vi "TC.vi"() -> ()   [LabVIEW 2013]
uses:
  lib/Lib.llb/CS.lvclass
  lib/Lib.llb/TCS.lvclass
  lib/Lib.llb/QCS.lvclass
  lib/Lib.llb/CS Emulation.lvclass
  lib/Lib.llb/PCS.lvclass
panel:
  out "Name":string
  out "SetControl":T1
  out "ControlNames":string[](array[string])
  out "VIRef":T2 {"Array DataType" format="%.0x"; "WaveForm Type" format="%.0x"; "RefNum Type" format="%.0x"; "DataType" format="%.0x"}
  out "Scan Parameters":cluster{string, "Freq":dbl, "V_exc":dbl}
  out "zConfig":path=path "C:/Users/Sasha/Dropbox/Labview/LC Software/ImpSoft-V5.2.2-multithreaded/ImpBridgeLabview/ImpBridgeDll.dll"
  out "TempStabilized":refnum<user-event>
  out "Actual I":dbl[](array[numeric])
  out "VI called?":bool=TRUE
  out "Error code":u8
  out "UpdateChannelInfo":refnum<user-event>
  out "zBridge set nr.":u8
  out "zDll":path=path "C:/Users/Sasha/Dropbox/Labview/LC Software/ImpSoft-V5.2.2-multithreaded/ImpBridgeLabview/ImpBridgeDll.dll"
  in  "String":string="^ Click the Run button to start the program "
  in  "Toolbar":enum32{"Page 1", "Page 2"}(tab)
  in  "Load config":bool
  in  "Start":bool
  in  "Load Data":bool
  in  "Pause":bool
  in  "Stop":bool
  in  "Copy to Clipboard":bool
  in  "Save to Cal Log":bool
  in  "Save config":bool
  in  "Save Data":bool
  in  "Clear all plots":bool
  in  "ColorBox":enum32{"Page 1", "Page 2"}(tab)
  in  "Colors":picture
  out "Color":u32(colorbox)
  in  "LogFileCreationTime":timestamp=timestamp(2742897600 s since 1904-01-01)
  out "UpdateLogFilePath":refnum<user-event>
  out "Calib path":path=path "C:/avs-47/aaaa"
  out "Log path":path
  out "TCS port":i32(ring)=3 items=["COM1", "COM2", "COM3", "COM4", "COM5", "COM6", "COM7", "COM8", "COM9", "PRN1", "PRN2", "PRN3", "PRN4"]
  out "UpdateCalibrations":refnum<user-event>
  out "AVS VISA session":refnum<visa-resource-name>="COM3"
  in  "Minimize 2":bool
  out "Revision":string="TC" caption="V"
  in  "Minimize":bool
  out "Current1flow":bool
  out "Current2flow":bool
  in  "Tab Control":enum32{"AVS"}(tab)
  in  "Channel Controls":T3(tab)=enum."All"
  out "T0":dbl=nan caption="T" format="%#.2p"
  out "R0":dbl caption="R" format="%.3p"
  out "R-Plot 0":cluster{dbl[], dbl[]}(graph) caption="R-Plot"
  out "T1":dbl=nan caption="T" format="%#.2p"
  out "R1":dbl caption="R" format="%.3p"
  out "R-Plot 1":cluster{dbl[], dbl[]}(graph) caption="R-Plot"
  out "T2":dbl=nan caption="T" format="%#.2p"
  out "R2":dbl caption="R" format="%.3p"
  out "R-Plot 2":cluster{dbl[], dbl[]}(graph) caption="R-Plot"
  out "T3":dbl=nan caption="T" format="%#.2p"
  out "R3":dbl caption="R" format="%.3p"
  out "R-Plot 3":cluster{dbl[], dbl[]}(graph) caption="R-Plot"
  out "T4":dbl=nan caption="T" format="%#.2p"
  out "R4":dbl caption="R" format="%.3p"
  out "R-Plot 4":cluster{dbl[], dbl[]}(graph) caption="R-Plot"
  out "T5":dbl=nan caption="T" format="%#.2p"
  out "R5":dbl caption="R" format="%.3p"
  out "R-Plot 5":cluster{dbl[], dbl[]}(graph) caption="R-Plot"
  out "T6":dbl=nan caption="T" format="%#.2p"
  out "R6":dbl caption="R" format="%.3p"
  out "R-Plot 6":cluster{dbl[], dbl[]}(graph) caption="R-Plot"
  out "T7":dbl=nan caption="T" format="%#.2p"
  out "R7":dbl caption="R" format="%.3p"
  out "R-Plot 7":cluster{dbl[], dbl[]}(graph) caption="R-Plot"
  out "T8":dbl=nan caption="T" format="%#.2p"
  out "R8":dbl caption="R" format="%.3p"
  out "R-Plot 8":cluster{dbl[], dbl[]}(graph) caption="R-Plot"
  out "T9":dbl=nan caption="T" format="%#.2p"
  out "R9":dbl caption="R" format="%.3p"
  out "R-Plot 9":cluster{dbl[], dbl[]}(graph) caption="R-Plot"
  out "T":T4 {"T0 3" format="%.2p"; "T0 2" format="%.2p"; "T0" format="%.2p"; "T0" format="%.2p"; "T0" format="%.2p"; "T0" format="%.2p"; "T0" format="%.2p"; "T0" format="%.2p"; "T0" format="%.2p"; "T0" format="%.2p"}
  in  "AVS names":T5={"AVS Name 0"="3K", "AVS Name 1"="Still", "AVS Name 2"="50 mK", "AVS Name 3"="MC", "AVS Name 4"="MC", "AVS Name 5"="", "AVS Name 6"="", "AVS Name 7"="", "AVS Name 8"="", "AVS Name 9"=""}
  in  "Edit Calibrations":T6
  in  "Thermometer":T7 {"Select sensor 10" items=["No Calibration", "PT100", "PT1000", "RuO2 10k", "RuO2 1k5", "RuO2 2k", "Emulation R", "PT 1000", "RuO2-10K-NEW", "testCMN", "No Calibration"]; "Select sensor 9" items=["No Calibration", "PT100", "PT1000", "RuO2 10k", "RuO2 1k5", "RuO2 2k", "Emulation R", "PT 1000", "RuO2-10K-NEW", "testCMN", "No Calibration"]; "Select sensor 8" items=["No Calibration", "PT100", "PT1000", "RuO2 10k", "RuO2 1k5", "RuO2 2k", "Emulation R", "PT 1000", "RuO2-10K-NEW", "testCMN", "No Calibration"]; "Select sensor 7" items=["No Calibration", "PT100", "PT1000", "RuO2 10k", "RuO2 1k5", "RuO2 2k", "Emulation R", "PT 1000", "RuO2-10K-NEW", "testCMN", "No Calibration"]; "Select sensor 6" items=["No Calibration", "PT100", "PT1000", "RuO2 10k", "RuO2 1k5", "RuO2 2k", "Emulation R", "PT 1000", "RuO2-10K-NEW", "testCMN", "No Calibration"]; "Select sensor 5" items=["No Calibration", "PT100", "PT1000", "RuO2 10k", "RuO2 1k5", "RuO2 2k", "Emulation R", "PT 1000", "RuO2-10K-NEW", "testCMN", "No Calibration"]; "Select sensor 4" items=["No Calibration", "PT100", "PT1000", "RuO2 10k", "RuO2 1k5", "RuO2 2k", "Emulation R", "PT 1000", "RuO2-10K-NEW", "testCMN", "No Calibration"]; "Select sensor 3" items=["No Calibration", "PT100", "PT1000", "RuO2 10k", "RuO2 1k5", "RuO2 2k", "Emulation R", "PT 1000", "RuO2-10K-NEW", "testCMN", "No Calibration"]; "Select sensor 2" items=["No Calibration", "PT100", "PT1000", "RuO2 10k", "RuO2 1k5", "RuO2 2k", "Emulation R", "PT 1000", "RuO2-10K-NEW", "testCMN", "No Calibration"]; "Select sensor 1" items=["No Calibration", "PT100", "PT1000", "RuO2 10k", "RuO2 1k5", "RuO2 2k", "Emulation R", "PT 1000", "RuO2-10K-NEW", "testCMN", "No Calibration"]}
  out "Units":T5
  out "R":T8={"R0"=0.0, "R1"=0.0, "R2"=-0.0, "R3"=0.0, "R4"=0.0, "R5"=0.0, "R6"=0.0, "R7"=0.0, "R6 2"=0.0, "R7 2"=0.0} {"R7 2" format="%.3p"; "R6 2" format="%.3p"; "R7" format="%.3p"; "R6" format="%.3p"; "R5" format="%.3p"; "R4" format="%.3p"; "R3" format="%.3p"; "R2" format="%.3p"; "R1" format="%.3p"; "R0" format="%.3p"}
  in  "Scan Parameters":enum32{"Page 1", "Page 2"}(tab)
  in  "Exc&Ranges":T9={"Excitationl 0"=4, "Excitationl 0"=4, "Excitationl 0"=3, "Excitationl 0"=3, "Excitationl 0"=3, "Excitationl 0"=3, "Excitationl 0"=3, "Excitationl 0"=3, "Range 0"=5, "Range 0"=5, "Range 0"=5, "Range 0"=5, "Range 0"=5, "Range 0"=5, "Range 0"=5, "Range 0"=5} {"Range 0" items=["n.a."=-1, "open"=0, "2 Ohm"=1, "20 Ohm"=2, "200 Ohm"=3, "2k Ohm"=4, "20k Ohm"=5, "200k Ohm"=6, "2M Ohm"=7]; "Range 0" items=["n.a."=-1, "open"=0, "2 Ohm"=1, "20 Ohm"=2, "200 Ohm"=3, "2k Ohm"=4, "20k Ohm"=5, "200k Ohm"=6, "2M Ohm"=7]; "Range 0" items=["n.a."=-1, "open"=0, "2 Ohm"=1, "20 Ohm"=2, "200 Ohm"=3, "2k Ohm"=4, "20k Ohm"=5, "200k Ohm"=6, "2M Ohm"=7]; "Range 0" items=["n.a."=-1, "open"=0, "2 Ohm"=1, "20 Ohm"=2, "200 Ohm"=3, "2k Ohm"=4, "20k Ohm"=5, "200k Ohm"=6, "2M Ohm"=7]; "Range 0" items=["n.a."=-1, "open"=0, "2 Ohm"=1, "20 Ohm"=2, "200 Ohm"=3, "2k Ohm"=4, "20k Ohm"=5, "200k Ohm"=6, "2M Ohm"=7]; "Range 0" items=["n.a."=-1, "open"=0, "2 Ohm"=1, "20 Ohm"=2, "200 Ohm"=3, "2k Ohm"=4, "20k Ohm"=5, "200k Ohm"=6, "2M Ohm"=7]; "Range 0" items=["n.a."=-1, "open"=0, "2 Ohm"=1, "20 Ohm"=2, "200 Ohm"=3, "2k Ohm"=4, "20k Ohm"=5, "200k Ohm"=6, "2M Ohm"=7]; "Range 0" items=["n.a."=-1, "open"=0, "2 Ohm"=1, "20 Ohm"=2, "200 Ohm"=3, "2k Ohm"=4, "20k Ohm"=5, "200k Ohm"=6, "2M Ohm"=7]; "Excitationl 0" items=["none", "3 µV", "10 µV", "30 µV", "100 µV", "300 µV", "1 mV", "3 mV"]; "Excitationl 0" items=["none", "3 µV", "10 µV", "30 µV", "100 µV", "300 µV", "1 mV", "3 mV"]; "Excitationl 0" items=["none", "3 µV", "10 µV", "30 µV", "100 µV", "300 µV", "1 mV", "3 mV"]; "Excitationl 0" items=["none", "3 µV", "10 µV", "30 µV", "100 µV", "300 µV", "1 mV", "3 mV"]; "Excitationl 0" items=["none", "3 µV", "10 µV", "30 µV", "100 µV", "300 µV", "1 mV", "3 mV"]; "Excitationl 0" items=["none", "3 µV", "10 µV", "30 µV", "100 µV", "300 µV", "1 mV", "3 mV"]; "Excitationl 0" items=["none", "3 µV", "10 µV", "30 µV", "100 µV", "300 µV", "1 mV", "3 mV"]; "Excitationl 0" items=["none", "3 µV", "10 µV", "30 µV", "100 µV", "300 µV", "1 mV", "3 mV"]}
  out "Status":T10
  out "zBridge params":T5
  out "uPlots":T11
  in  "Autorange":bool=TRUE
  out "Active":T12={"active Channel 0"=TRUE, "active Channel 1"=TRUE, "active Channel 2"=TRUE, "active Channel 3"=FALSE, "active Channel 4"=FALSE, "active Channel 5"=FALSE, "active Channel 6"=FALSE, "active Channel 7"=FALSE, "active Channel 8"=FALSE, "active Channel 9"=FALSE}
  out "PID-Plot":cluster{"Numeric":dbl, "R/T":dbl}(graph)
  in  "HW Address":u32
  in  "Edit calibration":bool
  in  "Convert":bool
  out "T7":dbl caption="T=" format="%#.2p"
  in  "QuickR":dbl caption="R=" format="%_6g"
  in  "Select sensor 1":u16(ring) items=["No Calibration", "PT100", "PT1000", "RuO2 10k", "RuO2 1k5", "RuO2 2k", "Emulation R", "PT 1000", "RuO2-10K-NEW", "testCMN", "No Calibration"]
  out "I_list[i]":dbl[](array[numeric]) min=-1.0
  out "I_in":dbl[](array[numeric]) min=-1.0
  in  "Tab Control 5":enum32{"Page 1", "Page 2"}(tab)
  in  "Data History":enum32{"History", "Settings"}(tab)=enum."Settings"
  in  "Mode Buttons":T13(radio)
  in  "Erase All":bool
  out "AVS names small":T5={"AVS Name 0"="3K", "AVS Name 1"="Still", "AVS Name 2"="50 mK", "AVS Name 3"="MC", "AVS Name 4"="MC", "AVS Name 5"="", "AVS Name 6"="", "AVS Name 7"="", "AVS Name 8"="", "AVS Name 9"=""}
  out "Active channel":T14
  out "Small T":T15 caption="T" {"R1" format="%#.2p"; "R1" format="%#.2p"; "R1" format="%#.2p"; "R1" format="%#.2p"; "R1" format="%#.2p"; "R1" format="%#.2p"; "R1" format="%#.2p"; "R1" format="%#.2p"; "R1" format="%#.2p"; "R1" format="%#.2p"}
  out "Small R":T16 caption="R" {"R1 2" format="%#_5p"; "R1 2" format="%#_5p"; "R1 2" format="%#_5p"; "R1 2" format="%#_5p"; "R1 2" format="%#_5p"; "R1 2" format="%#_5p"; "R1 2" format="%#_5p"; "R1 2" format="%#_5p"; "R1 2" format="%#_5p"; "R1 2" format="%#_5p"}
  out "Time":dbl format="%<%X\n%x>T"
  in  "AVS Runtime Settings":T17={"Read AVS channels from"=0, "Last Channel"=7, "Delay Between Scans"=0, "Stabilisation Delay"=0.5, "Averages"=2, "Data Memory"=5000, "Filter graphs:"=FALSE, "Y_min"=0.0, "Y_max"=2000000.0, "Plot type"=enum."T vs Time", "Allow neg R"=TRUE, "Data Memory 2"=30.0} {"Data Memory 2" min=0.0; "Delay Between Scans" format="%.0f s"; "Averages" min=1 max=1000; "Stabilisation Delay" min=0.5; "Last Channel" min=0 max=7 step=1; "Read AVS channels from" min=0 max=7 step=1; "Y_max" format="%#_6f"; "Y_min" min=0.0 format="%#_6f"; "Data Memory" min=3 max=30000}
  out "I":dbl[](array[numeric])
  in  "Data":cluster{"R":dbl[], "T":dbl[], "Time":dbl[]}[](array[cluster])=[{"R"=[], "T"=[], "Time"=[]}, {"R"=[0.0, 2.0], "T"=[], "Time"=[]}]
  out "Int":dbl=10.0 format="%#.2f"
  out "T_array":dbl[](array[numeric])
  in  "Data array":dbl[](array[numeric])
  out "I3_SetPnt":dbl
  out "Currents changed":bool
  in  "Excitations":T18={"Excitationl 0"=4, "Excitation 1"=4, "Excitation 2"=3, "Excitation 3"=3, "Excitation 4"=3, "Excitation 5"=3, "Excitation 6"=3, "Excitation 7"=3} {"Excitation 7" items=["none", "3 µV", "10 µV", "30 µV", "100 µV", "300 µV", "1 mV", "3 mV"]; "Excitation 6" items=["none", "3 µV", "10 µV", "30 µV", "100 µV", "300 µV", "1 mV", "3 mV"]; "Excitation 5" items=["none", "3 µV", "10 µV", "30 µV", "100 µV", "300 µV", "1 mV", "3 mV"]; "Excitation 4" items=["none", "3 µV", "10 µV", "30 µV", "100 µV", "300 µV", "1 mV", "3 mV"]; "Excitation 3" items=["none", "3 µV", "10 µV", "30 µV", "100 µV", "300 µV", "1 mV", "3 mV"]; "Excitation 2" items=["none", "3 µV", "10 µV", "30 µV", "100 µV", "300 µV", "1 mV", "3 mV"]; "Excitation 1" items=["none", "3 µV", "10 µV", "30 µV", "100 µV", "300 µV", "1 mV", "3 mV"]; "Excitationl 0" items=["none", "3 µV", "10 µV", "30 µV", "100 µV", "300 µV", "1 mV", "3 mV"]}
  in  "Ranges":T18={"Excitationl 0"=5, "Excitation 1"=5, "Excitation 2"=5, "Excitation 3"=5, "Excitation 4"=5, "Excitation 5"=5, "Excitation 6"=5, "Excitation 7"=5} {"Excitation 7" items=["n.a."=-1, "open"=0, "2 Ohm"=1, "20 Ohm"=2, "200 Ohm"=3, "2k Ohm"=4, "20k Ohm"=5, "200k Ohm"=6, "2M Ohm"=7]; "Excitation 6" items=["n.a."=-1, "open"=0, "2 Ohm"=1, "20 Ohm"=2, "200 Ohm"=3, "2k Ohm"=4, "20k Ohm"=5, "200k Ohm"=6, "2M Ohm"=7]; "Excitation 5" items=["n.a."=-1, "open"=0, "2 Ohm"=1, "20 Ohm"=2, "200 Ohm"=3, "2k Ohm"=4, "20k Ohm"=5, "200k Ohm"=6, "2M Ohm"=7]; "Excitation 4" items=["n.a."=-1, "open"=0, "2 Ohm"=1, "20 Ohm"=2, "200 Ohm"=3, "2k Ohm"=4, "20k Ohm"=5, "200k Ohm"=6, "2M Ohm"=7]; "Excitation 3" items=["n.a."=-1, "open"=0, "2 Ohm"=1, "20 Ohm"=2, "200 Ohm"=3, "2k Ohm"=4, "20k Ohm"=5, "200k Ohm"=6, "2M Ohm"=7]; "Excitation 2" items=["n.a."=-1, "open"=0, "2 Ohm"=1, "20 Ohm"=2, "200 Ohm"=3, "2k Ohm"=4, "20k Ohm"=5, "200k Ohm"=6, "2M Ohm"=7]; "Excitation 1" items=["n.a."=-1, "open"=0, "2 Ohm"=1, "20 Ohm"=2, "200 Ohm"=3, "2k Ohm"=4, "20k Ohm"=5, "200k Ohm"=6, "2M Ohm"=7]; "Excitationl 0" items=["n.a."=-1, "open"=0, "2 Ohm"=1, "20 Ohm"=2, "200 Ohm"=3, "2k Ohm"=4, "20k Ohm"=5, "200k Ohm"=6, "2M Ohm"=7]}
  out "CS ref":refnum<class "CS.lvclass">
  out "start 2":bool
  in  "Current indicators":enum32{"Page 1", "Page 2"}(tab)
  out "Automatic mode 0":bool
  out "Automatic mode 1":bool
  out "Map Channel 0 to 2":T19(ring) caption="Output to"
  in  "uA 0":u32
  in  "CS Names":T20={"CS Name 0"="N.C.", "CS Name 1"="3K", "CS Name 2"="Still", "CS Name 3"="MC"}
  out "I0":T21={"uA"="000", "ON"=FALSE, "Gated"=FALSE, "current flows"=FALSE, "Error"=FALSE} caption="Ch0 -"
  in  "uA 3":u32
  in  "uA 2":u32
  in  "uA 1":u32
  out "Automatic mode 3":bool
  out "Automatic mode 2":bool
  out "I3":T21={"uA"="000", "ON"=FALSE, "Gated"=FALSE, "current flows"=FALSE, "Error"=FALSE} caption="Chn 3"
  out "I2":T21={"uA"="000", "ON"=FALSE, "Gated"=FALSE, "current flows"=FALSE, "Error"=FALSE} caption="Chn 2"
  out "I1":T21={"uA"="000", "ON"=FALSE, "Gated"=FALSE, "current flows"=FALSE, "Error"=FALSE} caption="Chn 1"
  out "I_0":dbl=10.0
  out "vi reference":refnum<vi>
  in  "Show PID graph?":bool
  in  "Set Color":bool
  in  "Save Screen Data":bool
  in  "CS Ch3 mode":enum32{"Page 1", "Page 2"}(tab)=enum."Page 2"
  in  "T Sweep":T22={"Start value"=200.0, "End value"=250.0, "Step"=10.0, "Current"=0.0, "I_next"=FALSE, "I_prev"=FALSE, "Interrrupt Sweep"=FALSE, "Start"=FALSE, "Boolean"=TRUE} {"Step" min=0.0; "End value" min=0.0; "Start value" min=0.0}
  out "CallExtVI":refnum<user-event>
  out "Unit":string
  out "UpdateValuesAVS":refnum<user-event>
  out "DoPID":refnum<user-event>
  out "UpdateValuesZBridge":refnum<user-event>
  out "zBridge params/Error":string
  out "CurCalibrations":T23
  out "LMB Down":bool
  out "T controlled":dbl
  out "ResetPIDloop":refnum<user-event>
  in  "Tab Control 2":T24(tab)=enum."Current source control"
  in  "Refresh Calibrations":bool
  in  "Save Screen Data 2":bool
  out "ID":string
  out "Bridge status":errorcluster
  out "CS status":errorcluster
  out "General":errorcluster caption="General status"
  in  "Bridge settings":T25={"AVS type"=enum."AVS47A (GPIB interface)", "AVS_SPort"="COM5", "Address"="GPIB0::20::INSTR", "AVS_CalFolder"=path "E:/Dropbox/Labview/LC Software/All Calibrations"}
  in  "Current source settings":T26={"TCS_Port"="COM1", "TCS_Imax"=5, "CS type"=enum."TCS", "QCS/PCS Device"=0}
  in  "Data logging":T27={"AVS_Path"=path "C:/avs-47", "AVS_FName"="LogAVS", "CAL_FName"="calibration", "Filenames suffix"="_%Y-%m-%d-%H-%M-%S", "Delimeter"="\t", "NewFevery"=7, "Time Units"=enum."Days", "Date/Time Format"="%Y-%m-%d %H:%M:%S", "External VI path"=path "C:/Users/User1/Dropbox/Labview/LC Software/TempControl/OnTempStabilized Ext VI Laurens.vi", "VI state:"=enum."Bad", "Ask on start?"=FALSE, "Run description"="\n"}
  in  "I_list":dbl[][](array[numeric]) min=-1.0
  out "T Channel":bool[](array[boolean])
  in  "Trigger other running TC instances":bool
  in  "I_Clear":bool
  in  "I3 as temp":cluster{"I3 as temp 2":bool}
  in  "C_I3":T28={"Toggle ON/OFF"=FALSE, "Toggle Gated"=FALSE, "I"=0, "Range"=enum."x1 uA"} caption="I3" {"I" max=100000 step=1}
  in  "C_I2":T28={"Toggle ON/OFF"=FALSE, "Toggle Gated"=FALSE, "I"=0, "Range"=enum."x1 uA"} caption="I2" {"I" max=100000 step=1}
  in  "C_I1":T28={"Toggle ON/OFF"=FALSE, "Toggle Gated"=FALSE, "I"=0, "Range"=enum."x1 uA"} caption="I1" {"I" max=100000 step=1}
  in  "C_I0":T28={"Toggle ON/OFF"=FALSE, "Toggle Gated"=FALSE, "I"=0, "Range"=enum."x1 uA"} caption="I0" {"I" max=100000 step=1}
  in  "I0 output to":T29(ring) caption="Set QCS Channel 0 output to"
  in  "CS Mode":enum16{"Manual", "Automatic"}(ring) caption="CS control mode"
  in  "Write to log":bool
  in  "Load from file":bool
  in  "Save to file":bool
  in  "I_tofirst":bool
  in  "I_next":bool
  in  "I_prev":bool
  out "VI state:":T30(ring)
  out "I_selection":bool[](array[boolean])=[TRUE, FALSE, FALSE, FALSE, FALSE, FALSE, FALSE, FALSE, FALSE, FALSE]
  in  "Call external VI":bool
  out "Time Old":dbl format="%#_16g"
  in  "Automode Settings 2":T31={"AVS Channel"=0, "N averages"=10, "Delay Time"=10.0, "T stability"=0.3, "FB on"=enum."Temperature"} {"Delay Time" min=0.0 format="%#_g min"; "AVS Channel" min=-1 max=9 step=1}
  in  "Automode 2":bool=TRUE caption="Enable automatic sweeping/list iteration"
  in  "PID setup 2":T32={"Current limit, [uA]"=10000.0, "Proportional Gain"=3.0, "Integral Gain"=3.0, "Derivative Gain"=1.0, "SP tolerance"=0.1, "Feed Fwd Gain [uA/mK]"=0.0, "Integral Gain Bandwidth"=10.0, "Integral Gain Background"=1.0, "FB on 2"=enum."1"} {"Integral Gain Background" format="%#.6g"; "Integral Gain Bandwidth" format="%#.6g"; "Feed Fwd Gain [uA/mK]" format="%#.5g"; "SP tolerance" format="%#.5g"; "Derivative Gain" format="%#.6g"; "Integral Gain" format="%#.6g"; "Proportional Gain" format="%#.6g"; "Current limit, [uA]" format="%#.5g"}
  in  "Reset PID":bool
  in  "Next step":bool
  out "I_list_idx":i32=10 caption="Point #"
  out "I_list_idx_max":i32=10 caption="of"
  out "Timer":dbl format="%<%H:%M:%S>t"
  out "Slope":dbl format="%#_3g %"
  out "Error":dbl=10.0 format="%#_6f"
  out "SP reached?":bool
  # "Quick convert R->T:"
  # "Ohm"
  # "mK"
  # "Ch#"
  # "Miniplot"
  # "Channel parameters"
  # "Impedance"
  # "Unit"
  # "Type of sensor"
  # "T [mK]"
  # "Description"
  # "0"
  # "1"
  # "2"
  # "3"
  # "4"
  # "5"
  # "6"
  # "7"
  # "8"
  # "9"
  # "0"
  # "1"
  # "2"
  # "3"
  # "4"
  # "5"
  # "7"
  # "8"
  # "9"
  # "6"
  # "auto"
  # "auto"
  # "auto"
  # "auto"
  # "gated"
  # "gated"
  # "gated"
  # "gated"
  # "Ch3"
  # "Current source mode"
  # "Current source manual control"
  # "Automatic mode or current source"
  # "Currents List"
  # "Settings"
  # "I0"
  # "I1"
  # "I2"
  # "I3"
  # "Status"
  # "On temperature stabilized"
types:
  T1 = cluster{"Name":string, "Scalar":string, "Array":string[][]}
  T2 = cluster{"Control Ref ID":refnum<vi>[], "Full Name":string[], "ClassID":enum16{"<Null>", "1", "2", "Generic", "Decoration", "Text", "Control", "ColorBox", "Boolean", "RefNum", "Variant", "Path", "ListBox", "Table", "Array", "Picture", "ActiveXContainer", "Numeric", "Digital", "NamedNumeric", "ColorRamp", "Slide", "GraphOrChart", "WaveformChart", "WaveformGraph", "IntensityChart", "IntensityGraph", "String", "IOName", "ComboBox", "Cluster", "Panel", "Knob", "NumWithScale", "Ring", "Enum", "GObject", "Plot", "Cursor", "NumericText", "Scale", "ColorScale", "GraphScale", "ColorGraphScale", "TypedRefNum", "OldKnobScale", "MCListbox", "MeasureData", "BVTag", "DAQName", "VISAName", "IVIName", "SlideScale", "TabControl", "Page", "TabArrayTabControl", "ConPane", "57", "58", "59", "60", "61", "62", "63", "64", "SubPanel", "TreeControl", "67", "68", "69", "70", "71", "72", "73", "74", "75", "SplitterBar"}[], "Short Name":string[], "DataType":enum8{"<Null>", "I8", "I16", "I32", "I64", "U8", "U16", "U32", "U64", "SGL", "DBL", "EXT", "CSG", "CDB", "CXT", "0x0F", "0x10", "0x11", "0x12", "0x13", "0x14", "Enum U8", "Enum U16", "Enum U32", "Enum U64", "SGL PQ", "DBL PQ", "EXT PQ", "CSG PQ", "CDB PQ", "CXT PQ", "0x1F", "0x20", "Boolean", "0x22", "0x23", "0x24", "0x25", "0x26", "0x27", "0x28", "0x29", "0x2A", "0x2B", "0x2C", "0x2D", "0x2E", "0x2F", "String", "0x31", "Path", "Pict", "0x34", "0x35", "0x36", "DAQ", "0x38", "0x39", "0x3A", "0x3B", "0x3C", "0x3D", "0x3E", "0x3F", "Array", "0x41", "0x42", "0x43", "0x44", "0x45", "0x46", "0x47", "0x48", "0x49", "0x4A", "0x4B", "0x4C", "0x4D", "0x4E", "0x4F", "Cluster", "0x51", "0x52", "Variant", "Waveform", "0x55", "0x56", "0x57", "0x58", "0x59", "0x5A", "0x5B", "0x5C", "0x5D", "0x5E", "0x5F", "0x60", "0x61", "0x62", "0x63", "0x64", "0x65", "0x66", "0x67", "0x68", "0x69", "0x6A", "0x6B", "0x6C", "0x6D", "0x6E", "0x6F", "Refnum"}[], "RefNum Type":enum8{"Generic", "Datalog File Refnum", "Byte Stream File Refnum", "Device Refnum", "Occurence Refnum", "TCP Connection Refnum", "VISA Refnum (Obsolete)", "Automation Renum", "VI Server Refnum", "Menu Refnum", "IVI Refnum (Obsolete)", "IMAQ Session", "0x0C", "Datasocket Refnum", "VISA Resource", "IVI Logical Name", "UDP Connection Refnum", "Notifier Refnum", "Queue Refnum", "IrDA Refnum", "Hardware Plugin Refnum", "Hardware Plugin Tag Refnum", "DAQmx Refnum", "Event Registration Refnum", ".NET Refnum", "User Event Refnum", "0x1A", "Event Callback", "0x1C", "0x1D", "Only Used Internal to LabVIEW", "Bluetooth", "Data Value References", "RT FIFO", "TDM Streaming"}[], "WaveForm Type":enum8{"<Not a Waveform Type>", "0x01", "Analog 16-bit signed", "Analog Double-Precision", "0x04", "Analog Single Precision", "Timestamp", "Digital Data", "Digital Waveform", "Dynamic Data", "Analog Extended-Precision", "Analog 8-bit unsigned", "Analog 16-bit unsigned", "Analog 32-bit unsigned", "Analog 8-bit signed", "Analog 32-bit signed", "Analog Complex Single-Precision", "Analog Complex Double-Precision", "Analog Complex Extended Precision", "Analog 64-bit signed", "Analog 64-bit unsigned"}[], "Parent":i32[], "Array DataType":enum8{"<Null>", "I8", "I16", "I32", "I64", "U8", "U16", "U32", "U64", "SGL", "DBL", "EXT", "CSG", "CDB", "CXT", "0x0F", "0x10", "0x11", "0x12", "0x13", "0x14", "Enum U8", "Enum U16", "Enum U32", "Enum U64", "SGL PQ", "DBL PQ", "EXT PQ", "CSG PQ", "CDB PQ", "CXT PQ", "0x1F", "0x20", "Boolean", "0x22", "0x23", "0x24", "0x25", "0x26", "0x27", "0x28", "0x29", "0x2A", "0x2B", "0x2C", "0x2D", "0x2E", "0x2F", "String", "0x31", "Path", "Pict", "0x34", "0x35", "0x36", "DAQ", "0x38", "0x39", "0x3A", "0x3B", "0x3C", "0x3D", "0x3E", "0x3F", "Array", "0x41", "0x42", "0x43", "0x44", "0x45", "0x46", "0x47", "0x48", "0x49", "0x4A", "0x4B", "0x4C", "0x4D", "0x4E", "0x4F", "Cluster", "0x51", "0x52", "Variant", "Waveform", "0x55", "0x56", "0x57", "0x58", "0x59", "0x5A", "0x5B", "0x5C", "0x5D", "0x5E", "0x5F", "0x60", "0x61", "0x62", "0x63", "0x64", "0x65", "0x66", "0x67", "0x68", "0x69", "0x6A", "0x6B", "0x6C", "0x6D", "0x6E", "0x6F", "Refnum"}[], "Owning VI":refnum<vi>[], "Active?":bool[]}
  T3 = enum32{"0", "1", "2", "3", "4", "5", "6", "7", "8", "9", "All", "PID loop"}
  T4 = cluster{"T0":dbl, "T0":dbl, "T0":dbl, "T0":dbl, "T0":dbl, "T0":dbl, "T0":dbl, "T0":dbl, "T0 2":dbl, "T0 3":dbl}
  T5 = cluster{"AVS Name 0":string, "AVS Name 1":string, "AVS Name 2":string, "AVS Name 3":string, "AVS Name 4":string, "AVS Name 5":string, "AVS Name 6":string, "AVS Name 7":string, "AVS Name 8":string, "AVS Name 9":string}
  T6 = cluster{"Boolean":bool, "Boolean 2":bool, "Boolean 3":bool, "Boolean 4":bool, "Boolean 5":bool, "Boolean 6":bool, "Boolean 7":bool, "Boolean 8":bool, "Boolean 9":bool, "Boolean 10":bool}
  T7 = cluster{"Select sensor 1":u16, "Select sensor 2":u16, "Select sensor 3":u16, "Select sensor 4":u16, "Select sensor 5":u16, "Select sensor 6":u16, "Select sensor 7":u16, "Select sensor 8":u16, "Select sensor 9":u16, "Select sensor 10":u16}
  T8 = cluster{"R0":dbl, "R1":dbl, "R2":dbl, "R3":dbl, "R4":dbl, "R5":dbl, "R6":dbl, "R7":dbl, "R6 2":dbl, "R7 2":dbl}
  T9 = cluster{"Excitationl 0":i16, "Excitationl 0":i16, "Excitationl 0":i16, "Excitationl 0":i16, "Excitationl 0":i16, "Excitationl 0":i16, "Excitationl 0":i16, "Excitationl 0":i16, "Range 0":i16, "Range 0":i16, "Range 0":i16, "Range 0":i16, "Range 0":i16, "Range 0":i16, "Range 0":i16, "Range 0":i16}
  T10 = cluster{"Numeric":dbl, "Numeric":dbl, "Numeric":dbl, "Numeric":dbl, "Numeric":dbl, "Numeric":dbl, "Numeric":dbl, "Numeric":dbl, "Numeric":dbl, "Numeric":dbl}
  T11 = cluster{"uPlot 0":cluster{dbl[], dbl[]}, "uPlot 1":cluster{dbl[], dbl[]}, "uPlot 2":cluster{dbl[], dbl[]}, "uPlot 3":cluster{dbl[], dbl[]}, "uPlot 4":cluster{dbl[], dbl[]}, "uPlot 5":cluster{dbl[], dbl[]}, "uPlot 6":cluster{dbl[], dbl[]}, "uPlot 7":cluster{dbl[], dbl[]}, "uPlot 8":cluster{dbl[], dbl[]}, "uPlot 9":cluster{dbl[], dbl[]}}
  T12 = cluster{"active Channel 0":bool, "active Channel 1":bool, "active Channel 2":bool, "active Channel 3":bool, "active Channel 4":bool, "active Channel 5":bool, "active Channel 6":bool, "active Channel 7":bool, "active Channel 8":bool, "active Channel 9":bool}
  T13 = enum32{"No Selection", "Cursor Mode", "Erase point", "Erase Range"}
  T14 = cluster{"Boolean 5":bool, "Boolean 5":bool, "Boolean 5":bool, "Boolean 5":bool, "Boolean 5":bool, "Boolean 5":bool, "Boolean 5":bool, "Boolean 5":bool, "Boolean 5":bool, "Boolean 5":bool}
  T15 = cluster{"R1":dbl, "R1":dbl, "R1":dbl, "R1":dbl, "R1":dbl, "R1":dbl, "R1":dbl, "R1":dbl, "R1":dbl, "R1":dbl}
  T16 = cluster{"R1 2":dbl, "R1 2":dbl, "R1 2":dbl, "R1 2":dbl, "R1 2":dbl, "R1 2":dbl, "R1 2":dbl, "R1 2":dbl, "R1 2":dbl, "R1 2":dbl}
  T17 = cluster{"Read AVS channels from":i8, "Last Channel":i8, "Delay Between Scans":u32, "Stabilisation Delay":dbl, "Averages":u16, "Data Memory":u16, "Filter graphs:":bool, "Y_min":dbl, "Y_max":dbl, "Plot type":enum16{"R vs Time", "T vs Time"}, "Allow neg R":bool, "Data Memory 2":dbl}
  T18 = cluster{"Excitationl 0":i16, "Excitation 1":i16, "Excitation 2":i16, "Excitation 3":i16, "Excitation 4":i16, "Excitation 5":i16, "Excitation 6":i16, "Excitation 7":i16}
  T19 = enum16{"Chn 0", "Aux 0", "Aux 1", "Aux 2", "Aux 3"}
  T20 = cluster{"CS Name 0":string, "CS Name 1":string, "CS Name 2":string, "CS Name 3":string}
  T21 = cluster{"uA":string, "ON":bool, "Gated":bool, "current flows":bool, "Error":bool}
  T22 = cluster{"Start value":dbl, "End value":dbl, "Step":dbl, "Current":dbl, "I_next":bool, "I_prev":bool, "Interrrupt Sweep":bool, "Start":bool, "Boolean":bool}
  T23 = cluster{"[0]":string, "[1]":string, "[2]":string, "[3]":string, "[4]":string, "[5]":string, "[6]":string, "[7]":string, "[8]":string, "[9]":string}
  T24 = enum32{"Devices Settings", "Current source control"}
  T25 = cluster{"AVS type":enum16{"AVS47A (GPIB interface)", "AVS47B (RS232 interface)", "AVS48", "AVS Emulation", "Impedance Bridge", "Disabled"}, "AVS_SPort":refnum<visa-resource-name>, "Address":refnum<visa-resource-name>, "AVS_CalFolder":path}
  T26 = cluster{"TCS_Port":refnum<visa-resource-name>, "TCS_Imax":i32, "CS type":enum16{"TCS", "QCS v1", "PCS (n.a.)", "CS Emulation", "Disabled"}, "QCS/PCS Device":u16}
  T27 = cluster{"AVS_Path":path, "AVS_FName":string, "CAL_FName":string, "Filenames suffix":string, "Delimeter":string, "NewFevery":u32, "Time Units":enum16{"Minutes", "Hours", "Days"}, "Date/Time Format":string, "External VI path":path, "VI state:":enum32{"Bad", "Idle", "Run top level", "Running"}, "Ask on start?":bool, "Run description":string}
  T28 = cluster{"Toggle ON/OFF":bool, "Toggle Gated":bool, "I":u32, "Range":enum8{"Auto", "x1 uA", "x10 uA", "x100 uA", "x1 mA"}}
  T29 = enum16{"Channel 0", "Aux 0", "Aux 1", "Aux 2", "Aux 3"}
  T30 = enum32{"Bad", "Idle", "Run top level", "Running"}
  T31 = cluster{"AVS Channel":i32, "N averages":i32, "Delay Time":dbl, "T stability":dbl, "FB on":enum16{"Resistance", "Temperature"}}
  T32 = cluster{"Current limit, [uA]":dbl, "Proportional Gain":dbl, "Integral Gain":dbl, "Derivative Gain":dbl, "SP tolerance":dbl, "Feed Fwd Gain [uA/mK]":dbl, "Integral Gain Bandwidth":dbl, "Integral Gain Background":dbl, "FB on 2":enum16{"0", "1", "2", "3"}}
  T33 = cluster{"error":bool, "code":i32, "source":string}
  T34 = enum32{"No Selection", "Erase Data", "Erase Range", "Cursor Mode"}
  T35 = enum16{"AVS47A (GPIB interface)", "AVS47B (RS232 interface)", "AVS48", "AVS Emulation", "Impedance Bridge", "Disabled"}
  T36 = enum16{"TCS", "QCS v1", "PCS (n.a.)", "CS Emulation", "Disabled"}
  T37 = enum8{"Auto", "x1 uA", "x10 uA", "x100 uA", "x1 mA"}
  T38 = cluster{"Cluster":cluster{"Time":dbl[], "T":dbl[]}, "Cluster":cluster{"Time":dbl[], "T":dbl[]}, "Cluster":cluster{"Time":dbl[], "T":dbl[]}, "Cluster":cluster{"Time":dbl[], "T":dbl[]}, "Cluster":cluster{"Time":dbl[], "T":dbl[]}, "Cluster":cluster{"Time":dbl[], "T":dbl[]}, "Cluster":cluster{"Time":dbl[], "T":dbl[]}, "Cluster":cluster{"Time":dbl[], "T":dbl[]}, "Cluster":cluster{"Time":dbl[], "T":dbl[]}, "Cluster":cluster{"Time":dbl[], "T":dbl[]}}
  T39 = enum32{"HKEY_CLASSES_ROOT", "HKEY_CURRENT_USER", "HKEY_LOCAL_MACHINE", "HKEY_USERS", "HKEY_PERFORMANCE_DATA", "HKEY_CURRENT_CONFIG", "HKEY_DYN_DATA"}
  T40 = enum32{"invalid app kind", "Development System", "Run Time System", "Student Edition", "Embedded LabVIEW", "Evaluation", "Custom"}
  T41 = cluster{"[0]":dbl, "[1]":dbl, "[2]":dbl, "[3]":dbl, "[4]":dbl, "[5]":dbl, "[6]":dbl, "[7]":dbl, "[8]":dbl, "[9]":dbl}
  T42 = cluster{"Temperature[0]":dbl, "Temperature[1]":dbl, "Temperature[2]":dbl, "Temperature[3]":dbl, "Temperature[4]":dbl, "Temperature[5]":dbl, "Temperature[6]":dbl, "Temperature[7]":dbl, "Temperature[8]":dbl, "Temperature[9]":dbl}
  T43 = cluster{"type":string, "creator":string, "permissions":i32, "data size":i32, "res size":i32, "creation date":u32, "modification date":u32, "bFolder":bool, "bInvisible":bool, "location":cluster{"vertical":i16, "horizontal":i16}, "owner":string, "group":string}
  T44 = enum16{"CF", "CF_Z_Bridge", "MNK", "MNK_Z_Bridge"}
  T45 = cluster{"Units[0]":string, "Units[1]":string, "Units[2]":string, "Units[3]":string, "Units[4]":string, "Units[5]":string, "Units[6]":string, "Units[7]":string, "Units[8]":string, "Units[9]":string}
  T46 = cluster{"zBridge params[0]":string, "zBridge params[1]":string, "zBridge params[2]":string, "zBridge params[3]":string, "zBridge params[4]":string, "zBridge params[5]":string, "zBridge params[6]":string, "zBridge params[7]":string, "zBridge params[8]":string, "zBridge params[9]":string}
  T47 = cluster{"date/time string":string, "Value":dbl[], "Value":dbl[], "Value":dbl[]}
  T48 = typedef "imagedata.ctl" = cluster{"image type":i32, "image depth":i32, "image":u8[], "mask":u8[], "colors":u32[], "Rectangle":cluster{"left":i16, "top":i16, "right":i16, "bottom":i16}}
  T49 = typedef "LVPoint32TypeDef.ctl" = cluster{"Horizontal":i32, "Vertical":i32}
  T50 = cluster{"Output Array":dbl[], "array w/ subset deleted":dbl[], "array w/ subset deleted":dbl[]}
  T51 = typedef "LVRectTypeDef.ctl" = cluster{"Left":i16, "Top":i16, "Right":i16, "Bottom":i16}
  T52 = cluster{"Excitationl 0":i16, "Excitation 1":i16, "Excitation 2":i16, "Excitation 3":i16, "Excitation 4":i16, "Excitation 5":i16, "Excitation 6":i16, "Excitation 7":i16, "Range 0":i16, "Range 1":i16, "Range 2":i16, "Range 3":i16, "Range 4":i16, "Range 5":i16, "Range 6":i16, "Range 7":i16}
  T53 = enum8{"Active", "Channel Type", "Channel No", "Reference No", "RLC select", "Save Data", "L Inverted", "Menu Active"}
  T54 = typedef "LVPositionTypeDef.ctl" = cluster{"Left":i32, "Top":i32}
  T55 = cluster{"Range 0":i16, "Range 1":i16, "Range 2":i16, "Range 3":i16, "Range 4":i16, "Range 7":i16, "Range 5":i16, "Range 6":i16}
  T56 = cluster{"Range 0":i16, "Range 1":i16, "Range 2":i16, "Range 3":i16, "Range 4":i16, "Range 5":i16, "Range 6":i16, "Range 7":i16}
  T57 = cluster{"RANGE 0":u16, "RANGE 1":u16, "RANGE 2":u16, "RANGE 3":u16, "RANGE 4":u16, "RANGE 5":u16, "RANGE 6":u16, "RANGE 7":u16}
  T58 = cluster{"Range":u8, "Current":dbl, "Current (string)":string, "On?":bool, "G?":bool, "I?":bool, "Err?":bool}
  T59 = cluster{"uA":string, " ON":bool, "Gated":bool, "current flows":bool, "Error":bool}
  T60 = cluster{"Toggle ON/OFF":bool, "Toggle Gated":bool}
  T61 = cluster{"Current":u32, "Range":enum16{"Auto", "x1 uA", "x10 uA", "x100 uA", "x1 mA"}}
  T62 = cluster{"Toggle ON/OFF":bool, "Toggle Gated":bool, "Current":u32, "Range":enum8{"Auto", "x1 uA", "x10 uA", "x100 uA", "x1 mA"}}
  T63 = cluster{"Status[0]":i32, "Status[1]":i32, "Status[2]":i32, "Status[3]":i32, "Status[4]":i32, "Status[5]":i32, "Status[6]":i32, "Status[7]":i32, "Status[8]":i32, "Status[9]":i32}
  T64 = cluster{"Active":bool, "Active":bool, "Active":bool, "Active":bool, "Active":bool, "Active":bool, "Active":bool, "Active":bool, "Active":bool, "Active":bool}
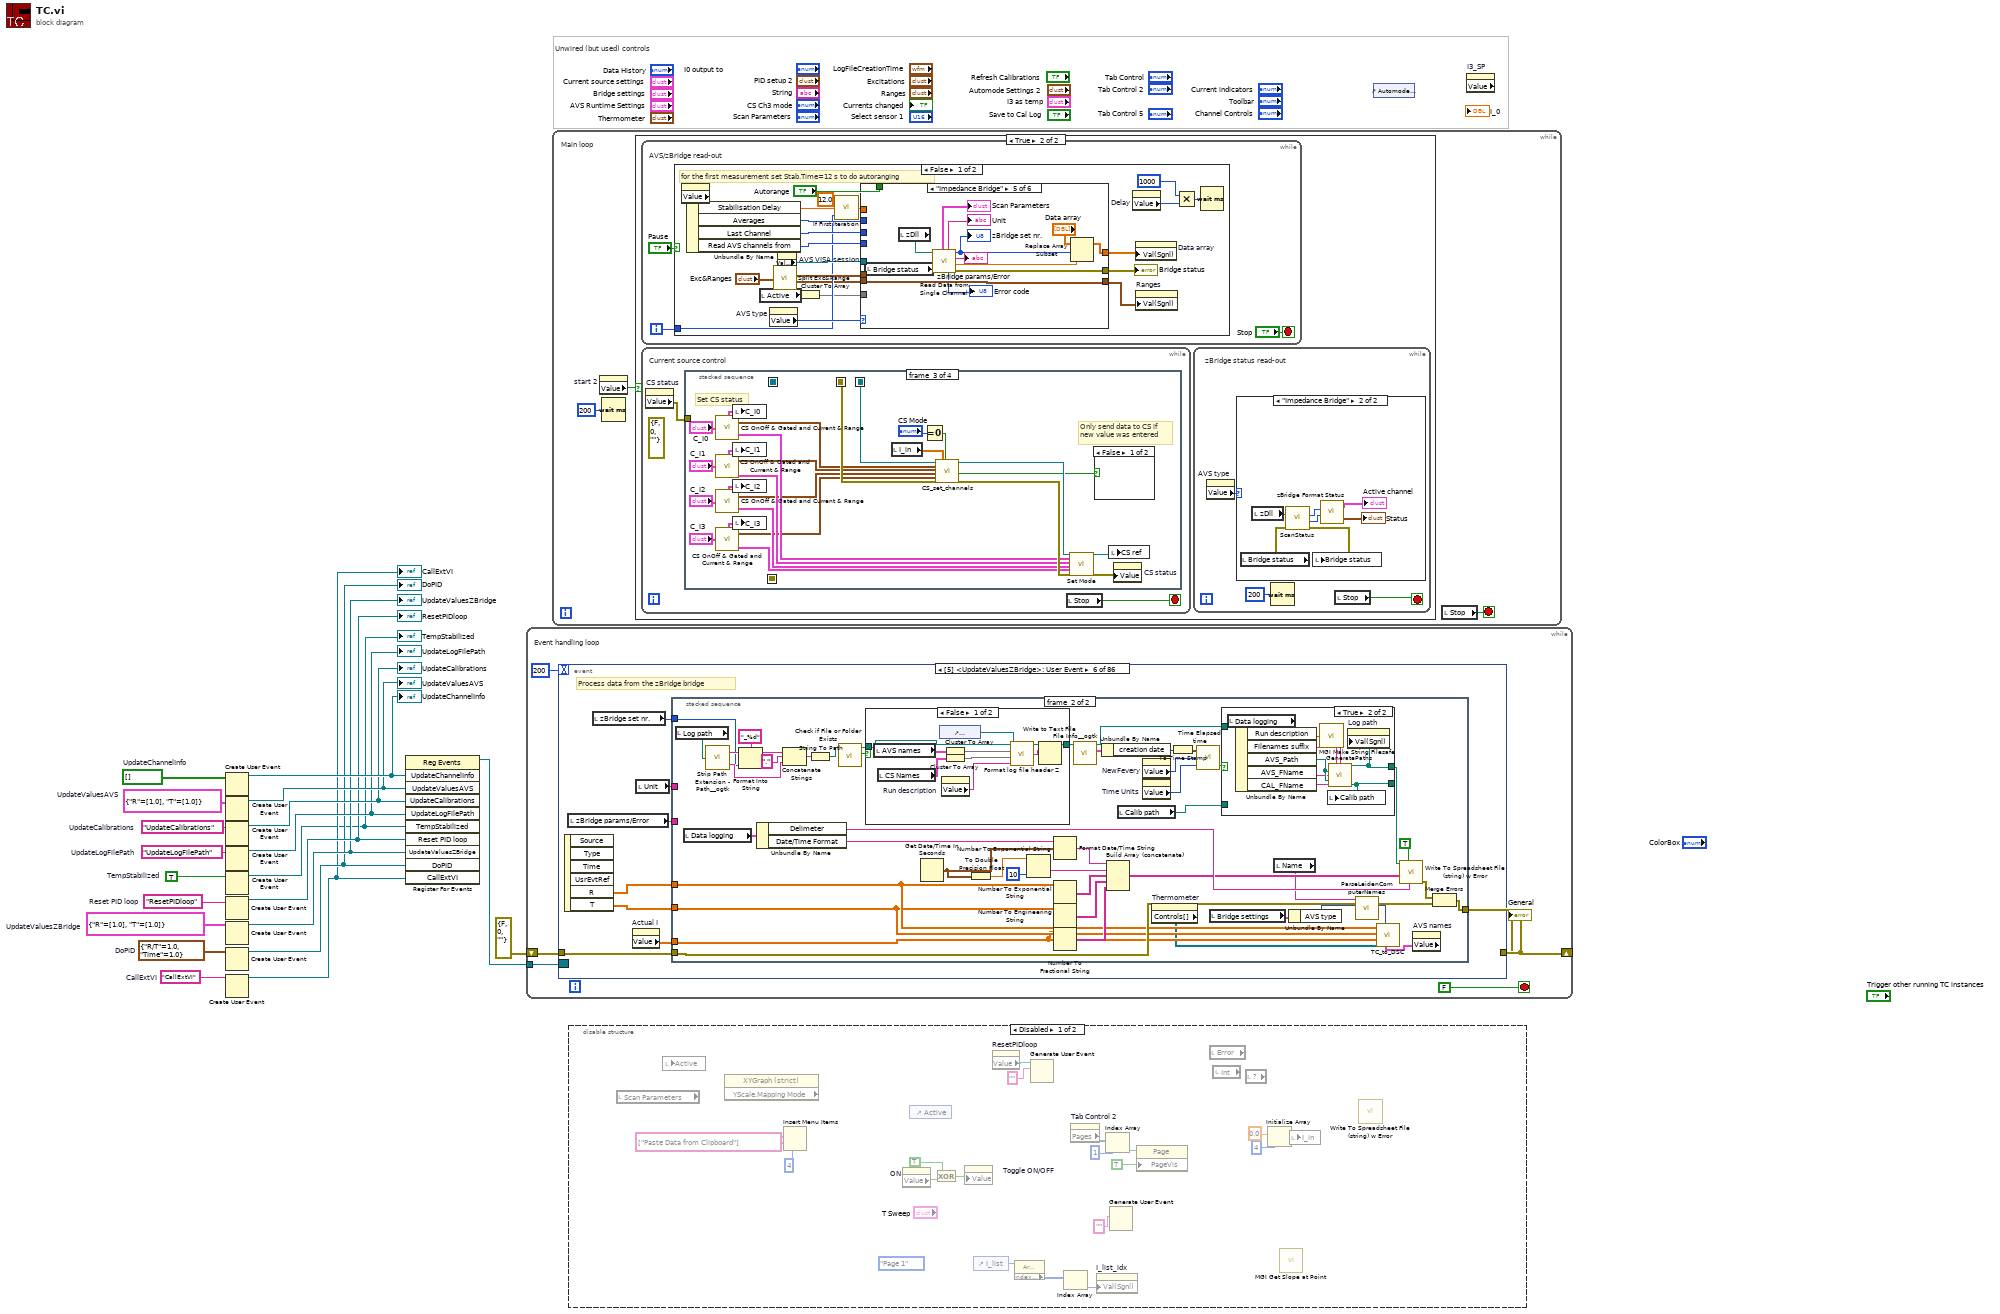
[diagram p0: block diagram]
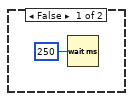
[diagram p3: hidden frame]
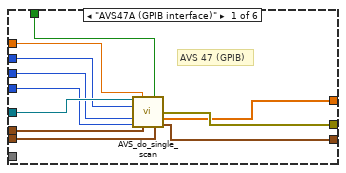
[diagram p5: hidden frame]
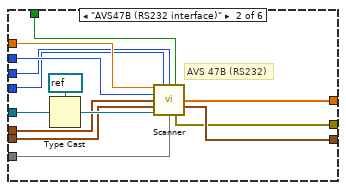
[diagram p6: hidden frame]
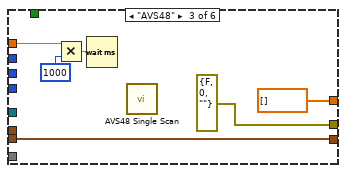
[diagram p7: hidden frame]
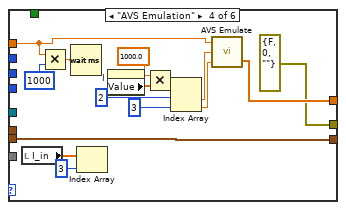
[diagram p8: hidden frame]
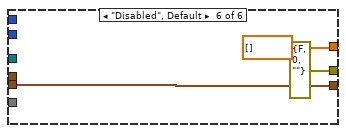
[diagram p9: hidden frame]
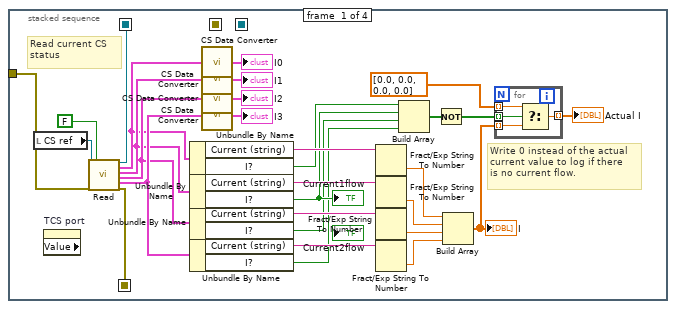
[diagram p11: hidden frame]
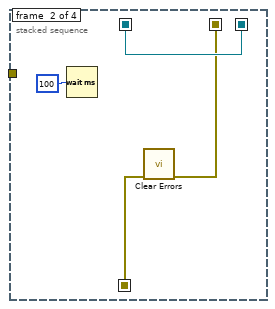
[diagram p12: hidden frame]
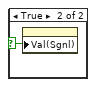
[diagram p13: hidden frame]
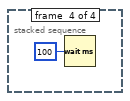
[diagram p14: hidden frame]
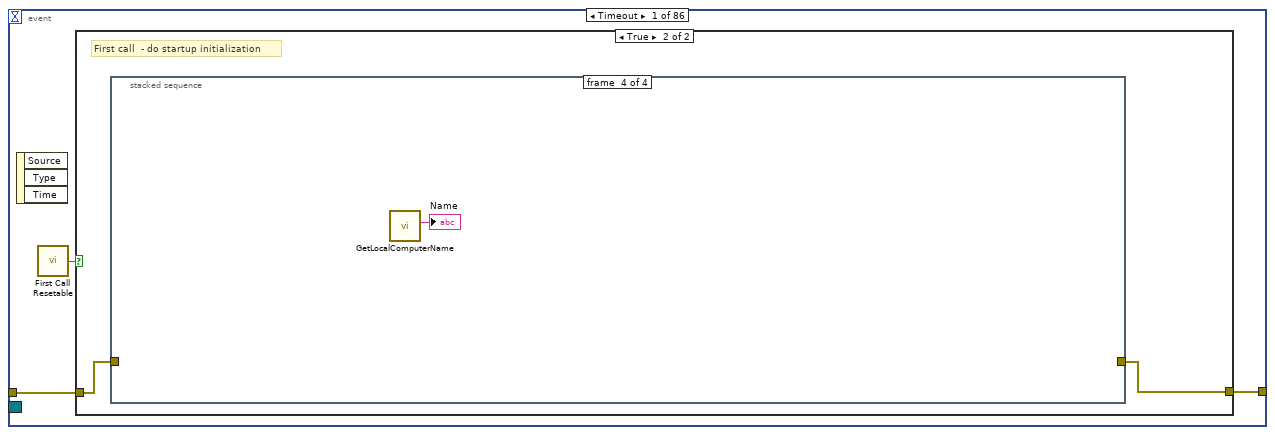
[diagram p15: hidden frame]
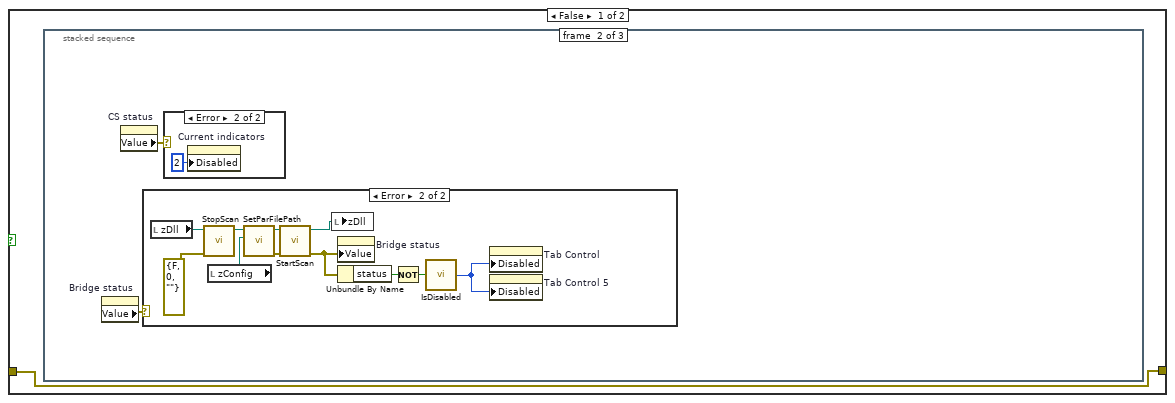
[diagram p16: hidden frame]
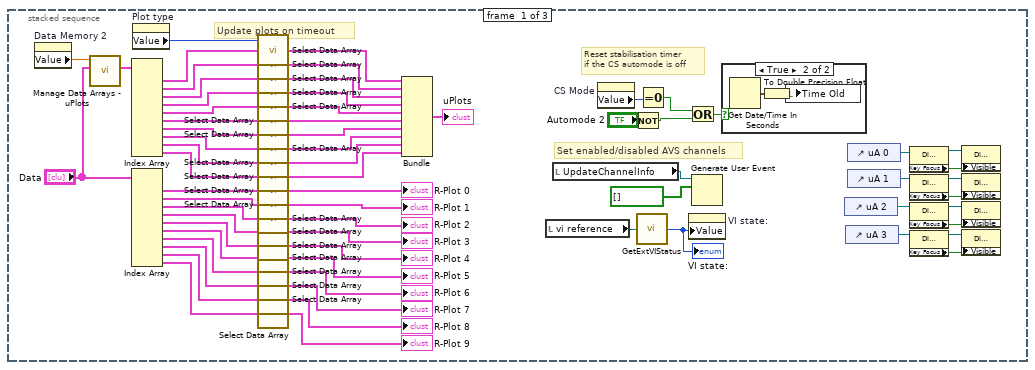
[diagram p17: hidden frame]
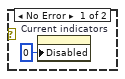
[diagram p19: hidden frame]
diagram:
  w2 = "CallExtVI"  # CallExtVI
  w4 = bool[] []  # UpdateChannelInfo
  w7 = cluster{"R/T":dbl, "Time":dbl} {"R/T"=1.0, "Time"=1.0}  # DoPID
  w8 = cluster{"R":dbl[], "T":dbl[]} {"R"=[1.0], "T"=[1.0]}  # UpdateValuesAVS
  w9 = cluster{"R":dbl[], "T":dbl[]} {"R"=[1.0], "T"=[1.0]}  # UpdateValuesZBridge
  w11 = "ResetPIDloop"  # Reset PID loop
  w13 = TRUE  # TempStabilized
  w14 = "UpdateLogFilePath"  # UpdateLogFilePath
  w17 = "UpdateCalibrations"  # UpdateCalibrations
  # "Unwired (but used) controls"
  n1 = Create User Event(user event datatype=w4) -> (user event=w20:refnum<user-event>)  [unwired: 1 in, 1 out]
  "UpdateChannelInfo" <- w20
  n2 = Create User Event(user event datatype=w8) -> (user event=w19:refnum<user-event>)  [unwired: 1 in, 1 out]
  "UpdateValuesAVS" <- w19
  n3 = Create User Event(user event datatype=w17) -> (user event=w16:refnum<user-event>)  [unwired: 1 in, 1 out]
  "UpdateCalibrations" <- w16
  n4 = Create User Event(user event datatype=w14) -> (user event=w15:refnum<user-event>)  [unwired: 1 in, 1 out]
  "UpdateLogFilePath" <- w15
  n5 = Create User Event ("TempStabilized")(user event datatype=w13) -> (user event=w1:refnum<user-event>)  [unwired: 1 in, 1 out]
  "TempStabilized" <- w1
  n6 = Create User Event(user event datatype=w11) -> (user event=w10:refnum<user-event>)  [unwired: 1 in, 1 out]
  "ResetPIDloop" <- w10
  n7 = Create User Event(user event datatype=w9) -> (user event=w6:refnum<user-event>)  [unwired: 1 in, 1 out]
  "UpdateValuesZBridge" <- w6
  n8 = Create User Event(user event datatype=w7) -> (user event=w5:refnum<user-event>)  [unwired: 1 in, 1 out]
  "DoPID" <- w5
  n9 = Create User Event(user event datatype=w2) -> (user event=w3:refnum<user-event>)  [unwired: 1 in, 1 out]
  "CallExtVI" <- w3
  n10 = register-events(w20, w19, w16, w15, w1, w10, w6, w5, w3) -> (reference out=w18:refnum<event-registration>)  [unwired: 2 in, 1 out]
  n11 = while {
    tunnel: w18 -> [w24]
    shift-right: [w21] -> _
    shift-left: errorcluster {"status"=FALSE, "code"=0, "source"=""} ("error in (no error)") -> [w22]
    stop <- FALSE stop-if-true
    # "Event handling loop"
    n12 = event shown="[5] <UpdateValuesZBridge>: User Event" {
      selector: w24 -> [_ _ _ _ _ _ _ _ _ _ _ _ _ _ _ _ _ _ _ _ _ _ _ _ _ _ _ _ _ _ _ _ _ _ _ _ _ _ _ _ _ _ _ _ _ _ _ _ _ _ _ _ _ _ _ _ _ _ _ _ _ _ _ _ _ _ _ _ _ _ _ _ _ _ _ _ _ _ _ _ _ _ _ _ _ _]
      dyn-events: _ -> [_ _ _ _ _ _ _ _ _ _ _ _ _ _ _ _ _ _ _ _ _ _ _ _ _ _ _ _ _ _ _ _ _ _ _ _ _ _ _ _ _ _ _ _ _ _ _ _ _ _ _ _ _ _ _ _ _ _ _ _ _ _ _ _ _ _ _ _ _ _ _ _ _ _ _ _ _ _ _ _ _ _ _ _ _ _]
      timeout: 200 -> [_ _ _ _ _ _ _ _ _ _ _ _ _ _ _ _ _ _ _ _ _ _ _ _ _ _ _ _ _ _ _ _ _ _ _ _ _ _ _ _ _ _ _ _ _ _ _ _ _ _ _ _ _ _ _ _ _ _ _ _ _ _ _ _ _ _ _ _ _ _ _ _ _ _ _ _ _ _ _ _ _ _ _ _ _ _]
      tunnel: w22 -> [w28 _ _ w420 w467 w551 _ _ w719 _ _ w816 w824 _ _ _ _ _ _ _ _ _ _ _ w1113 _ w1120 _ _ _ _ _ _ _ _ _ w1203 _ _ _ _ _ _ _ _ _ _ _ _ _ _ _ _ _ _ _ _ _ _ _ _ _ w1612 w1629 _ _ _ _ _ w1753 _ _ _ _ _ _ _ _ _ _ _ _ _ _ _ _]
      tunnel: [w27 _ _ w423 w466 w548 _ _ w718 _ _ w815 w824 _ _ _ _ _ _ _ _ _ _ _ w1113 _ w1120 _ _ _ _ _ _ _ _ _ w1203 _ _ _ _ _ _ _ _ _ _ _ _ _ _ _ _ _ _ _ _ _ _ _ _ _ w1611 w1628 _ _ _ _ _ w1753 _ _ _ _ _ _ _ _ _ _ _ _ _ _ _ _] -> w21
      event Timeout {
        n13 = event-data() -> ()  [unwired: 1 in, 3 out]
        n14 = call "First Call Resetable.vi"() -> ("First Call?"=w26:bool)
        n15 = case shown="True" w26 {
          tunnel: w28 -> [w29 w144]
          tunnel: [w29 w143] -> w27
          frame False {
            n16 = stacked-sequence {
              frame #0 {
                # "Update plots on timeout"
                # "Set enabled/disabled AVS channels"
                # "Reset stabilisation timer\nif the CS automode is off"
                n17 = property on="Data Memory 2" class="DigNum (strict)"() -> ("Value"=w91:dbl)  [unwired: 2 in, 2 out]
                n18 = call "Manage Data Arrays - uPlots.vi"("Data In"="Data", "Data Memory"=w91) -> ("Data Out"=w46:cluster{"R":dbl[], "T":dbl[], "Time":dbl[]}[])  [unwired: 7 in]
                n19 = Index Array(array=w46) -> (element #1=w61:cluster{"R":dbl[], "T":dbl[], "Time":dbl[]}, element #2=w62:cluster{"R":dbl[], "T":dbl[], "Time":dbl[]}, element #3=w63:cluster{"R":dbl[], "T":dbl[], "Time":dbl[]}, element #4=w64:cluster{"R":dbl[], "T":dbl[], "Time":dbl[]}, element #5=w65:cluster{"R":dbl[], "T":dbl[], "Time":dbl[]}, element #6=w66:cluster{"R":dbl[], "T":dbl[], "Time":dbl[]}, element #7=w67:cluster{"R":dbl[], "T":dbl[], "Time":dbl[]}, element #8=w68:cluster{"R":dbl[], "T":dbl[], "Time":dbl[]}, element #9=w69:cluster{"R":dbl[], "T":dbl[], "Time":dbl[]}, element #10=w70:cluster{"R":dbl[], "T":dbl[], "Time":dbl[]})  [unwired: 10 in]
                n20 = Index Array(array="Data") -> (element #1=w90:cluster{"R":dbl[], "T":dbl[], "Time":dbl[]}, element #2=w89:cluster{"R":dbl[], "T":dbl[], "Time":dbl[]}, element #3=w88:cluster{"R":dbl[], "T":dbl[], "Time":dbl[]}, element #4=w87:cluster{"R":dbl[], "T":dbl[], "Time":dbl[]}, element #5=w86:cluster{"R":dbl[], "T":dbl[], "Time":dbl[]}, element #6=w85:cluster{"R":dbl[], "T":dbl[], "Time":dbl[]}, element #7=w84:cluster{"R":dbl[], "T":dbl[], "Time":dbl[]}, element #8=w83:cluster{"R":dbl[], "T":dbl[], "Time":dbl[]}, element #9=w82:cluster{"R":dbl[], "T":dbl[], "Time":dbl[]}, element #10=w81:cluster{"R":dbl[], "T":dbl[], "Time":dbl[]})  [unwired: 10 in]
                n21 = property on="Plot type" class="Enum (strict)"() -> ("Value"=w49:enum16{"R vs Time", "T vs Time"})  [unwired: 2 in, 2 out]
                n22 = call "Select Data Array.vi"("Cluster 2"=w61, "Value"=w49) -> ("Cluster"=w71:cluster{"Time":dbl[], "T":dbl[]})
                n23 = call "Select Data Array.vi"("Cluster 2"=w62, "Value"=w49) -> ("Cluster"=w72:cluster{"Time":dbl[], "T":dbl[]})
                n24 = call "Select Data Array.vi"("Cluster 2"=w63, "Value"=w49) -> ("Cluster"=w73:cluster{"Time":dbl[], "T":dbl[]})
                n25 = call "Select Data Array.vi"("Cluster 2"=w64, "Value"=w49) -> ("Cluster"=w74:cluster{"Time":dbl[], "T":dbl[]})
                n26 = call "Select Data Array.vi"("Cluster 2"=w65, "Value"=w49) -> ("Cluster"=w80:cluster{"Time":dbl[], "T":dbl[]})
                n27 = call "Select Data Array.vi"("Cluster 2"=w66, "Value"=w49) -> ("Cluster"=w75:cluster{"Time":dbl[], "T":dbl[]})
                n28 = call "Select Data Array.vi"("Cluster 2"=w67, "Value"=w49) -> ("Cluster"=w76:cluster{"Time":dbl[], "T":dbl[]})
                n29 = call "Select Data Array.vi"("Cluster 2"=w68, "Value"=w49) -> ("Cluster"=w77:cluster{"Time":dbl[], "T":dbl[]})
                n30 = call "Select Data Array.vi"("Cluster 2"=w69, "Value"=w49) -> ("Cluster"=w78:cluster{"Time":dbl[], "T":dbl[]})
                n31 = call "Select Data Array.vi"("Cluster 2"=w70, "Value"=w49) -> ("Cluster"=w79:cluster{"Time":dbl[], "T":dbl[]})
                n32 = call "Select Data Array.vi"("Cluster 2"=w90, "Value"=w49) -> ("Cluster"=→"R-Plot 0":cluster{"Time":dbl[], "T":dbl[]})
                n33 = call "Select Data Array.vi"("Cluster 2"=w89, "Value"=w49) -> ("Cluster"=→"R-Plot 1":cluster{"Time":dbl[], "T":dbl[]})
                n34 = call "Select Data Array.vi"("Cluster 2"=w88, "Value"=w49) -> ("Cluster"=→"R-Plot 2":cluster{"Time":dbl[], "T":dbl[]})
                n35 = call "Select Data Array.vi"("Cluster 2"=w87, "Value"=w49) -> ("Cluster"=→"R-Plot 3":cluster{"Time":dbl[], "T":dbl[]})
                n36 = call "Select Data Array.vi"("Cluster 2"=w86, "Value"=w49) -> ("Cluster"=→"R-Plot 4":cluster{"Time":dbl[], "T":dbl[]})
                n37 = call "Select Data Array.vi"("Cluster 2"=w85, "Value"=w49) -> ("Cluster"=→"R-Plot 5":cluster{"Time":dbl[], "T":dbl[]})
                n38 = call "Select Data Array.vi"("Cluster 2"=w84, "Value"=w49) -> ("Cluster"=→"R-Plot 6":cluster{"Time":dbl[], "T":dbl[]})
                n39 = call "Select Data Array.vi"("Cluster 2"=w83, "Value"=w49) -> ("Cluster"=→"R-Plot 7":cluster{"Time":dbl[], "T":dbl[]})
                n40 = call "Select Data Array.vi"("Cluster 2"=w82, "Value"=w49) -> ("Cluster"=→"R-Plot 8":cluster{"Time":dbl[], "T":dbl[]})
                n41 = call "Select Data Array.vi"("Cluster 2"=w81, "Value"=w49) -> ("Cluster"=→"R-Plot 9":cluster{"Time":dbl[], "T":dbl[]})
                n42 = Bundle("Cluster"=w71, "Cluster"=w72, "Cluster"=w73, "Cluster"=w74, "Cluster"=w80, "Cluster"=w75, "Cluster"=w76, "Cluster"=w77, "Cluster"=w78, "Cluster"=w79) -> (→"uPlots":T38)  [unwired: 1 in]
                n43 = local read "vi reference"() -> (w45:refnum<vi>)
                n44 = local read "UpdateChannelInfo"() -> (w44:refnum<user-event>)
                n45 = property on="CS Mode" class="Enum (strict)"() -> ("Value"=w94:enum16{"Manual", "Automatic"})  [unwired: 2 in, 2 out]
                n46 = Not(x="Automode 2") -> (.not. x?=w93:bool)
                n47 = call "GetExtVIStatus.vi"("vi reference in"=w45) -> ("Exec.State"=w43:T30)  [unwired: 2 out]
                "VI state:" <- w43
                n48 = Equal To 0?(x=w94) -> (x = 0?=w42:bool)
                n49 = Or(x=w42, y=w93) -> (x .or. y?=w92:bool)
                n50 = property on="VI state:" class="Enum (strict)"("Value"=w43) -> ()  [unwired: 2 in, 2 out]
                n51 = Generate User Event(user event=w44, event data cluster=bool[] [] ("event data")) -> ()  [unwired: 2 in, 2 out]
                n52 = case shown="True" w92 {
                  frame False {
                  }
                  frame True {
                    n53 = Get Date/Time In Seconds() -> (seconds since 1Jan1904=w96:timestamp)
                    n54 = To Double Precision Float(number=w96) -> (double precision float=w97:dbl)
                    n55 = local write "Time Old"(w97) -> ()
                  }
                }
                n56 = control-ref of="uA 2"() -> (w30:refnum<vi>)
                n57 = control-ref of="uA 3"() -> (w31:refnum<vi>)
                n58 = control-ref of="uA 0"() -> (w41:refnum<vi>)
                n59 = control-ref of="uA 1"() -> (w37:refnum<vi>)
                n60 = property class="DigNum (strict)"(reference=w41) -> (reference out=w40:refnum<vi>, "Key Focus"=w39:bool)  [unwired: 1 in, 1 out]
                n61 = property class="DigNum (strict)"(reference=w37) -> (reference out=w38:refnum<vi>, "Key Focus"=w36:bool)  [unwired: 1 in, 1 out]
                n62 = property class="DigNum (strict)"(reference=w30) -> (reference out=w32:refnum<vi>, "Key Focus"=w33:bool)  [unwired: 1 in, 1 out]
                n63 = property class="DigNum (strict)"(reference=w31) -> (reference out=w34:refnum<vi>, "Key Focus"=w35:bool)  [unwired: 1 in, 1 out]
                n64 = property class="DigNum (strict)"(reference=w40, "Visible"=w39) -> ()  [unwired: 1 in, 2 out]
                n65 = property class="DigNum (strict)"(reference=w38, "Visible"=w36) -> ()  [unwired: 1 in, 2 out]
                n66 = property class="DigNum (strict)"(reference=w32, "Visible"=w33) -> ()  [unwired: 1 in, 2 out]
                n67 = property class="DigNum (strict)"(reference=w34, "Visible"=w35) -> ()  [unwired: 1 in, 2 out]
              }
              frame #1 {
                n68 = property on="Bridge status" class="Clust (strict)"() -> ("Value"=w99:errorcluster)  [unwired: 2 in, 2 out]
                n69 = property on="CS status" class="Clust (strict)"() -> ("Value"=w98:errorcluster)  [unwired: 2 in, 2 out]
                n70 = case shown="Error" w99 {
                  frame No Error {
                  }
                  frame Error {
                    n71 = local read "zDll"() -> (w112:path)
                    n72 = call "StopScan.vi"("error in (no error)"=errorcluster {"status"=FALSE, "code"=0, "source"=""}, "path in"=w112) -> ("path out"=w108:path)  [unwired: 8 in, 1 out]
                    n73 = local read "zConfig"() -> (w111:path)
                    n74 = call "SetParFilePath.vi"("path"=w111, "zDll"=w108) -> ("error out"=w110:errorcluster, "zDll out"=w109:path)  [unwired: 8 in]
                    n75 = call "StartScan.vi"("error in (no error)"=w110, "path in"=w109) -> ("error out"=w105:errorcluster, "path out"=w106:path)  [unwired: 8 in]
                    n76 = local write "zDll"(w106) -> ()
                    n77 = property on="Bridge status" class="Clust (strict)"("Value"=w105) -> ()  [unwired: 2 in, 2 out]
                    n78 = Unbundle By Name(w105) -> ("status"=w103:bool)
                    n79 = Not(x=w103) -> (.not. x?=w104:bool)
                    n80 = call "IsDisabled.vi"("Enabled?"=w104) -> ("Numeric"=w102:i16)
                    n81 = property on="Tab Control" class="TabCtl (strict)"("Disabled"=w102) -> ()  [unwired: 2 in, 2 out]
                    n82 = property on="Tab Control 5" class="TabCtl (strict)"("Disabled"=w102) -> ()  [unwired: 2 in, 2 out]
                  }
                }
                n83 = case shown="Error" w98 {
                  frame No Error {
                    n84 = property on="Current indicators" class="TabCtl (strict)"("Disabled"=u8 0) -> ()  [unwired: 2 in, 2 out]
                  }
                  frame Error {
                    n85 = property on="Current indicators" class="TabCtl (strict)"("Disabled"=u8 2) -> ()  [unwired: 2 in, 2 out]
                  }
                }
              }
              frame #2 {
                # "Check if the structure is \nnot empty and only one\nof Scalar or Array is set"
                # "Set FP control value from external script/program"
                n86 = local read "SetControl"() -> (w113:T1)
                n87 = Unbundle By Name(w113) -> ("Name"=w115:string, "Scalar"=w114:string, "Array"=w123:string[][])
                n88 = call "Empty 2D Array (String)__ogtk.vi"("Array"=w123) -> ("Empty Array?"=w120:bool)  [unwired: 8 in]
                n89 = Empty String/Path?(string/path=w115) -> (empty?=w119:bool)
                n90 = Empty String/Path?(string/path=w114) -> (empty?=w118:bool)
                n91 = Not(x=w119) -> (.not. x?=w117:bool)
                n92 = Not(x=w118) -> (.not. x?=w121:bool)
                n93 = Not(x=w120) -> (.not. x?=w124:bool)
                n94 = Exclusive Or(1:w124, 2:w121) -> (0:w122:bool)
                n95 = And(x=w117, y=w122) -> (x .and. y?=w116:bool)
                n96 = case shown="True" w116 {
                  tunnel: w115 -> [_ w128]
                  tunnel: w114 -> [_ w127]
                  tunnel: w123 -> [_ w126]
                  tunnel: w124 -> [_ w125]
                  frame False {
                  }
                  frame True {
                    n97 = flat-sequence {
                      tunnel: w128 -> [w132]
                      tunnel: w127 -> [w131]
                      tunnel: w126 -> [w129]
                      tunnel: w125 -> [w130]
                      frame #0 {
                        n98 = local read "VIRef"() -> (w133:T2)
                        n99 = case shown="True" w130 {
                          tunnel: w133 -> [w136 w139]
                          tunnel: w132 -> [w135 w138]
                          tunnel: w131 -> [w134 _]
                          tunnel: w129 -> [_ w137]
                          frame False {
                            n100 = call "Push2VI.vi"("New Value"=w134, "element"=w135, "VIRef"=w136) -> ()  [unwired: 8 in, 1 out]
                          }
                          frame True {
                            n101 = call "PushArray2VI.vi"("Str"=w137, "element"=w138, "VIRef"=w139) -> ()  [unwired: 8 in, 1 out]
                          }
                        }
                      }
                      frame #1 {
                        w141 = ""
                        n102 = Bundle(w141, w141, "Array"=string[][] []) -> (→"SetControl":cluster{string, string, "Array":string[][]})  [unwired: 1 in]
                      }
                    }
                  }
                }
              }
            }
          }
          frame True {
            # "First call  - do startup initialization"
            n103 = stacked-sequence {
              tunnel: w144 -> [_ w169 _ _]
              tunnel: [_ w160 _ _] -> w143
              frame #0 {
                w157 = u8 0 ("Disabled")
                n104 = property on="Tab Control 5" class="TabCtl (strict)"("Disabled"=w157) -> ()  [unwired: 2 in, 2 out]
                n105 = property on="Toolbar" class="TabCtl (strict)"("Disabled"=w157) -> ()  [unwired: 2 in, 2 out]
                n106 = property on="Tab Control" class="TabCtl (strict)"("Disabled"=w157) -> ()  [unwired: 2 in, 2 out]
                n107 = property on="Current indicators" class="TabCtl (strict)"("Disabled"=w157) -> ()  [unwired: 2 in, 2 out]
                n108 = property on="Tab Control 2" class="TabCtl (strict)"("Disabled"=w157) -> ()  [unwired: 2 in, 2 out]
                n109 = property on="String" class="Str"("Visible"=FALSE) -> ()  [unwired: 2 in, 2 out]
                n110 = property on="I_0" class="DigNum (strict)"("Value"=0.0 ("I3")) -> ()  [unwired: 2 in, 2 out]
                n111 = call "Current VIs Reference__ogtk.vi"() -> ("Current VI's reference"=w147:refnum<vi>)  [unwired: 5 in]
                n112 = call "Current VIs Parent Directory__ogtk.vi"("Relative path (.)"=path "Calibrations" ("Library Path")) -> ("Parent Directory (+ Relative)"=w153:path)  [unwired: 4 in]
                n113 = call "Current VIs Parent Directory__ogtk.vi"("Relative path (.)"=path "data/Temp Control.lvlib" ("Library Path")) -> ("Parent Directory (+ Relative)"=w155:path)  [unwired: 4 in]
                n114 = call "Current VIs Parent Directory__ogtk.vi"("Relative path (.)"=path "data/ImpBridgeDll.dll" ("Library Path")) -> ("Parent Directory (+ Relative)"=→"zDll":path)  [unwired: 4 in]
                n115 = call "Current VIs Parent Directory__ogtk.vi"("Relative path (.)"=path "data" ("Library Path")) -> ("Parent Directory (+ Relative)"=→"zConfig":path)  [unwired: 4 in]
                n116 = call "GetFrontPanelControls.vi"("Ref to VI"=w147) -> ("VIRef"=w146:T2)  [unwired: 9 in, 1 out]
                "VIRef" <- w146
                n117 = property on="AVS_CalFolder" class="Path"("Value"=w153) -> ()  [unwired: 2 in, 2 out]
                n118 = invoke class="App" method="Library.Deploy Library"("libPath"=w155) -> ()  [unwired: 4 in, 5 out]
                n119 = Unbundle By Name(w146) -> ("Full Name"=→"ControlNames":string[])
                n120 = property on="Minimize" class="Bool (strict)"("Val(Sgnl)"=FALSE ("Value (Signaling)")) -> ()  [unwired: 2 in, 2 out]
              }
              frame #1 {
                # "Read settings from registry"
                n121 = flat-sequence {
                  tunnel: [w184] -> w168
                  tunnel: w169 -> [w183]
                  tunnel: [w181] -> w167
                  tunnel: w168 -> [w189]
                  tunnel: [w189] -> w166
                  tunnel: [w187] -> w165
                  tunnel: w167 -> [w187]
                  tunnel: [w194] -> w164
                  tunnel: w166 -> [w193]
                  tunnel: [w191] -> w163
                  tunnel: w165 -> [w191]
                  tunnel: w164 -> [w200]
                  tunnel: [w200] -> w162
                  tunnel: [w198] -> w161
                  tunnel: w163 -> [w198]
                  tunnel: w162 -> [w203]
                  tunnel: [w202] -> w160
                  tunnel: w161 -> [w201]
                  frame #0 {
                    n122 = call "Current VIs Parent Directory__ogtk.vi"("Relative path (.)"=path "data/config.ini") -> ("Parent Directory (+ Relative)"=w181:path)  [unwired: 4 in]
                    n123 = control-ref of="Active"() -> (w173:refnum<vi>)
                    n124 = control-ref of="Automode Settings 2"() -> (w171:refnum<vi>)
                    n125 = control-ref of="Current source settings"() -> (w174:refnum<vi>)
                    n126 = control-ref of="Bridge settings"() -> (w185:refnum<vi>)
                    n127 = control-ref of="AVS Runtime Settings"() -> (w180:refnum<vi>)
                    n128 = control-ref of="I3 as temp"() -> (w172:refnum<vi>)
                    n129 = control-ref of="Data logging"() -> (w179:refnum<vi>)
                    n130 = control-ref of="PID setup 2"() -> (w178:refnum<vi>)
                    n131 = control-ref of="CS Names"() -> (w177:refnum<vi>)
                    n132 = control-ref of="CurCalibrations"() -> (w175:refnum<vi>)
                    n133 = control-ref of="AVS names"() -> (w176:refnum<vi>)
                    n134 = Build Array(w173, w174, w185, w180, w179, w178, w177, w176, w175, w172, w171) -> (w186:refnum<vi>[])
                    n135 = call "Save Load Settings to File by Ref with path.vi"("Array of Cluster References"=w186, "Action"=enum8{"Load", "Save"}."Load", "error in (no error)"=w183, "configuration file path"=w181) -> ("error out"=w184:errorcluster)  [unwired: 5 in]
                  }
                  frame #1 {
                    n136 = Wait (ms)(milliseconds to wait=250) -> ()  [unwired: 1 out]
                  }
                  frame #2 {
                    n137 = control-ref of="Thermometer"() -> (w192:refnum<vi>)
                    n138 = control-ref of="CurCalibrations"() -> (w190:refnum<vi>)
                    n139 = control-ref of="CurCalibrations"() -> ()  [unwired: 1 out]
                    n140 = control-ref of="AVS_CalFolder"() -> (w196:refnum<vi>)
                    n141 = control-ref of="Select sensor 1"() -> (w197:refnum<vi>)
                    n142 = control-ref of="Select sensor 1"() -> (w195:refnum<vi>)
                    n143 = call "ReloadCalibrations.vi"("error in (no error)"=w193, "Quick convert sensors"=w195, "CurCalibrations"=w190, "Calibration files path"=w196, "Channel1 sensors"=w197, "Channels list"=w192) -> ("error out"=w194:errorcluster)  [unwired: 1 in]
                  }
                  frame #3 {
                    n144 = Wait (ms)(milliseconds to wait=250) -> ()  [unwired: 1 out]
                  }
                  frame #4 {
                    n145 = disable-structure shown="Enabled" {
                      disable-tunnel: w203 -> [w206 w213]
                      disable-tunnel: [w205 w211] -> w202
                      disable-tunnel: w201 -> [w204 _]
                      frame Disabled {
                        (unwired) "SOFTWARE\\Leiden Cryogenics\\TC" ("subkey 2")
                        (unwired) T39."HKEY_CURRENT_USER" ("root key (HKEY_LOCAL_MACHINE) 2")
                        n146 = control-ref of="Thermometer"() -> (w208:refnum<vi>)
                        n147 = Build Array(w208) -> (w207:refnum<vi>[])
                        n148 = call "Save Load Settings to File by Ref with path.vi"("Array of Cluster References"=w207, "Action"=enum8{"Load", "Save"}."Load", "error in (no error)"=w206, "configuration file path"=w204) -> ("error out"=w205:errorcluster)  [unwired: 5 in]
                      }
                      frame Enabled {
                        n149 = property on="UpdateCalibrations" class="TypRef (strict)"(error in=w213) -> (error out=w212:errorcluster, "Value"=w214:refnum<user-event>)  [unwired: 1 in, 1 out]
                        n150 = Generate User Event(user event=w214, event data cluster="" ("event data"), error in=w212) -> (error out=w211:errorcluster)  [unwired: 1 in, 1 out]
                      }
                    }
                  }
                }
              }
              frame #2 {
                w224 = 0.0 ("T_error")
                w225 = u8 0 ("Disabled")
                # "Set enabled/disabled AVS channels"
                # "Print VI version on low left corner"
                # "Reset Current lists\nto first element"
                # "Reset pid parameters"
                # "Hardware settings"
                # "Reset currents lists"
                # "Set initial controls state"
                n151 = property on="Start" class="Bool (strict)"("Visible"=TRUE, "Disabled"=u8 0, "Value"=FALSE ("start")) -> ()  [unwired: 2 in, 2 out]
                n152 = property on="I_list_idx" class="DigNum (strict)"("Val(Sgnl)"=1 ("Value (Signaling)")) -> ()  [unwired: 2 in, 2 out]
                n153 = property on="CS Mode" class="Enum (strict)"("Val(Sgnl)"=enum16{"Manual", "Automatic"}."Manual" ("Value (Signaling)")) -> ()  [unwired: 2 in, 2 out]
                n154 = property on="I_tofirst" class="Bool (strict)"("Val(Sgnl)"=TRUE ("Value (Signaling)")) -> ()  [unwired: 2 in, 2 out]
                n155 = property on="AVS type" class="Enum (strict)"("Disabled"=w225) -> ()  [unwired: 2 in, 2 out]
                n156 = property on="Address" class="VISAName"("Disabled"=w225) -> ()  [unwired: 2 in, 2 out]
                n157 = property on="TCS_Port" class="VISAName"("Disabled"=w225) -> ()  [unwired: 2 in, 2 out]
                n158 = property on="CS type" class="Enum (strict)"("Disabled"=w225) -> ()  [unwired: 2 in, 2 out]
                n159 = property on="QCS/PCS Device" class="DigNum (strict)"("Disabled"=w225) -> ()  [unwired: 2 in, 2 out]
                n160 = property on="I0 output to" class="Enum (strict)"("Disabled"=u8 2, "Value"=T29."Channel 0" ("Map Channel 0 to")) -> ()  [unwired: 2 in, 2 out]
                n161 = property class="App"() -> ("App.Kind"=w220:T40)  [unwired: 2 in, 2 out]
                n162 = case shown="\"Run Time System\"" w220 {
                  tunnel: [w230 w241] -> w221
                  frame "invalid app kind", Default {
                    n163 = control-ref of="This VI"() -> (w237:refnum<vi>)
                    n164 = property class="VI"(reference=w237) -> ("Hist.Revision"=w236:u32)  [unwired: 1 in, 2 out]
                    n165 = Divide(x=w236, y=1000.0 ("x")) -> (x/y=w232:dbl)
                    n166 = Number To Fractional String(use system decimal point (T)=FALSE, number=w232, precision (6)=i16 2) -> (F-format string=w231:string)  [unwired: 1 in]
                    n167 = Concatenate Strings("" ("string"), w231) -> (w230:string)
                  }
                  frame "Run Time System" {
                    n168 = Current VI's Path() -> (path=w243:path)
                    n169 = Strip Path(path=w243) -> (stripped path=w242:path)  [unwired: 1 out]
                    n170 = Path To String(path=w242) -> (string=w240:string)
                    n171 = invoke class="FileVersionInfo" method="GetVersionInfo"(reference=refnum<k24> refnum (".NET object"), "fileName"=w240) -> ("GetVersionInfo"=w239:refnum<k24>)  [unwired: 2 in, 3 out]
                    n172 = property class="FileVersionInfo"(reference=w239) -> ("FileVersion"=w241:string)  [unwired: 1 in, 2 out]
                  }
                }
                "Revision" <- w221
                n173 = local write "Error"(w224) -> ()
                n174 = local write "Int"(w224) -> ()
                n175 = local read "UpdateChannelInfo"() -> (w219:refnum<user-event>)
                n176 = Generate User Event(user event=w219, event data cluster=bool[] [] ("event data")) -> ()  [unwired: 2 in, 2 out]
              }
              frame #3 {
                n177 = call <userlib>:"GetLocalComputerName.vi"() -> ("Name"=→"Name":string)  [unwired: 10 in, 1 out]
              }
            }
          }
        }
      }
      event "Start": Value Change {
        # "\"Start\" button clicked -> start measuring"
        n178 = event-data() -> ()  [unwired: 1 in, 6 out]
        n179 = stacked-sequence {
          frame #0 {
            n180 = property on="Run description" class="Str"() -> ("Value"=w247:string)  [unwired: 2 in, 2 out]
            n181 = property on="Ask on start?" class="Bool (strict)"() -> ("Value"=w246:bool)  [unwired: 2 in, 2 out]
            n182 = Not(x=w246) -> (.not. x?=w245:bool)
            n183 = call "Run Reference DLG.vi"("Enable"=w246, "Run Reference"=w247, "Dont' ask again"=w245) -> ("Dont' ask again"=w249:bool, "Run Reference"=w250:string, "OK"=w251:bool)  [unwired: 13 in, 1 out]
            n184 = Not(x=w249) -> (.not. x?=w248:bool)
            n185 = case shown="True" w251 {
              tunnel: w250 -> [_ w253]
              tunnel: w248 -> [_ w252]
              frame False {
              }
              frame True {
                n186 = property on="Run description" class="Str"("Val(Sgnl)"=w253) -> ()  [unwired: 2 in, 2 out]
                n187 = property on="Ask on start?" class="Bool (strict)"("Val(Sgnl)"=w252) -> ()  [unwired: 2 in, 2 out]
              }
            }
          }
          frame #1 {
            (unwired) T39."HKEY_CURRENT_USER" ("root key (HKEY_LOCAL_MACHINE) 2")
            # "Save new settings to config file"
            n188 = control-ref of="Active"() -> (w258:refnum<vi>)
            n189 = control-ref of="I3 as temp"() -> (w257:refnum<vi>)
            n190 = control-ref of="Automode Settings 2"() -> (w256:refnum<vi>)
            n191 = control-ref of="Automode Settings 2"() -> (w255:refnum<vi>)
            n192 = control-ref of="CS Names"() -> (w263:refnum<vi>)
            n193 = control-ref of="AVS names"() -> (w262:refnum<vi>)
            n194 = control-ref of="CurCalibrations"() -> (w259:refnum<vi>)
            n195 = control-ref of="Bridge settings"() -> (w268:refnum<vi>)
            n196 = control-ref of="AVS Runtime Settings"() -> (w269:refnum<vi>)
            n197 = control-ref of="Current source settings"() -> (w267:refnum<vi>)
            n198 = control-ref of="Thermometer"() -> (w270:refnum<vi>)
            n199 = control-ref of="PID setup 2"() -> (w271:refnum<vi>)
            n200 = control-ref of="Data logging"() -> (w266:refnum<vi>)
            n201 = Build Array(w258, w268, w269, w267, w266, w270, w271, w263, w262, w259, w257, w256, w255) -> (w265:refnum<vi>[])
            n202 = call "Current VIs Parent Directory__ogtk.vi"("Relative path (.)"=path "data/config.ini") -> ("Parent Directory (+ Relative)"=w260:path)  [unwired: 4 in]
            n203 = call "Save Load Settings to File by Ref with path.vi"("Array of Cluster References"=w265, "subkey"="SOFTWARE\\Leiden Cryogenics\\TC" ("subkey 2"), "Action"=enum8{"Load", "Save"}."Save", "configuration file path"=w260) -> ()  [unwired: 5 in, 1 out]
          }
          frame #2 {
            w284 = u8 2 ("Disabled")
            # "Reset stop button"
            # "Hide Disable Start button"
            # "Load external calibration VI"
            # "Set controls\nInitialize data for run"
            # "Lock hardware settings"
            n204 = property on="AVS type" class="Enum (strict)"("Disabled"=w284) -> ()  [unwired: 2 in, 2 out]
            n205 = property on="Address" class="VISAName"("Disabled"=w284) -> ()  [unwired: 2 in, 2 out]
            n206 = property on="AVS_SPort" class="VISAName"("Disabled"=w284) -> ()  [unwired: 2 in, 2 out]
            n207 = property on="TCS_Port" class="VISAName"("Disabled"=w284) -> ()  [unwired: 2 in, 2 out]
            n208 = property on="CS type" class="Enum (strict)"("Disabled"=w284) -> ()  [unwired: 2 in, 2 out]
            n209 = property on="QCS/PCS Device" class="DigNum (strict)"("Disabled"=w284) -> ()  [unwired: 2 in, 2 out]
            n210 = property on="I0 output to" class="Enum (strict)"("Disabled"=u8 0) -> ()  [unwired: 2 in, 2 out]
            n211 = Get Date/Time In Seconds() -> (seconds since 1Jan1904=w283:timestamp)
            n212 = To Double Precision Float(number=w283) -> (double precision float=w282:dbl)
            n213 = local write "Time Old"(w282) -> ()
            n214 = property on="External VI path" class="Path"() -> ("Value"=w281:path)  [unwired: 2 in, 2 out]
            n215 = vi-ref "OnTempStabilizedRef.vi"() -> (w280:refnum<vi>)
            n216 = Open VI Reference(type specifier VI Refnum (for type only)=w280, vi path=w281) -> (vi reference=→"vi reference":refnum<vi>)  [unwired: 4 in, 1 out]
            n217 = local write "VI called?"(FALSE ("VI called?")) -> ()
            n218 = property on="Start" class="Bool (strict)"("Visible"=TRUE, "Disabled"=u8 2) -> ()  [unwired: 2 in, 2 out]
            n219 = Initialize Array(cluster{"R":dbl[], "T":dbl[], "Time":dbl[]} {"R"=[], "T"=[], "Time"=[]}, 10 ("dimension size")) -> (w275:cluster{"R":dbl[], "T":dbl[], "Time":dbl[]}[])
            n220 = disable-structure shown="Enabled" {
              frame Enabled {
                n221 = property on="Stop" class="Bool (strict)"("Value"=FALSE ("MainStopButton")) -> ()  [unwired: 2 in, 2 out]
              }
              frame Disabled {
              }
            }
            n222 = local write "Data"(w275) -> ()
          }
          frame #3 {
            # "Initialize CS"
            n223 = local read "CS ref"() -> (w296:refnum<class "CS.lvclass">)
            n224 = call-dynamic "Initialize.vi"("CS in"=w296, "HW Address"="HW Address", "error in (no error)"=T33 {"error"=FALSE, "code"=0, "source"=""} ("error in")) -> ("CS out"=w289:refnum<class "CS.lvclass">, "Instrument ID"=→"ID":string, "error out"=w288:errorcluster)  [unwired: 10 in]
            n225 = call-dynamic "Get Currents & Ranges.vi"("CS.lvclass in"=w289, "error in (no error)"=w288) -> ("CS.lvclass out"=w297:refnum<class "CS.lvclass">, "I0"=w298:cluster{"Value":dbl, "Range":dbl}, "I1"=w290:cluster{"Value":dbl, "Range":dbl}, "I2"=w291:cluster{"Value":dbl, "Range":dbl}, "I3"=w292:cluster{"Value":dbl, "Range":dbl}, "error out"=w294:errorcluster)  [unwired: 12 in]
            "CS status" <- w294
            n226 = local write "CS ref"(w297) -> ()
            n227 = Unbundle By Name(w294) -> ("status"=w286:bool)
            n228 = case shown="False" w286 {
              tunnel: w290 -> [w310 _]
              tunnel: w291 -> [w309 _]
              tunnel: w292 -> [w308 _]
              tunnel: w298 -> [w302 _]
              frame False {
                n229 = Unbundle By Name(w302) -> ("Value"=w301:dbl, "Range"=w300:dbl)
                n230 = Unbundle By Name(w310) -> ("Value"=w307:dbl, "Range"=w306:dbl)
                n231 = Unbundle By Name(w309) -> ("Value"=w305:dbl, "Range"=w304:dbl)
                n232 = Unbundle By Name(w308) -> ("Value"=w299:dbl, "Range"=w303:dbl)
                n233 = property on="I" class="DigNum (strict)"("Value"=w301) -> ()  [unwired: 2 in, 2 out]
                n234 = property on="I" class="DigNum (strict)"("Value"=w307) -> ()  [unwired: 2 in, 2 out]
                n235 = property on="I" class="DigNum (strict)"("Value"=w305) -> ()  [unwired: 2 in, 2 out]
                n236 = property on="I" class="DigNum (strict)"("Value"=w299) -> ()  [unwired: 2 in, 2 out]
                n237 = property on="Range" class="Enum (strict)"("Value"=w300) -> ()  [unwired: 2 in, 2 out]
                n238 = property on="Range" class="Enum (strict)"("Value"=w306) -> ()  [unwired: 2 in, 2 out]
                n239 = property on="Range" class="Enum (strict)"("Value"=w304) -> ()  [unwired: 2 in, 2 out]
                n240 = property on="Range" class="Enum (strict)"("Value"=w303) -> ()  [unwired: 2 in, 2 out]
                n241 = property on="I_0" class="DigNum (strict)"("Value"=w299) -> ()  [unwired: 2 in, 2 out]
              }
              frame True {
              }
            }
          }
          frame #4 {
            # "Initialize AVS/zBridge"
            n242 = property on="AVS type" class="Enum (strict)"() -> ("Value"=w314:T35)  [unwired: 2 in, 2 out]
            n243 = case shown="\"Impedance Bridge\"" w314 {
              tunnel: [w322 w331 w348 refnum<visa-resource-name> refnum ("dup VISA session") refnum<visa-resource-name> refnum ("dup VISA session")] -> w313
              tunnel: [w321 w334 _ w357 errorcluster {"status"=FALSE, "code"=0, "source"=""} ("error out")] -> w312
              tunnel: [TRUE ("start 2") TRUE ("start 2") TRUE ("start 2") TRUE ("start 2") TRUE ("start 2")] -> w315
              tunnel: [_ _ w347 _ _] -> _
              frame "AVS47A (GPIB interface)" {
                # "Set default Parameters,\n enable Autoranging"
                n244 = property on="Address" class="VISAName"() -> ("Value"=w316:refnum<visa-resource-name>)  [unwired: 2 in, 2 out]
                n245 = call "AVS47IB Initialize.vi"("Instr. Descriptor (GPIB::)"=w316) -> ("VISA session"=w330:refnum<visa-resource-name>, "error out"=w317:errorcluster)  [unwired: 13 in]
                n246 = call "AVS47IB Stop.vi"("VISA session"=w330, "error in (no error)"=w317) -> ("dup VISA session"=w328:refnum<visa-resource-name>, "error out"=w320:errorcluster)  [unwired: 12 in]
                n247 = call "AVS47IB Go Remote.vi"("VISA session"=w328, "error in (no error)"=w320) -> ("dup VISA session"=w329:refnum<visa-resource-name>, "error out"=w319:errorcluster)  [unwired: 12 in]
                n248 = call "AVS47IB Configure 47IB.vi"("VISA session"=w329, "Printer Enabled (-1:no change)"=i8 0, "Buffer Enabled (-1:no change)"=i8 0, "Message Headers Included  (-1:no change)"=i8 0, "Autoranging Enabled (-1:no change)"=i8 1, "Stabilisation Delay (-1:no change)"=i8 15, "error in (no error)"=w319) -> ("dup VISA session"=w322:refnum<visa-resource-name>, "error out"=w321:errorcluster)  [unwired: 7 in]
              }
              frame "AVS47B (RS232 interface)" {
                n249 = property on="Bridge settings" class="Clust (strict)"() -> ("Value"=w339:T25)  [unwired: 2 in, 2 out]
                n250 = Unbundle By Name(w339) -> ("AVS_SPort"=w338:refnum<visa-resource-name>)
                n251 = call "InitPort_b.vi"("VISA resource"=w338) -> ("error out"=w333:errorcluster, "dup VISA resource"=w337:refnum<visa-resource-name>)  [unwired: 5 in]
                n252 = Type Cast(type=refnum<visa-resource-name> refnum ("dup VISA session"), x=w337) -> (*(type *) &x=w332:refnum<visa-resource-name>)
                n253 = case shown="Error" w333 {
                  selector: w333 -> [w340 w343]
                  tunnel: w332 -> [w341 w345]
                  tunnel: [w340 w344] -> w334
                  tunnel: [w341 refnum<visa-resource-name> refnum ("dup VISA session")] -> w331
                  frame No Error {
                  }
                  frame Error {
                    n254 = VISA Close(VISA resource name=w345, error in (no error)=w343) -> (error out=w344:errorcluster)
                  }
                }
              }
              frame "AVS48" {
                n255 = property on="Bridge settings" class="Clust (strict)"() -> ("Value"=w352:T25)  [unwired: 2 in, 2 out]
                n256 = Unbundle By Name(w352) -> ("AVS_SPort"=w349:refnum<visa-resource-name>)
                n257 = call "Configure Hardware.vi"("VISA RESOURCE NAME"=w349) -> ("THREAD OUT"=w346:string)  [unwired: 14 in]
                n258 = call "Configure Sensor Wiring of CHs.vi"("THREAD IN"=w346) -> ("THREAD OUT"=w347:string)  [unwired: 10 in]
                n259 = Type Cast(type=refnum<visa-resource-name> refnum ("dup VISA session"), x=w349) -> (*(type *) &x=w348:refnum<visa-resource-name>)
              }
              frame "Impedance Bridge" {
                n260 = local read "zConfig"() -> (w356:path)
                n261 = local read "zDll"() -> (w353:path)
                n262 = call "SetParFilePath.vi"("path"=w356, "zDll"=w353) -> ("error out"=w355:errorcluster, "zDll out"=w354:path)  [unwired: 8 in]
                n263 = call "StartScan.vi"("error in (no error)"=w355, "path in"=w354) -> ("error out"=w357:errorcluster)  [unwired: 8 in, 1 out]
              }
              frame "Disabled", Default {
              }
            }
            "AVS VISA session" <- w313
            "start 2" <- w315
            n264 = property on="Bridge status" class="Clust (strict)"("Value"=w312) -> ()  [unwired: 2 in, 2 out]
            n265 = property on="Data array" class="Arr (strict)"("Value"=dbl[] [0.0, 0.0, 0.0, 0.0, 0.0, 0.0, 0.0, 0.0, 0.0, 0.0] ("R_array")) -> ()  [unwired: 2 in, 2 out]
          }
          frame #5 {
            # "Generate paths for log files"
            n266 = Unbundle By Name("Data logging") -> ("Run description"=w366:string, "Filenames suffix"=w367:string, "AVS_Path"=w364:path, "AVS_FName"=w370:string, "CAL_FName"=w369:string)
            n267 = call "Create Dir if Non-Existant__ogtk.vi"("Directory Path"=w364) -> ("dup Directory Path"=w363:path)  [unwired: 8 in, 2 out]
            n268 = call "MGI Make String Filesafe.vi"("String In"=w366) -> ("Filesafe String Out"=w365:string)
            n269 = call "GeneratePaths.vi"("Filename Suffix"=w367, "Run description"=w365, "AVS_Path"=w363, "AVS_FName"=w370, "CAL_Path"=w363, "CAL_FName"=w369) -> ("Generated Log path"=w368:path, "Generated Calib path"=→"Calib path":path)  [unwired: 8 in]
            n270 = property on="Log path" class="Path"("Val(Sgnl)"=w368) -> ()  [unwired: 2 in, 2 out]
          }
        }
      }
      event "Stop": Value Change; Application Instance Close {
        # "\"Stop\" button pressed -> Stop measuring."
        n271 = event-data() -> ()  [unwired: 1 in, 3 out]
        n272 = flat-sequence {
          frame #0 {
            (unwired) T39."HKEY_CURRENT_USER" ("root key (HKEY_LOCAL_MACHINE) 2")
            # "Save settings to config file"
            n273 = control-ref of="Active"() -> (w375:refnum<vi>)
            n274 = control-ref of="Bridge settings"() -> (w384:refnum<vi>)
            n275 = control-ref of="AVS Runtime Settings"() -> (w383:refnum<vi>)
            n276 = control-ref of="Current source settings"() -> (w385:refnum<vi>)
            n277 = control-ref of="Data logging"() -> (w386:refnum<vi>)
            n278 = control-ref of="Thermometer"() -> (w382:refnum<vi>)
            n279 = control-ref of="PID setup 2"() -> (w381:refnum<vi>)
            n280 = control-ref of="CS Names"() -> (w380:refnum<vi>)
            n281 = control-ref of="AVS names"() -> (w379:refnum<vi>)
            n282 = control-ref of="CurCalibrations"() -> (w376:refnum<vi>)
            n283 = control-ref of="I3 as temp"() -> (w374:refnum<vi>)
            n284 = control-ref of="Automode Settings 2"() -> (w373:refnum<vi>)
            n285 = call "Current VIs Parent Directory__ogtk.vi"("Relative path (.)"=path "data/config.ini") -> ("Parent Directory (+ Relative)"=w377:path)  [unwired: 4 in]
            n286 = Build Array(w375, w384, w383, w385, w386, w382, w381, w380, w379, w376, w374, w373) -> (w388:refnum<vi>[])
            n287 = call "Save Load Settings to File by Ref with path.vi"("Array of Cluster References"=w388, "subkey"="SOFTWARE\\Leiden Cryogenics\\TC" ("subkey 2"), "Action"=enum8{"Load", "Save"}."Save", "configuration file path"=w377) -> ()  [unwired: 5 in, 1 out]
          }
          frame #1 {
            # "Free serial ports"
            n288 = control-ref of="AVS VISA session"() -> (w391:refnum<vi>)
            n289 = control-ref of="TCS_Port"() -> (w396:refnum<vi>)
            n290 = local read "zDll"() -> (w390:path)
            n291 = call "StopScan.vi"("path in"=w390) -> ()  [unwired: 9 in, 2 out]
            n292 = property class="VISAName"(reference=w391) -> (error out=w393:errorcluster, "Value"=w392:refnum<visa-resource-name>)  [unwired: 1 in, 1 out]
            n293 = property class="VISAName"(reference=w396) -> (error out=w394:errorcluster, "Value"=w395:refnum<visa-resource-name>)  [unwired: 1 in, 1 out]
            n294 = VISA Close(VISA resource name=w392, error in (no error)=w393) -> ()  [unwired: 1 out]
            n295 = VISA Close(VISA resource name=w395, error in (no error)=w394) -> ()  [unwired: 1 out]
          }
          frame #2 {
            w399 = u8 0 ("Disabled")
            # "Reset controls state"
            n296 = property on="Start" class="Bool (strict)"("Visible"=TRUE, "Disabled"=u8 0, "Value"=FALSE ("start")) -> ()  [unwired: 2 in, 2 out]
            n297 = property on="Stop" class="Bool (strict)"("Value"=FALSE ("MainStopButton")) -> ()  [unwired: 2 in, 2 out]
            n298 = property on="start 2" class="Bool (strict)"("Value"=FALSE ("start 2")) -> ()  [unwired: 2 in, 2 out]
            n299 = property on="AVS type" class="Enum (strict)"("Disabled"=w399) -> ()  [unwired: 2 in, 2 out]
            n300 = property on="Address" class="VISAName"("Disabled"=w399) -> ()  [unwired: 2 in, 2 out]
            n301 = property on="AVS_SPort" class="VISAName"("Disabled"=w399) -> ()  [unwired: 2 in, 2 out]
            n302 = property on="TCS_Port" class="VISAName"("Disabled"=w399) -> ()  [unwired: 2 in, 2 out]
            n303 = property on="CS type" class="Enum (strict)"("Disabled"=w399) -> ()  [unwired: 2 in, 2 out]
            n304 = property on="QCS/PCS Device" class="DigNum (strict)"("Disabled"=w399) -> ()  [unwired: 2 in, 2 out]
          }
          frame #3 {
            w403 = u8 2 ("Disabled")
            # "Disable UI"
            n305 = property on="Toolbar" class="TabCtl (strict)"("Disabled"=w403) -> ()  [unwired: 2 in, 2 out]
            n306 = property on="Tab Control" class="TabCtl (strict)"("Disabled"=w403) -> ()  [unwired: 2 in, 2 out]
            n307 = property on="Current indicators" class="TabCtl (strict)"("Disabled"=w403) -> ()  [unwired: 2 in, 2 out]
            n308 = property on="Tab Control 2" class="TabCtl (strict)"("Disabled"=w403) -> ()  [unwired: 2 in, 2 out]
            n309 = property on="Tab Control 5" class="TabCtl (strict)"("Disabled"=w403) -> ()  [unwired: 2 in, 2 out]
            n310 = property on="String" class="Str"("Visible"=TRUE) -> ()  [unwired: 2 in, 2 out]
          }
          frame #4 {
            # "Stop execution"
            n311 = Stop(stop? (T)=TRUE) -> ()
          }
        }
      }
      event "Data array": Value Change {
        # "Convert 8 elements AVS\narray to 10 elements"
        # "Received new data from AVS/zBridge. Do general tasks - update indicators, calculate temperature and pass the data further to \nAVS/zBridge specific processing"
        n312 = event-data() -> ("NewVal"=w417:dbl[])  [unwired: 1 in, 4 out]
        n313 = for {
          tunnel: w417 -> [w447] mode=indexing
          tunnel: [w445] -> w413 mode=indexing
          n314 = Less?(x=w447, y=1e+25) -> (x < y?=w448:bool)
          n315 = Select(t=w447, s=w448, f=inf) -> (s? t:f=w445:dbl)
        }
        n316 = Index Array(array=w413) -> (element #1=→"R0":dbl, element #2=→"R1":dbl, element #3=→"R2":dbl, element #4=→"R3":dbl, element #5=→"R4":dbl, element #6=→"R5":dbl, element #7=→"R6":dbl, element #8=→"R7":dbl, element #9=→"R8":dbl, element #10=→"R9":dbl)  [unwired: 10 in]
        n317 = Array To Cluster(array=w413) -> (cluster=w407:T41)
        "R" <- w407
        n318 = Cluster To Array(cluster=w407) -> (array=w406:dbl[])
        n319 = Absolute Value(x=w406) -> (abs(x)=w414:dbl[])
        n320 = property on="Allow neg R" class="Bool (strict)"() -> ("Value"=w412:bool)  [unwired: 2 in, 2 out]
        n321 = Select(t=w406, s=w412, f=w414) -> (s? t:f=w411:dbl[])
        n322 = local read "CurCalibrations"() -> (w419:T23)
        n323 = property on="AVS_CalFolder" class="Path"() -> ("Value"=w427:path)  [unwired: 2 in, 2 out]
        n324 = Cluster To Array(cluster=w419) -> (array=w418:string[])
        n325 = call "Resistance to Temp no Ext.vi"("error in"=w420, "Path"=w427, "CurCalibrations"=w418, "Resistance"=w411) -> ("Temperature"=w409:dbl[])  [unwired: 1 in, 3 out]
        "T_array" <- w409
        n326 = Array To Cluster(array=w409) -> (cluster=w425:T42)
        "T" <- w425
        n327 = Unbundle(w425) -> ("Temperature[0]"=→"T0":dbl, "Temperature[1]"=→"T1":dbl, "Temperature[2]"=→"T2":dbl, "Temperature[3]"=→"T3":dbl, "Temperature[4]"=→"T4":dbl, "Temperature[5]"=→"T5":dbl, "Temperature[6]"=→"T6":dbl, "Temperature[7]"=→"T7":dbl, "Temperature[8]"=→"T8":dbl, "Temperature[9]"=→"T9":dbl)
        n328 = property on="Mode Buttons" class="RadioBtnsControl (strict)"() -> ("Value"=w424:T13)  [unwired: 2 in, 2 out]
        n329 = Array To Cluster(array=w411) -> (cluster=w410:T41)
        n330 = Array To Cluster(array=w409) -> (cluster=w408:T42)
        n331 = case shown="\"No Selection\", Default" w424 {
          tunnel: w408 -> [w459 _]
          tunnel: w410 -> [w460 _]
          frame "No Selection", Default {
            n332 = Get Date/Time In Seconds() -> (seconds since 1Jan1904=w462:timestamp)
            n333 = To Double Precision Float(number=w462) -> (double precision float=→"Time":dbl)
            "Small R" <- w460
            "Small T" <- w459
          }
          frame "Cursor Mode" {
          }
        }
        n334 = Bundle(w411, "Temperature"=w409) -> (w422:cluster{dbl[], "Temperature":dbl[]})  [unwired: 1 in]
        n335 = property on="AVS type" class="Enum (strict)"() -> ("Value"=w421:T35)  [unwired: 2 in, 2 out]
        n336 = case shown="\"AVS47B (RS232 interface)\", Default" w421 {
          tunnel: [w453 w454 w457] -> w423
          tunnel: w420 -> [w452 w454 w458]
          tunnel: w422 -> [w450 _ w456]
          frame "AVS47B (RS232 interface)", Default {
            n337 = local read "UpdateValuesAVS"() -> (w451:refnum<user-event>)
            n338 = Generate User Event(user event=w451, event data cluster=w450, error in=w452) -> (error out=w453:errorcluster)  [unwired: 1 in, 1 out]
          }
          frame "Disabled" {
          }
          frame "Impedance Bridge" {
            n339 = local read "UpdateValuesZBridge"() -> (w455:refnum<user-event>)
            n340 = Generate User Event(user event=w455, event data cluster=w456, error in=w458) -> (error out=w457:errorcluster)  [unwired: 1 in, 1 out]
          }
        }
      }
      event User Event {
        # "Process data from the AVS bridge"
        n341 = event-data() -> ("R"=w464:dbl[], "T"=w463:dbl[])  [unwired: 1 in]
        n342 = property on="Actual I" class="Arr (strict)"() -> ("Value"=w465:dbl[])  [unwired: 2 in, 2 out]
        n343 = stacked-sequence {
          tunnel: w467 -> [_ w499]
          tunnel: [_ w513] -> w466
          tunnel: w465 -> [_ w496]
          tunnel: w464 -> [w486 w498]
          tunnel: w463 -> [w487 w497]
          frame #0 {
            # "Filter data and add it to the data array. \nDo PID"
            n344 = property on="AVS Runtime Settings" class="Clust (strict)"() -> ("Value"=w475:T17)  [unwired: 2 in, 2 out]
            n345 = Unbundle By Name(w475) -> ("Y_max"=w478:dbl, "Y_min"=w477:dbl, "Filter graphs:"=w476:bool)
            n346 = local read "Data"() -> (w472:cluster{"R":dbl[], "T":dbl[], "Time":dbl[]}[])
            n347 = property on="Data Memory" class="DigNum (strict)"() -> ("Value"=w480:u16)  [unwired: 2 in, 2 out]
            n348 = Get Date/Time In Seconds() -> (seconds since 1Jan1904=w474:timestamp)
            n349 = To Double Precision Float(number=w474) -> (double precision float=w471:dbl)
            n350 = call "Manage Data Arrays - AVS.vi"("Y_max"=w478, "Y_min"=w477, "Filter Graph Results"=w476, "Append New Data"=TRUE, "Data In"=w472, "Curr R"=w486, "Curr T"=w487, "Curr Time"=w471, "Data Memory"=w480) -> ("Data Out"=w473:cluster{"R":dbl[], "T":dbl[], "Time":dbl[]}[])  [unwired: 10 in]
            n351 = property on="FB on" class="Enum (strict)"() -> ("Value"=w468:enum16{"Resistance", "Temperature"})  [unwired: 2 in, 2 out]
            n352 = local write "Data"(w473) -> ()
            n353 = property on="AVS Channel" class="DigNum (strict)"() -> ("Value"=w469:i32)  [unwired: 2 in, 2 out]
            n354 = Index Array(array=w486, index=w469) -> (element=w485:dbl)
            n355 = Index Array(array=w487, index=w469) -> (element=w484:dbl)
            n356 = case shown="\"Temperature\"" w468 {
              tunnel: w485 -> [w488 _]
              tunnel: [w488 w489] -> w482
              tunnel: w484 -> [_ w489]
              frame "Resistance", Default {
              }
              frame "Temperature" {
              }
            }
            "T controlled" <- w482
            n357 = local read "DoPID"() -> (w483:refnum<user-event>)
            n358 = Bundle(w482, w471) -> (w481:cluster{dbl, dbl})  [unwired: 1 in]
            n359 = Generate User Event(user event=w483, event data cluster=w481) -> ()  [unwired: 2 in, 2 out]
            n360 = local write "Units"(T5 {"AVS Name 0"="O\u0000h\u0000m\u0000\u0000\u0000\u0000\u0000\u0000\u0000\u0000\u0000\u0000\u0000\u0000\u0000\u0000\u0000", "AVS Name 1"="O\u0000h\u0000m\u0000\u0000\u0000\u0000\u0000\u0000\u0000\u0000\u0000\u0000\u0000\u0000\u0000\u0000\u0000", "AVS Name 2"="O\u0000h\u0000m\u0000\u0000\u0000\u0000\u0000\u0000\u0000\u0000\u0000\u0000\u0000\u0000\u0000\u0000\u0000", "AVS Name 3"="O\u0000h\u0000m\u0000\u0000\u0000\u0000\u0000\u0000\u0000\u0000\u0000\u0000\u0000\u0000\u0000\u0000\u0000", "AVS Name 4"="O\u0000h\u0000m\u0000\u0000\u0000\u0000\u0000\u0000\u0000\u0000\u0000\u0000\u0000\u0000\u0000\u0000\u0000", "AVS Name 5"="O\u0000h\u0000m\u0000\u0000\u0000\u0000\u0000\u0000\u0000\u0000\u0000\u0000\u0000\u0000\u0000\u0000\u0000", "AVS Name 6"="O\u0000h\u0000m\u0000\u0000\u0000\u0000\u0000\u0000\u0000\u0000\u0000\u0000\u0000\u0000\u0000\u0000\u0000", "AVS Name 7"="O\u0000h\u0000m\u0000\u0000\u0000\u0000\u0000\u0000\u0000\u0000\u0000\u0000\u0000\u0000\u0000\u0000\u0000", "AVS Name 8"="O\u0000h\u0000m\u0000\u0000\u0000\u0000\u0000\u0000\u0000\u0000\u0000\u0000\u0000\u0000\u0000\u0000\u0000", "AVS Name 9"="O\u0000h\u0000m\u0000\u0000\u0000\u0000\u0000\u0000\u0000\u0000\u0000\u0000\u0000\u0000\u0000\u0000\u0000"} ("Units")) -> ()
          }
          frame #1 {
            # "Save data to log file"
            n361 = local read "Calib path"() -> (w512:path)
            n362 = local read "Log path"() -> (w511:path)
            n363 = call <vilib>:"Check if File or Folder Exists.vi"("path"=w511) -> ("file or folder exists?"=w503:bool, "dup path"=w504:path)  [unwired: 8 in, 1 out]
            n364 = case shown="False" w503 {
              tunnel: w504 -> [w540 w547]
              tunnel: [w540 w547] -> w505
              frame False {
                n365 = control-ref of="Thermometer"() -> (w543:refnum<vi>)
                n366 = property on="Run description" class="Str"() -> ("Value"=w539:string)  [unwired: 2 in, 2 out]
                n367 = Cluster To Array(cluster="AVS names") -> (array=w545:string[])
                n368 = Cluster To Array(cluster="CS Names") -> (array=w546:string[])
                n369 = call "Format log file header Z.vi"("Thermometer"=w543, "AVS names"=w545, "CS Names"=w546, "Run description"=w539) -> ("String"=w541:string)  [unwired: 1 in]
                n370 = Write to Text File(file (use dialog)=w540, text=w541) -> ()  [unwired: 2 in, 3 out]
              }
              frame True {
              }
            }
            n371 = property on="Data logging" class="Clust (strict)"() -> ("Value"=w526:T27)  [unwired: 2 in, 2 out]
            n372 = Unbundle By Name(w526) -> ("Delimeter"=w527:string, "Date/Time Format"=w525:string)
            n373 = Get Date/Time In Seconds() -> (seconds since 1Jan1904=w518:timestamp)
            n374 = To Double Precision Float(number=w518) -> (double precision float=w516:dbl)
            n375 = call "File Info__ogtk.vi"("file"=w505) -> ("file info"=w501:T43, "file out"=w510:path)  [unwired: 5 in, 1 out]
            n376 = Unbundle By Name(w501) -> ("creation date"=w502:u32)
            n377 = Number To Exponential String(number=w516, precision (6)=i16 10) -> (E-format string=w517:string)  [unwired: 2 in]
            n378 = Format Date/Time String(time format string (%c)=w525, seconds (now)=w518) -> (date/time string=w522:string)  [unwired: 1 in]
            n379 = Number To Fractional String(number=w498) -> (F-format string=w524:string[])  [unwired: 3 in]
            n380 = Number To Fractional String(number=w497) -> (F-format string=w523:string[])  [unwired: 3 in]
            n381 = Number To Fractional String(number=w496) -> (F-format string=w521:string[])  [unwired: 3 in]
            n382 = property on="NewFevery" class="DigNum (strict)"() -> ("Value"=w506:u32)  [unwired: 2 in, 2 out]
            n383 = property on="Time Units" class="Enum (strict)"() -> ("Value"=w507:enum16{"Minutes", "Hours", "Days"})  [unwired: 2 in, 2 out]
            n384 = To Time Stamp(1:w502) -> (0:w508:timestamp)
            n385 = Build Array (concatenate)(w522, w517, w524, w523, w521) -> (w520:string[])
            n386 = call "Time Elapsed time.vi"("Time Units"=w507, "Delay Time"=w506, "Time Old In"=w508) -> ("T>dT?"=w509:bool)  [unwired: 2 out]
            n387 = case shown="True" w509 {
              tunnel: [w529 w532] -> w500
              tunnel: [w528 w533] -> _
              tunnel: w510 -> [w529 _]
              tunnel: w512 -> [w528 _]
              frame False {
              }
              frame True {
                n388 = local read "Data logging"() -> (w534:T27)
                n389 = Unbundle By Name(w534) -> ("Run description"=w530:string, "AVS_Path"=w538:path, "AVS_FName"=w536:string, "CAL_FName"=w537:string, "Filenames suffix"=w535:string)
                n390 = call "MGI Make String Filesafe.vi"("String In"=w530) -> ("Filesafe String Out"=w531:string)
                n391 = call "GeneratePaths.vi"("Filename Suffix"=w535, "Run description"=w531, "AVS_Path"=w538, "AVS_FName"=w536, "CAL_Path"=w538, "CAL_FName"=w537) -> ("Generated Log path"=w532:path, "Generated Calib path"=w533:path)  [unwired: 8 in]
                n392 = local write "Calib path"(w533) -> ()
                n393 = property on="Log path" class="Path"("Val(Sgnl)"=w532) -> ()  [unwired: 2 in, 2 out]
              }
            }
            n394 = property on="Thermometer" class="Clust (strict)"() -> ("Controls[]"=w495:refnum<vi>[])  [unwired: 2 in, 2 out]
            n395 = local read "Bridge settings"() -> (w491:T25)
            n396 = Unbundle By Name(w491) -> ("AVS type"=w490:T35)
            n397 = local read "Name"() -> (w493:string)
            n398 = call <userlib>:"ParseLeidenComputerNames.vi"("AVS type"=w490, "computer name"=w493) -> ("AVS Type"=w492:T44)  [unwired: 7 in, 2 out]
            n399 = call "Write To Spreadsheet File (string) w Error.vi"("delimiter (\\t)"=w527, "append to file? (new file:F)"=TRUE, "1D data"=w520, "file path (dialog if empty)"=w500) -> ("error out"=w514:errorcluster)  [unwired: 6 in, 1 out]
            n400 = property on="AVS names" class="Clust (strict)"() -> ("Value"=w494:T5)  [unwired: 2 in, 2 out]
            n401 = call <userlib>:"TC_to_DSC.vi"("AVS names"=w494, "AVS Type"=w492, "Array"=w495, "I"=w496, "T"=w497, "R"=w498) -> ()  [unwired: 6 in]
            n402 = Merge Errors(w514, w499) -> (w513:errorcluster)
          }
        }
      }
      event User Event {
        # "Process data from the zBridge bridge"
        n403 = event-data() -> ("R"=w554:dbl[], "T"=w553:dbl[])  [unwired: 1 in, 4 out]
        n404 = local read "zBridge params/Error"() -> (w549:string)
        n405 = local read "zBridge set nr."() -> (w555:u8)
        n406 = property on="Actual I" class="Arr (strict)"() -> ("Value"=w552:dbl[])  [unwired: 2 in, 2 out]
        n407 = local read "Unit"() -> (w550:string)
        n408 = stacked-sequence {
          tunnel: w549 -> [w581 _]
          tunnel: w555 -> [w564 w600]
          tunnel: w554 -> [w563 w597]
          tunnel: w553 -> [w562 w596]
          tunnel: w552 -> [_ w595]
          tunnel: w551 -> [_ w623]
          tunnel: [_ w622] -> w548
          tunnel: w550 -> [w567 _]
          frame #0 {
            # "Only do PID after measuring\non selected channel"
            n409 = local read "zBridge params"() -> (w566:T5)
            n410 = local read "Units"() -> (w568:T5)
            n411 = Cluster To Array(cluster=w568) -> (array=w571:string[])
            n412 = Cluster To Array(cluster=w566) -> (array=w582:string[])
            n413 = Replace Array Subset(array=w571, new element=w567, index=w564) -> (w570:string[])
            n414 = Replace Array Subset(array=w582, new element=w581, index=w564) -> (w583:string[])
            n415 = Array To Cluster(array=w570) -> (cluster=→"Units":T45)
            n416 = Array To Cluster(array=w583) -> (cluster=→"zBridge params":T46)
            n417 = property on="AVS Runtime Settings" class="Clust (strict)"() -> ("Value"=w575:T17)  [unwired: 2 in, 2 out]
            n418 = Unbundle By Name(w575) -> ("Y_max"=w578:dbl, "Y_min"=w577:dbl, "Filter graphs:"=w576:bool)
            n419 = local read "Data"() -> (w572:cluster{"R":dbl[], "T":dbl[], "Time":dbl[]}[])
            n420 = property on="FB on" class="Enum (strict)"() -> ("Value"=w556:enum16{"Resistance", "Temperature"})  [unwired: 2 in, 2 out]
            n421 = property on="AVS Channel" class="DigNum (strict)"() -> ("Value"=w557:i32)  [unwired: 2 in, 2 out]
            n422 = property on="Data Memory" class="DigNum (strict)"() -> ("Value"=w580:u16)  [unwired: 2 in, 2 out]
            n423 = Get Date/Time In Seconds() -> (seconds since 1Jan1904=w574:timestamp)
            n424 = To Double Precision Float(number=w574) -> (double precision float=w559:dbl)
            n425 = Index Array(array=w563, index=w557) -> (element=w560:dbl)
            n426 = Index Array(array=w562, index=w557) -> (element=w561:dbl)
            n427 = call "Manage Data Arrays - zBridge.vi"("Y_max"=w578, "Y_min"=w577, "Filter Graph Results"=w576, "Append New Data"=TRUE, "Data In"=w572, "Curr R"=w563, "Curr T"=w562, "Curr Time"=w559, "Channel"=w564, "Data Memory"=w580) -> ("Data Out"=w573:cluster{"R":dbl[], "T":dbl[], "Time":dbl[]}[])  [unwired: 9 in]
            n428 = case shown="\"Resistance\", Default" w556 {
              tunnel: w561 -> [_ w586]
              tunnel: w560 -> [w585 _]
              tunnel: [w585 w586] -> w558
              frame "Resistance", Default {
              }
              frame "Temperature" {
              }
            }
            n429 = local write "Data"(w573) -> ()
            n430 = Equal?(x=w564, y=w557) -> (x = y?=w565:bool)
            n431 = case shown="True" w565 {
              tunnel: w558 -> [_ w588]
              tunnel: w559 -> [_ w587]
              frame False {
              }
              frame True {
                n432 = local read "DoPID"() -> (w590:refnum<user-event>)
                n433 = Bundle(w588, w587) -> (w589:cluster{dbl, dbl})  [unwired: 1 in]
                n434 = Generate User Event(user event=w590, event data cluster=w589) -> ()  [unwired: 2 in, 2 out]
              }
            }
            n435 = property on="T controlled" class="DigNum (strict)"("Value"=w558) -> ()  [unwired: 2 in, 2 out]
          }
          frame #1 {
            n436 = local read "Log path"() -> (w603:path)
            n437 = local read "Data logging"() -> (w621:T27)
            n438 = call "Strip Path Extension - Path__ogtk.vi"("path"=w603) -> ("root"=w604:string, "extension"=w607:string)
            n439 = Format Into String(format string="_%d", initial string=w604, w600) -> (resulting string=w605:string)  [unwired: 1 in, 1 out]
            n440 = Unbundle By Name(w621) -> ("Delimeter"=w636:string, "Date/Time Format"=w635:string)
            n441 = Concatenate Strings(w605, "." ("string"), w607) -> (w602:string)
            n442 = String To Path(string=w602) -> (path=w601:path)
            n443 = call <vilib>:"Check if File or Folder Exists.vi"("path"=w601) -> ("file or folder exists?"=w612:bool, "dup path"=w613:path)  [unwired: 8 in, 1 out]
            n444 = case shown="False" w612 {
              tunnel: w613 -> [w653 w656]
              tunnel: [w653 w656] -> w614
              frame False {
                n445 = local read "AVS names"() -> (w652:T5)
                n446 = local read "CS Names"() -> (w651:T20)
                n447 = control-ref of="Thermometer"() -> (w655:refnum<vi>)
                n448 = property on="Run description" class="Str"() -> ("Value"=w648:string)  [unwired: 2 in, 2 out]
                n449 = Cluster To Array(cluster=w652) -> (array=w649:string[])
                n450 = Cluster To Array(cluster=w651) -> (array=w650:string[])
                n451 = call "Format log file header Z.vi"("Thermometer"=w655, "AVS names"=w649, "CS Names"=w650, "Run description"=w648) -> ("String"=w654:string)  [unwired: 1 in]
                n452 = Write to Text File(file (use dialog)=w653, text=w654) -> ()  [unwired: 2 in, 3 out]
              }
              frame True {
              }
            }
            n453 = Get Date/Time In Seconds() -> (seconds since 1Jan1904=w628:timestamp)
            n454 = To Double Precision Float(number=w628) -> (double precision float=w626:dbl)
            n455 = Number To Exponential String(number=w626, precision (6)=i16 10) -> (E-format string=w627:string)  [unwired: 2 in]
            n456 = Format Date/Time String(time format string (%c)=w635, seconds (now)=w628) -> (date/time string=w632:string)  [unwired: 1 in]
            n457 = Number To Exponential String(number=w597) -> (E-format string=w634:string[])  [unwired: 3 in]
            n458 = Number To Engineering String(4:w596) -> (0:w633:string[])  [unwired: 3 in]
            n459 = Number To Fractional String(number=w595) -> (F-format string=w631:string[])  [unwired: 3 in]
            n460 = call "File Info__ogtk.vi"("file"=w614) -> ("file info"=w610:T43, "file out"=w619:path)  [unwired: 5 in, 1 out]
            n461 = Unbundle By Name(w610) -> ("creation date"=w611:u32)
            n462 = Build Array (concatenate)(w632, w627, w634, w633, w631) -> (w630:string[])
            n463 = local read "Calib path"() -> (w620:path)
            n464 = property on="NewFevery" class="DigNum (strict)"() -> ("Value"=w615:u32)  [unwired: 2 in, 2 out]
            n465 = property on="Time Units" class="Enum (strict)"() -> ("Value"=w616:enum16{"Minutes", "Hours", "Days"})  [unwired: 2 in, 2 out]
            n466 = property on="Thermometer" class="Clust (strict)"() -> ("Controls[]"=w594:refnum<vi>[])  [unwired: 2 in, 2 out]
            n467 = To Time Stamp(1:w611) -> (0:w617:timestamp)
            n468 = call "Time Elapsed time.vi"("Time Units"=w616, "Delay Time"=w615, "Time Old In"=w617) -> ("T>dT?"=w618:bool)  [unwired: 2 out]
            n469 = local read "Bridge settings"() -> (w598:T25)
            n470 = case shown="True" w618 {
              tunnel: [w638 w641] -> w609
              tunnel: [w637 w643] -> _
              tunnel: w619 -> [w638 _]
              tunnel: w620 -> [w637 _]
              frame False {
              }
              frame True {
                n471 = local read "Data logging"() -> (w644:T27)
                n472 = Unbundle By Name(w644) -> ("Run description"=w640:string, "Filenames suffix"=w642:string, "AVS_Path"=w647:path, "AVS_FName"=w645:string, "CAL_FName"=w646:string)
                n473 = call "MGI Make String Filesafe.vi"("String In"=w640) -> ("Filesafe String Out"=w639:string)
                n474 = call "GeneratePaths.vi"("Filename Suffix"=w642, "Run description"=w639, "AVS_Path"=w647, "AVS_FName"=w645, "CAL_Path"=w647, "CAL_FName"=w646) -> ("Generated Log path"=w641:path, "Generated Calib path"=w643:path)  [unwired: 8 in]
                n475 = local write "Calib path"(w643) -> ()
                n476 = property on="Log path" class="Path"("Val(Sgnl)"=w641) -> ()  [unwired: 2 in, 2 out]
              }
            }
            n477 = local read "Name"() -> (w591:string)
            n478 = Unbundle By Name(w598) -> ("AVS type"=w592:T35)
            n479 = call <userlib>:"ParseLeidenComputerNames.vi"("AVS type"=w592, "computer name"=w591) -> ("AVS Type"=w593:T44)  [unwired: 7 in, 2 out]
            n480 = call "Write To Spreadsheet File (string) w Error.vi"("delimiter (\\t)"=w636, "append to file? (new file:F)"=TRUE, "1D data"=w630, "file path (dialog if empty)"=w609) -> ("error out"=w624:errorcluster)  [unwired: 6 in, 1 out]
            n481 = property on="AVS names" class="Clust (strict)"() -> ("Value"=w599:T5)  [unwired: 2 in, 2 out]
            n482 = call <userlib>:"TC_to_DSC.vi"("AVS names"=w599, "AVS Type"=w593, "Array"=w594, "I"=w595, "T"=w596, "R"=w597) -> ()  [unwired: 6 in]
            n483 = Merge Errors(w624, w623) -> (w622:errorcluster)
          }
        }
      }
      event User Event {
        # "Current source automatic mode"
        # "Check if PID error (SP-PV)==0"
        # "Check if temperature\nis stabilized"
        # "Check if any channel\nis in automatic mode"
        # "Check if stabilization delay time \nis elapsed"
        # "T sabilized?"
        # "If TCS auto mode enabled and temperature is not changing => fire TempStabilized event to save log and set new CS point. Otherwise do PID (if enabled)."
        n484 = event-data() -> ("R/T"=w666:dbl, "Time"=w667:dbl)  [unwired: 1 in, 4 out]
        n485 = local read "I_list[i]"() -> (w660:dbl[])
        n486 = local read "Error"() -> (w670:dbl)
        n487 = property on="N averages" class="DigNum (strict)"() -> ("Value"=w663:i32)  [unwired: 2 in, 2 out]
        n488 = property on="FB to" class="Enum (strict)"() -> ("Value"=w659:enum16{"0", "1", "2", "3"})  [unwired: 2 in, 2 out]
        n489 = local read "Time Old"() -> (w676:dbl)
        n490 = local read "CS Mode"() -> (w658:enum16{"Manual", "Automatic"})
        n491 = property on="T stability" class="DigNum (strict)"() -> ("Value"=w661:dbl)  [unwired: 2 in, 2 out]
        n492 = Equal To 0?(x=w670) -> (x = 0?=w668:bool)
        n493 = property on="Delay Time" class="DigNum (strict)"() -> ("Value"=w662:dbl)  [unwired: 2 in, 2 out]
        n494 = Index Array(array=w660, index=w659) -> (element=w677:dbl)
        n495 = Not Equal To 0?(x=w658) -> (x != 0?=w657:bool)
        n496 = call "Derivatives Pt by Pt.vi"("Points to avg"=w663, "accuracy (%)"=w661, "Time"=w667, "Data"=w666) -> ("Stable?"=w669:bool, "Stability (%)"=→"Slope":dbl, "dt (s)"=w673:dbl)  [unwired: 3 in]
        n497 = call "Time Elapsed dbl.vi"("Delay Time"=w662, "Time Old In"=w676) -> ("T>dT?"=w665:bool, "Delta T"=→"Timer":dbl, "Time New Out"=w675:dbl)  [unwired: 1 in]
        n498 = Compound Arithmetic op=AND(w665, w657, w668, w669) -> (w671:bool)
        "SP reached?" <- w671
        n499 = property on="Enable PID" class="Bool (strict)"() -> ("Value"=w664:bool)  [unwired: 2 in, 2 out]
        n500 = case shown="False" w671 {
          tunnel: w675 -> [_ w694]
          tunnel: w673 -> [w692 _]
          tunnel: w666 -> [w686 _]
          tunnel: w664 -> [w684 _]
          tunnel: w677 -> [w685 _]
          tunnel: w660 -> [w681 _]
          tunnel: w659 -> [w680 _]
          tunnel: w657 -> [w678 _]
          frame False {
            # "Temperature is not stable. If enabled, do PID regulation"
            n501 = And(x=w684, y=w678) -> (x .and. y?=w679:bool)
            n502 = local read "PID setup 2"() -> (w689:T32)
            n503 = property on="I_0" class="DigNum (strict)"() -> ("Value"=w690:dbl)  [unwired: 2 in, 2 out]
            n504 = call "PID control incremental.vi"("Process Variable"=w686, "dt"=w692, "Setpoint"=w685, "PID Settings"=w689, "I in"=w690, "PID Enabled"=w679) -> ("err out"=→"Error":dbl, "int out"=→"Int":dbl, "I out"=w683:dbl)  [unwired: 10 in, 1 out]
            n505 = Bundle("Numeric"=w685, "R/T"=w686) -> (→"PID-Plot":cluster{"Numeric":dbl, "R/T":dbl})  [unwired: 1 in]
            n506 = Replace Array Subset(array=w681, new element=w683, index=w680) -> (→"I_in":dbl[])
          }
          frame True {
            # "Temperature is stable & automode is on"
            n507 = case shown="False" "Call external VI" {
              tunnel: w694 -> [w697 _]
              frame False {
                # "External VI call disabled -> proceed\nwith automode"
                n508 = local write "Time Old"(w697) -> ()
                n509 = property on="TempStabilized" class="TypRef (strict)"() -> ("Value"=w696:refnum<user-event>)  [unwired: 2 in, 2 out]
                n510 = Generate User Event(user event=w696, event data cluster=TRUE ("event data")) -> ()  [unwired: 2 in, 2 out]
              }
              frame True {
                # "Call external VI"
                n511 = property on="CallExtVI" class="TypRef (strict)"() -> ("Value"=w698:refnum<user-event>)  [unwired: 2 in, 2 out]
                n512 = Generate User Event(user event=w698, event data cluster="" ("event data")) -> ()  [unwired: 2 in, 2 out]
              }
            }
          }
        }
      }
      event User Event {
        n513 = event-data() -> ()  [unwired: 1 in, 5 out]
        n514 = local read "vi reference"() -> (w703:refnum<vi>)
        n515 = call "GetExtVIStatus.vi"("vi reference in"=w703) -> ("vi reference out"=w700:refnum<vi>, "Exec.State"=w702:T30, "Finished?"=w701:bool)
        n516 = case shown="\"Idle\"" w702 {
          tunnel: w701 -> [_ _]
          tunnel: w700 -> [_ w704]
          frame "Bad", Default {
          }
          frame "Idle" {
            n517 = local read "VI called?"() -> (w705:bool)
            n518 = case shown="True" w705 {
              tunnel: w704 -> [w707 _]
              frame False {
                n519 = property on="Data array" class="Arr (strict)"() -> ("Value"=w710:dbl[])  [unwired: 2 in, 2 out]
                n520 = property on="T_array" class="Arr (strict)"() -> ("Value"=w711:dbl[])  [unwired: 2 in, 2 out]
                n521 = property on="I" class="Arr (strict)"() -> ("Value"=w712:dbl[])  [unwired: 2 in, 2 out]
                n522 = Format Date/Time String() -> (date/time string=w709:string)  [unwired: 3 in]
                n523 = Bundle("date/time string"=w709, "Value"=w710, "Value"=w711, "Value"=w712) -> (w708:T47)  [unwired: 1 in]
                n524 = call "CallExtVI.vi"("vi reference in"=w707, "Cluster"=w708) -> ()  [unwired: 1 out]
                "VI called?" <- TRUE ("VI called?")
              }
              frame True {
                n525 = property on="TempStabilized" class="TypRef (strict)"() -> ("Value"=w714:refnum<user-event>)  [unwired: 2 in, 2 out]
                n526 = Get Date/Time In Seconds() -> (seconds since 1Jan1904=w715:timestamp)
                n527 = To Double Precision Float(number=w715) -> (double precision float=w716:dbl)
                n528 = Generate User Event(user event=w714, event data cluster=TRUE ("event data")) -> ()  [unwired: 2 in, 2 out]
                n529 = local write "Time Old"(w716) -> ()
              }
            }
          }
        }
      }
      event User Event {
        # "CS automode\nT is stabilized"
        n530 = event-data() -> ("TempStabilized"=w717:bool)  [unwired: 1 in, 4 out]
        n531 = stacked-sequence {
          tunnel: w719 -> [w725 _]
          tunnel: [w726 _] -> w718
          tunnel: w717 -> [_ w746]
          frame #0 {
            # "Step1: Save R,T,I values to calibration file. Make screenshot when creating the calibration file."
            n532 = property on="Calib path" class="Path"() -> ("Value"=w721:path)  [unwired: 2 in, 2 out]
            n533 = call "File Exists__ogtk.vi"("file path"=w721) -> ("exists"=w722:bool)  [unwired: 6 in, 1 out]
            n534 = case shown="False" w722 {
              tunnel: w721 -> [w735 w745]
              tunnel: [w735 w745] -> w720
              frame False {
                n535 = local read "AVS names"() -> (w742:T5)
                n536 = local read "CS Names"() -> (w741:T20)
                n537 = control-ref of="Thermometer"() -> (w744:refnum<vi>)
                n538 = property on="Run description" class="Str"() -> ("Value"=w738:string)  [unwired: 2 in, 2 out]
                n539 = Cluster To Array(cluster=w742) -> (array=w739:string[])
                n540 = Cluster To Array(cluster=w741) -> (array=w740:string[])
                n541 = call "Format log file header Z.vi"("Thermometer"=w744, "AVS names"=w739, "CS Names"=w740, "Run description"=w738) -> ("String"=w743:string)  [unwired: 1 in]
                n542 = Write to Text File(file (use dialog)=w735, text=w743) -> ()  [unwired: 2 in, 3 out]
                n543 = control-ref of="This VI"() -> (w737:refnum<vi>)
                n544 = invoke class="VI" method="FP.Get Image"(reference=w737) -> ("image data"=w736:T48)  [unwired: 5 in, 5 out]
                n545 = call "Convert File Extension (Path)__ogtk.vi"("new ending (none)"="png" ("name or relative path"), "file name"=w735) -> ("new filename"=w734:path)  [unwired: 1 out]
                n546 = call <vilib>:"Write PNG File.vi"("image data"=w736, "path to PNG file"=w734) -> ()  [unwired: 8 in, 2 out]
              }
              frame True {
              }
            }
            n547 = local write "VI called?"(FALSE ("VI called?")) -> ()
            n548 = property on="Data logging" class="Clust (strict)"() -> ("Value"=w729:T27)  [unwired: 2 in, 2 out]
            n549 = Unbundle By Name(w729) -> ("Date/Time Format"=w730:string, "Delimeter"=w727:string)
            n550 = property on="R" class="Clust (strict)"() -> ("Value"=w728:T8)  [unwired: 2 in, 2 out]
            n551 = property on="T" class="Clust (strict)"() -> ("Value"=w732:T4)  [unwired: 2 in, 2 out]
            n552 = property on="I" class="Arr (strict)"() -> ("Value"=w731:dbl[])  [unwired: 2 in, 2 out]
            n553 = call "Write to cal log file.vi"("Value 2"=w731, "Date/Time Format"=w730, "Value 3"=w732, "Value"=w728, "Delimeter"=w727, "Value 4"=w720) -> ("error out"=w724:errorcluster)  [unwired: 1 out]
            n554 = Merge Errors(w724, w725) -> (w726:errorcluster)
          }
          frame #1 {
            # "Step 2: Sweep through the currents list"
            n555 = case shown="True" w746 {
              frame False {
              }
              frame True {
                n556 = local read "I_list_idx_max"() -> (w748:i32)
                n557 = local read "I_list_idx"() -> (w749:i32)
                n558 = Less?(x=w749, y=w748) -> (x < y?=w747:bool)
                n559 = case shown="False" w747 {
                  frame False {
                    n560 = property on="CS Mode" class="Enum (strict)"("Val(Sgnl)"=enum16{"Manual", "Automatic"}."Manual" ("Value (Signaling)")) -> ()  [unwired: 2 in, 2 out]
                  }
                  frame True {
                    n561 = property on="I_next" class="Bool (strict)"("Val(Sgnl)"=TRUE) -> ()  [unwired: 2 in, 2 out]
                  }
                }
              }
            }
          }
        }
      }
      event User Event {
        # "Disable controls for disabled channels"
        n562 = event-data() -> ()  [unwired: 1 in, 5 out]
        n563 = property on="AVS type" class="Enum (strict)"() -> ("Value"=w759:T35)  [unwired: 2 in, 2 out]
        n564 = case shown="\"Impedance Bridge\"" w759 {
          tunnel: [w769 w780 w789] -> w758
          frame Default {
            n565 = property on="AVS Runtime Settings" class="Clust (strict)"() -> ("Value"=w773:T17)  [unwired: 2 in, 2 out]
            n566 = Unbundle By Name(w773) -> ("Read AVS channels from"=w771:i8, "Last Channel"=w772:i8)
            n567 = for {
              N: 10 -> [_]
              tunnel: w772 -> [w775]
              tunnel: w771 -> [w776]
              tunnel: [w774] -> w769 mode=indexing
              i -> [w777]
              n568 = Less Or Equal?(x=w776, y=w777) -> (x <= y?=w779:bool)
              n569 = Less Or Equal?(x=w777, y=w775) -> (x <= y?=w778:bool)
              n570 = And(x=w779, y=w778) -> (x .and. y?=w774:bool)
            }
          }
          frame "Impedance Bridge" {
            n571 = local read "zDll"() -> (w781:path)
            n572 = for {
              N: 10 -> [_]
              tunnel: [w784] -> w782 mode=indexing
              tunnel: w781 -> [w785]
              i -> [w787]
              n573 = call "GetByteParam.vi"("ParNo"=u8 0, "SetNo"=w787, "zDll"=w785) -> ("return type"=w784:u8)  [unwired: 6 in, 2 out]
            }
            n574 = Greater Than 0?(x=w782) -> (x > 0?=w780:bool[])
          }
          frame "AVS47B (RS232 interface)" {
            n575 = local read "Active"() -> (w788:T12)
            n576 = Cluster To Array(cluster=w788) -> (array=w789:bool[])
          }
        }
        n577 = control-ref of="Active"() -> (w765:refnum<vi>)
        n578 = control-ref of="Exc&Ranges"() -> (w761:refnum<vi>)
        n579 = control-ref of="R"() -> (w766:refnum<vi>)
        n580 = control-ref of="Thermometer"() -> (w767:refnum<vi>)
        n581 = control-ref of="T"() -> (w768:refnum<vi>)
        n582 = control-ref of="uPlots"() -> (w762:refnum<vi>)
        n583 = control-ref of="AVS names"() -> (w760:refnum<vi>)
        n584 = control-ref of="zBridge params"() -> (w757:refnum<vi>)
        n585 = control-ref of="Status"() -> (w756:refnum<vi>)
        n586 = control-ref of="Units"() -> (w755:refnum<vi>)
        n587 = control-ref of="AVS names small"() -> (w754:refnum<vi>)
        n588 = control-ref of="Small R"() -> (w753:refnum<vi>)
        n589 = control-ref of="Small T"() -> (w752:refnum<vi>)
        n590 = Build Array(w765, w761, w766, w767, w768, w762, w760, w757, w756, w755, w754, w753, w752) -> (w763:refnum<vi>[])
        n591 = Array Size(array=w763) -> (size(s)=w764:i32)
        n592 = for {
          N: w764 -> [_]
          tunnel: w763 -> [w793] mode=indexing
          tunnel: w758 -> [w790]
          n593 = property class="Clust"(reference=w793) -> ("Controls[]"=w791:refnum<vi>[])  [unwired: 1 in, 2 out]
          n594 = Array Size(array=w791) -> (size(s)=w792:i32)
          n595 = for {
            N: w792 -> [_]
            tunnel: w791 -> [w795] mode=indexing
            tunnel: w790 -> [w794] mode=indexing
            n596 = case shown="True" w794 {
              tunnel: w795 -> [w796 w801]
              frame False {
                n597 = property class="Ctl"(reference=w796, "Disabled"=u8 2) -> ("ClassName"=w797:string)  [unwired: 1 in, 2 out]
                n598 = case shown="\"Boolean\"" w797 {
                  tunnel: w796 -> [_ w800 _]
                  frame "False", Default {
                  }
                  frame "Boolean" {
                    n599 = property class="Ctl"(reference=w800, "Value"=FALSE) -> ()  [unwired: 1 in, 2 out]
                  }
                  frame "Ring" {
                  }
                }
              }
              frame True {
                n600 = property class="Ctl"(reference=w801, "Disabled"=u8 0) -> ("ClassName"=w802:string)  [unwired: 1 in, 2 out]
                n601 = case shown="\"Boolean\"" w802 {
                  tunnel: w801 -> [_ w805]
                  frame "False", Default {
                  }
                  frame "Boolean" {
                    n602 = property class="Ctl"(reference=w805, "Value"=TRUE) -> ()  [unwired: 1 in, 2 out]
                  }
                }
              }
            }
          }
        }
      }
      event "Log path": Value Change {
        # "Modify window title to show measurement information"
        n603 = event-data() -> ("NewVal"=w812:path)  [unwired: 1 in, 5 out]
        n604 = property on="Run description" class="Str"() -> ("Value"=w806:string)  [unwired: 2 in, 2 out]
        n605 = property on="AVS type" class="Enum (strict)"() -> ("RingText.Text"=w807:string)  [unwired: 2 in, 2 out]
        n606 = property on="CS type" class="Enum (strict)"() -> ("RingText.Text"=w810:string)  [unwired: 2 in, 2 out]
        n607 = Path To String(path=w812) -> (string=w809:string)
        n608 = Format Into String(format string="%s - %s - %s   (%s)", w806, w807, w810, w809) -> (resulting string=w808:string)  [unwired: 2 in, 1 out]
        n609 = control-ref of="This VI"() -> (w813:refnum<vi>)
        n610 = property class="VI"(reference=w813, "Front Panel.Title"=w808) -> ()  [unwired: 1 in, 2 out]
      }
      event "Refresh Calibrations", "Bridge settings.AVS_CalFolder": Value Change; User Event {
        # "Refresh the list of calibration files"
        n611 = event-data() -> ()  [unwired: 1 in, 3 out]
        n612 = control-ref of="Thermometer"() -> (w820:refnum<vi>)
        n613 = control-ref of="CurCalibrations"() -> (w814:refnum<vi>)
        n614 = control-ref of="AVS_CalFolder"() -> (w818:refnum<vi>)
        n615 = control-ref of="Select sensor 1"() -> (w819:refnum<vi>)
        n616 = control-ref of="Select sensor 1"() -> (w817:refnum<vi>)
        n617 = call "ReloadCalibrations.vi"("error in (no error)"=w816, "Quick convert sensors"=w817, "CurCalibrations"=w814, "Calibration files path"=w818, "Channel1 sensors"=w819, "Channels list"=w820) -> ("error out"=w815:errorcluster)  [unwired: 1 in]
      }
      event "Mode Buttons": Value Change {
        w826 = refnum<vi> refnum  # XYGraph
        # "Show cursor on plot is \"Cursor\" or \"Delete points\" mode is enabled"
        # "!!NOTE:This routine assumes that XY graph is control #0 on tab page!!"
        n618 = event-data() -> ("NewVal"=w822:T13)  [unwired: 1 in, 5 out]
        n619 = property on="Channel Controls" class="TabCtl (strict)"() -> ("Pages"=w830:refnum<vi>[], "Value"=w829:T3)  [unwired: 2 in, 2 out]
        n620 = Index Array(array=w830, index=w829) -> (element=w828:refnum<vi>)
        n621 = property class="Page"(reference=w828) -> ("ControlsOnPage"=w823:refnum<vi>[])  [unwired: 1 in, 2 out]
        n622 = Index Array(array=w823, index=0) -> (element=w827:refnum<vi>)
        n623 = Type Cast(type=w826, x=w827) -> (*(type *) &x=w821:refnum<vi>)
        n624 = case shown="\"Erase Range\"" w822 {
          tunnel: w821 -> [w831 w840 w848 w856]
          frame "No Selection", Default {
            n625 = property class="XYGraph"(reference=w831, "Active Cursor"=u32 0, "Cursor.Visible"=FALSE) -> (reference out=w834:refnum<vi>)  [unwired: 1 in, 1 out]
            n626 = property class="XYGraph"(reference=w834, "Active Cursor"=u32 1, "Cursor.Visible"=FALSE) -> ()  [unwired: 1 in, 2 out]
          }
          frame "Erase Range" {
            n627 = property class="XYGraph"(reference=w840, "Active Cursor"=u32 0, "Cursor.Visible"=TRUE, "Cursor.Cursor Color"=u32 16777062, "Cursor.Cursor Index"=0, "ActPaletteTool"=0 ("Palette:Active Tool")) -> (reference out=w843:refnum<vi>)  [unwired: 1 in, 1 out]
            n628 = property class="XYGraph"(reference=w843, "Active Cursor"=u32 1, "Cursor.Visible"=TRUE, "Cursor.Cursor Color"=u32 6618880) -> ()  [unwired: 1 in, 2 out]
          }
          frame "Cursor Mode" {
            n629 = property class="XYGraph"(reference=w848, "Active Cursor"=u32 0, "Cursor.Visible"=TRUE, "Cursor.Cursor Color"=u32 6618880, "ActPaletteTool"=0 ("Palette:Active Tool")) -> (reference out=w851:refnum<vi>)  [unwired: 1 in, 1 out]
            n630 = property class="XYGraph"(reference=w851, "Active Cursor"=u32 1, "Cursor.Visible"=FALSE) -> ()  [unwired: 1 in, 2 out]
          }
          frame "Erase point" {
            n631 = property class="XYGraph"(reference=w856, "Active Cursor"=u32 0, "Cursor.Visible"=TRUE, "Cursor.Cursor Color"=u32 16777062, "ActPaletteTool"=0 ("Palette:Active Tool")) -> (reference out=w859:refnum<vi>)  [unwired: 1 in, 1 out]
            n632 = property class="XYGraph"(reference=w859, "Active Cursor"=u32 1, "Cursor.Visible"=FALSE) -> ()  [unwired: 1 in, 2 out]
          }
        }
      }
      event "R-Plot 0", "R-Plot 1", "R-Plot 2", "R-Plot 3", "R-Plot 4", "R-Plot 5", "R-Plot 6", "R-Plot 7", "R-Plot 8", "R-Plot 9": Mouse Down? {
        # "Disabled"
        n633 = event-data() -> ("CtlRef"=w864:refnum<vi>, "Button"=w869:u16, "Mods.Double Click"=w866:bool)  [unwired: 1 in, 5 out]
        n634 = Equal?(x=u16 1, y=w869) -> (x = y?=w867:bool)
        n635 = And(x=w867, y=w866) -> (x .and. y?=w865:bool)
        n636 = disable-structure shown="Disabled" {
          disable-tunnel: w865 -> [w872 _]
          disable-tunnel: w864 -> [w871 _]
          disable-tunnel: "Mode Buttons" -> [w870 _]
          frame Disabled {
            n637 = case shown="True" w872 {
              tunnel: w870 -> [_ w874]
              tunnel: w871 -> [_ w873]
              frame False {
              }
              frame True {
                n638 = case shown="\"Erase Range\"" w874 {
                  tunnel: w873 -> [_ w875]
                  frame "No Selection", Default {
                  }
                  frame "Erase Range" {
                    n639 = property class="XYGraph (strict)"(reference=w875, "ActPaletteTool"=0 ("Palette:Active Tool"), "Active Cursor"=u32 0, "Cursor.Visible"=TRUE) -> ()  [unwired: 1 in, 2 out]
                  }
                }
              }
            }
          }
          frame Enabled {
          }
        }
        n640 = event-data() -> ()  [unwired: 5 in, 1 out]
      }
      event "R-Plot 0", "R-Plot 1", "R-Plot 2", "R-Plot 3", "R-Plot 4", "R-Plot 5", "R-Plot 6", "R-Plot 7", "R-Plot 8", "R-Plot 9": Mouse Down {
        # "Process (double) click on plots in special modes (\"Cursor\", \"Erase\")"
        n641 = event-data() -> ("CtlRef"=w880:refnum<vi>, "Coords"=w883:T49, "Button"=w879:u16, "Mods.Double Click"=w882:bool)  [unwired: 1 in, 4 out]
        n642 = property on="Mode Buttons" class="RadioBtnsControl (strict)"() -> ("Value"=w881:T13)  [unwired: 2 in, 2 out]
        n643 = case shown="1" w879 {
          tunnel: w883 -> [_ w917]
          tunnel: w882 -> [_ w916]
          tunnel: w881 -> [w888 w915]
          tunnel: w880 -> [w889 w914]
          frame 0, Default {
            n644 = local read "LMB Down"() -> (w886:bool)
            n645 = Equal?(x=w888, y=T13."Erase Range" ("Mode Buttons")) -> (x = y?=w887:bool)
            n646 = And(x=w886, y=w887) -> (x .and. y?=w885:bool)
            n647 = case shown="True" w885 {
              tunnel: w889 -> [_ w912]
              frame False {
              }
              frame True {
                n648 = property class="XYGraph (strict)"(reference=w912, "Active Cursor"=u32 0, "Active Cursor"=u32 1) -> ("Cursor.Cursor X"=w909:dbl, "Cursor.Cursor X"=w890:dbl)  [unwired: 1 in, 2 out]
                n649 = local read "Channel Controls"() -> (w911:T3)
                n650 = local read "Data"() -> (w906:cluster{"R":dbl[], "T":dbl[], "Time":dbl[]}[])
                n651 = Max & Min(x=w909, y=w890) -> (max(x,y)=w899:dbl, min(x,y)=w892:dbl)
                n652 = Index Array(array=w906, index=w911) -> (element=w902:cluster{"R":dbl[], "T":dbl[], "Time":dbl[]})
                n653 = Unbundle By Name(w902) -> ("R"=w900:dbl[], "T"=w901:dbl[], "Time"=w898:dbl[])
                n654 = Threshold 1D Array(2:w899, 3:w898) -> (0:w896:dbl)  [unwired: 1 in]
                n655 = Threshold 1D Array(2:w892, 3:w898) -> (0:w897:dbl)  [unwired: 1 in]
                n656 = Subtract(x=w896, y=w897) -> (x-y=w895:dbl)
                n657 = Delete From Array(array=w900, length=w895, index=w897) -> (array with subset deleted=w905:dbl[])  [unwired: 1 out]
                n658 = Delete From Array(array=w901, length=w895, index=w897) -> (array with subset deleted=w904:dbl[])  [unwired: 1 out]
                n659 = Delete From Array(array=w898, length=w895, index=w897) -> (array with subset deleted=w903:dbl[])  [unwired: 1 out]
                n660 = Bundle By Name(cluster=w902, "R"=w905, "T"=w904, "Time"=w903) -> (w907:cluster{"R":dbl[], "T":dbl[], "Time":dbl[]})
                n661 = Replace Array Subset(array=w906, new element=w907, index=w911) -> (w908:cluster{"R":dbl[], "T":dbl[], "Time":dbl[]}[])
                n662 = local write "Data"(w908) -> ()
                n663 = property class="XYGraph (strict)"(reference=w912, "Active Cursor"=u32 0, "Cursor.Cursor X"=w892, "Active Cursor"=u32 1, "Cursor.Cursor X"=w892) -> ()  [unwired: 1 in, 2 out]
              }
            }
          }
          frame 1 {
            n664 = case shown="\"Cursor Mode\"" w915 {
              tunnel: w914 -> [_ w920 w941 w949]
              tunnel: w917 -> [_ w919 w940 w951]
              tunnel: w916 -> [_ w918 w942 w950]
              frame "No Selection", Default {
              }
              frame "Cursor Mode" {
                n665 = case shown="True" w918 {
                  tunnel: w920 -> [_ w930]
                  tunnel: w919 -> [_ w928]
                  frame False {
                  }
                  frame True {
                    n666 = invoke class="XYGraph (strict)" method="Map Coords To XY"(reference=w930, "Coords"=w928) -> (reference out=w929:refnum<vi>, "XY"=w927:cluster{"X":dbl, "Y":dbl})  [unwired: 5 in, 5 out]
                    n667 = Unbundle By Name(w927) -> ("X"=w925:dbl)
                    n668 = local read "Data"() -> (w926:cluster{"R":dbl[], "T":dbl[], "Time":dbl[]}[])
                    n669 = property class="XYGraph (strict)"(reference=w929, "Active Cursor"=u32 0, "Cursor.Cursor Position"=w927) -> ()  [unwired: 1 in, 2 out]
                    n670 = for {
                      tunnel: w926 -> [w939] mode=indexing
                      tunnel: w925 -> [w937]
                      tunnel: [w933] -> w924 mode=indexing
                      tunnel: [w932] -> w923 mode=indexing
                      n671 = Unbundle By Name(w939) -> ("R"=w936:dbl[], "T"=w935:dbl[], "Time"=w938:dbl[])
                      n672 = Threshold 1D Array(2:w937, 3:w938) -> (0:w934:dbl)  [unwired: 1 in]
                      n673 = Index Array(array=w936, index=w934) -> (element=w933:dbl)
                      n674 = Index Array(array=w935, index=w934) -> (element=w932:dbl)
                    }
                    n675 = Array To Cluster(array=w923) -> (cluster=w921:T41)
                    n676 = Array To Cluster(array=w924) -> (cluster=w922:T41)
                    n677 = property on="Time" class="DigNum (strict)"("Value"=w925) -> ()  [unwired: 2 in, 2 out]
                    n678 = property on="Small R" class="Clust (strict)"("Value"=w922) -> ()  [unwired: 2 in, 2 out]
                    n679 = property on="Small T" class="Clust (strict)"("Value"=w921) -> ()  [unwired: 2 in, 2 out]
                  }
                }
              }
              frame "Erase Range" {
                n680 = case shown="False" w942 {
                  tunnel: w941 -> [w946 _]
                  tunnel: w940 -> [w945 _]
                  frame False {
                    n681 = invoke class="XYGraph (strict)" method="Map Coords To XY"(reference=w946, "Coords"=w945) -> (reference out=w948:refnum<vi>, "XY"=w943:cluster{"X":dbl, "Y":dbl})  [unwired: 5 in, 5 out]
                    n682 = property class="XYGraph (strict)"(reference=w948, "Active Cursor"=u32 0, "Cursor.Cursor Position"=w943, "Active Cursor"=u32 1, "Cursor.Cursor Position"=w943) -> ()  [unwired: 1 in, 2 out]
                  }
                  frame True {
                  }
                }
              }
              frame "Erase point" {
                n683 = case shown="False" w950 {
                  tunnel: w949 -> [w956 w971]
                  tunnel: w951 -> [w955 _]
                  frame False {
                    n684 = invoke class="XYGraph (strict)" method="Map Coords To XY"(reference=w956, "Coords"=w955) -> (reference out=w954:refnum<vi>, "XY"=w953:cluster{"X":dbl, "Y":dbl})  [unwired: 5 in, 5 out]
                    n685 = property class="XYGraph (strict)"(reference=w954, "Active Cursor"=u32 0, "Cursor.Cursor Position"=w953) -> ()  [unwired: 1 in, 2 out]
                  }
                  frame True {
                    n686 = property class="XYGraph (strict)"(reference=w971, "Active Cursor"=u32 0) -> ("Cursor.Cursor X"=w958:dbl)  [unwired: 1 in, 2 out]
                    n687 = local read "Channel Controls"() -> (w957:T3)
                    n688 = local read "Data"() -> (w967:cluster{"R":dbl[], "T":dbl[], "Time":dbl[]}[])
                    n689 = Index Array(array=w967, index=w957) -> (element=w963:cluster{"R":dbl[], "T":dbl[], "Time":dbl[]})
                    n690 = Unbundle By Name(w963) -> ("R"=w959:dbl[], "T"=w960:dbl[], "Time"=w961:dbl[])
                    n691 = Threshold 1D Array(2:w958, 3:w961) -> (0:w962:dbl)  [unwired: 1 in]
                    n692 = Delete From Array(array=w959, index=w962) -> (array with subset deleted=w966:dbl[])  [unwired: 1 in, 1 out]
                    n693 = Delete From Array(array=w960, index=w962) -> (array with subset deleted=w965:dbl[])  [unwired: 1 in, 1 out]
                    n694 = Delete From Array(array=w961, index=w962) -> (array with subset deleted=w964:dbl[])  [unwired: 1 in, 1 out]
                    n695 = Bundle By Name(cluster=w963, "R"=w966, "T"=w965, "Time"=w964) -> (w968:cluster{"R":dbl[], "T":dbl[], "Time":dbl[]})
                    n696 = Replace Array Subset(array=w967, new element=w968, index=w957) -> (w969:cluster{"R":dbl[], "T":dbl[], "Time":dbl[]}[])
                    n697 = local write "Data"(w969) -> ()
                  }
                }
              }
            }
            "LMB Down" <- TRUE ("Mouse down")
          }
        }
      }
      event "R-Plot 0", "R-Plot 1", "R-Plot 2", "R-Plot 3", "R-Plot 4", "R-Plot 5", "R-Plot 6", "R-Plot 7", "R-Plot 8", "R-Plot 9": Mouse Move {
        # "Process mouse movement over plots in special modes (\"Cursor\", \"Erase\")"
        n698 = event-data() -> ("CtlRef"=w972:refnum<vi>, "Coords"=w973:T49)  [unwired: 1 in, 3 out]
        n699 = property on="Mode Buttons" class="RadioBtnsControl (strict)"() -> ("Value"=w977:T13)  [unwired: 2 in, 2 out]
        n700 = local read "LMB Down"() -> (w978:bool)
        n701 = Equal?(x=w977, y=T34."Erase Range") -> (x = y?=w974:bool)
        n702 = And(x=w978, y=w974) -> (x .and. y?=w975:bool)
        n703 = case shown="True" w975 {
          tunnel: w973 -> [_ w980]
          tunnel: w972 -> [_ w979]
          frame False {
          }
          frame True {
            n704 = invoke class="XYGraph (strict)" method="Map Coords To XY"(reference=w979, "Coords"=w980) -> (reference out=w983:refnum<vi>, "XY"=w982:cluster{"X":dbl, "Y":dbl})  [unwired: 5 in, 5 out]
            n705 = property class="XYGraph (strict)"(reference=w983, "Active Cursor"=u32 1, "Cursor.Cursor Position"=w982) -> ()  [unwired: 1 in, 2 out]
          }
        }
      }
      event "R-Plot 0", "R-Plot 1", "R-Plot 2", "R-Plot 3", "R-Plot 4", "R-Plot 5", "R-Plot 6", "R-Plot 7", "R-Plot 8", "R-Plot 9": Mouse Up {
        n706 = event-data() -> ("CtlRef"=w986:refnum<vi>, "Button"=w984:u16)  [unwired: 1 in, 6 out]
        n707 = property on="Mode Buttons" class="RadioBtnsControl (strict)"() -> ("Value"=w987:T13)  [unwired: 2 in, 2 out]
        n708 = property class="XYGraph (strict)"(reference=w986) -> ("ActPaletteTool"=w985:i32)  [unwired: 1 in, 2 out]
        n709 = case shown="1" w984 {
          tunnel: w987 -> [_ w991]
          tunnel: w986 -> [_ w990]
          tunnel: w985 -> [_ w989]
          frame 0, Default {
          }
          frame 1 {
            n710 = local write "LMB Down"(FALSE ("Mouse down")) -> ()
            n711 = case shown="Default" w989 {
              tunnel: w991 -> [_ _]
              tunnel: w990 -> [_ _]
              frame Default {
                n712 = property on="Mode Buttons" class="RadioBtnsControl (strict)"("Val(Sgnl)"=T13."No Selection" ("Value (Signaling)")) -> ()  [unwired: 2 in, 2 out]
              }
              frame 0 {
              }
            }
          }
        }
      }
      event "R-Plot 0", "R-Plot 1", "R-Plot 2", "R-Plot 3", "R-Plot 4", "R-Plot 5", "R-Plot 6", "R-Plot 7", "R-Plot 8", "R-Plot 9": Mouse Leave {
        n713 = event-data() -> ()  [unwired: 1 in, 4 out]
        n714 = local write "LMB Down"(FALSE ("Mouse down")) -> ()
      }
      event "R-Plot 0", "R-Plot 1", "R-Plot 2", "R-Plot 3", "R-Plot 4", "R-Plot 5", "R-Plot 6", "R-Plot 7", "R-Plot 8", "R-Plot 9": Scale Range Change {
        w995 = u8 0 ("X Scale.Scale Fit")
        # "Disable plot autoscaling if the user has changed the scale of the plot manualy"
        n715 = event-data() -> ("CtlRef"=w994:refnum<vi>)  [unwired: 1 in, 7 out]
        n716 = property class="XYGraph (strict)"(reference=w994, "XScale.ScaleFit"=w995, "YScale.ScaleFit"=w995) -> ()  [unwired: 1 in, 2 out]
      }
      event "R-Plot 0", "R-Plot 1", "R-Plot 2", "R-Plot 3", "R-Plot 4", "R-Plot 5", "R-Plot 6", "R-Plot 7", "R-Plot 8", "R-Plot 9": Shortcut Menu Activation? {
        w1003 = string[] ["Log Y"] ("item names")
        w1005 = string[] ["Zoom In to Last Data", "Autoscale XY"] ("item names")
        # "Add extra options to the plots context menu"
        n717 = event-data() -> ("MenuRef"=w1007:refnum<k9>, "CtlRef"=w999:refnum<vi>)  [unwired: 1 in]
        n718 = Insert Menu Items(4:10, 7:w1005, 8:w1005, 9:w1007) -> (3:w1001:refnum<k9>)  [unwired: 2 in, 2 out]
        n719 = property class="XYGraph (strict)"(reference=w999) -> ("YScale.Mapping Mode"=w998:u8)  [unwired: 1 in, 2 out]
        n720 = Insert Menu Items(4:14, 7:w1003, 8:w1003, 9:w1001) -> (3:w1000:refnum<k9>)  [unwired: 2 in, 2 out]
        n721 = Not Equal To 0?(x=w998) -> (x != 0?=w997:bool)
        n722 = Set Menu Item Info(6:w997, 7:"Log Y", 11:w1000) -> ()  [unwired: 4 in, 2 out]
        n723 = local read "LMB Down"() -> (w1004:bool)
        n724 = event-data("Discard?"=w1004) -> ()  [unwired: 1 in, 1 out]
      }
      event "R-Plot 0", "R-Plot 1", "R-Plot 2", "R-Plot 3", "R-Plot 4", "R-Plot 5", "R-Plot 6", "R-Plot 7", "R-Plot 8", "R-Plot 9": Shortcut Menu Selection (User) {
        # "Zoom in to last \"Miniplot points\". Zoom out a bit to have some space around the points"
        n725 = event-data() -> ("CtlRef"=w1011:refnum<vi>, "ItemTag"=w1009:string)  [unwired: 1 in]
        n726 = Type Cast(type=refnum<vi> refnum ("R-Plot 0"), x=w1011) -> (*(type *) &x=w1010:refnum<vi>)
        n727 = case shown="\"Zoom In to Last Data\"" w1009 {
          tunnel: w1010 -> [_ w1013 w1042 w1048]
          frame Default {
          }
          frame "Autoscale XY" {
            w1012 = u8 2 ("X Scale.Scale Fit")
            n728 = property class="XYGraph (strict)"(reference=w1013, "XScale.ScaleFit"=w1012, "YScale.ScaleFit"=w1012) -> ()  [unwired: 1 in, 2 out]
          }
          frame "Zoom In to Last Data" {
            w1038 = u8 0 ("Y Scale.Scale Fit")
            n729 = property on="AVS Runtime Settings" class="Clust (strict)"() -> ("Value"=w1037:T17)  [unwired: 2 in, 2 out]
            n730 = property class="XYGraph (strict)"(reference=w1042) -> (reference out=w1039:refnum<vi>, "Value"=w1041:cluster{dbl[], dbl[]})  [unwired: 1 in, 1 out]
            n731 = Unbundle By Name(w1037) -> ("Data Memory 2"=w1036:dbl)
            n732 = Unbundle(w1041) -> (w1015:dbl[], w1040:dbl[])
            n733 = Multiply(x=w1036, y=60.0) -> (x*y=w1032:dbl)
            n734 = Reverse 1D Array(array=w1015) -> (reversed array=w1020:dbl[])
            n735 = Reverse 1D Array(array=w1040) -> (reversed array=w1028:dbl[])
            n736 = Index Array(array=w1020) -> (element=w1034:dbl)  [unwired: 1 in]
            n737 = Multiply(x=0.5, y=w1032) -> (x*y=w1033:dbl)
            n738 = Add(x=w1033, y=w1034) -> (x+y=w1031:dbl)
            n739 = Subtract(x=w1034, y=w1032) -> (x-y=w1029:dbl)
            n740 = call "Improved Threshold Detector.71.vi"("Threshold"=w1029, "Array"=w1015) -> ("Positive transition indices"=w1016:i32[])  [unwired: 8 in, 1 out]
            n741 = Index Array(array=w1016) -> (element=w1043:i32)  [unwired: 1 in]
            n742 = Array Size(array=w1015) -> (size(s)=w1018:i32)
            n743 = Index Array(array=w1015, index=w1043) -> (element=w1014:dbl)
            n744 = Subtract(x=w1018, y=w1043) -> (x-y=w1017:i32)
            n745 = Array Subset(array=w1028, length=w1017) -> (w1027:dbl[])  [unwired: 1 in]
            n746 = Array Max & Min(array=w1027) -> (max value=w1024:dbl, min value=w1023:dbl)  [unwired: 2 out]
            n747 = Subtract(x=w1024, y=w1023) -> (x-y=w1026:dbl)
            n748 = Divide(x=w1026, y=2.0) -> (x/y=w1022:dbl)
            n749 = Add(x=w1024, y=w1022) -> (x+y=w1019:dbl)
            n750 = Subtract(x=w1023, y=w1022) -> (x-y=w1021:dbl)
            n751 = property class="XYGraph (strict)"(reference=w1039, "XScale.ScaleFit"=w1038, "YScale.ScaleFit"=w1038, "XScale.Maximum"=w1031, "XScale.Minimum"=w1014, "YScale.Maximum"=w1019, "YScale.Minimum"=w1021) -> ()  [unwired: 1 in, 2 out]
          }
          frame "Log Y" {
            n752 = property class="XYGraph (strict)"(reference=w1048) -> (reference out=w1047:refnum<vi>, "YScale.Mapping Mode"=w1046:u8)  [unwired: 1 in, 1 out]
            n753 = Equal To 0?(x=w1046) -> (x = 0?=w1045:bool)
            n754 = Boolean To (0,1)(Boolean=w1045) -> (0, 1=w1044:i16)
            n755 = property class="XYGraph (strict)"(reference=w1047, "YScale.Mapping Mode"=w1044) -> ()  [unwired: 1 in, 2 out]
          }
        }
      }
      event "PID-Plot": Shortcut Menu Activation? {
        w1056 = string[] ["Log Y"] ("item names")
        w1058 = string[] ["Autoscale XY"] ("item names")
        # "Add extra options to the plots context menu"
        n756 = event-data() -> ("MenuRef"=w1060:refnum<k9>, "CtlRef"=w1052:refnum<vi>)  [unwired: 1 in]
        n757 = Insert Menu Items(4:8, 7:w1058, 8:w1058, 9:w1060) -> (3:w1054:refnum<k9>)  [unwired: 2 in, 2 out]
        n758 = property class="WFChart (strict)"(reference=w1052) -> ("YScale.Mapping Mode"=w1051:u8)  [unwired: 1 in, 2 out]
        n759 = Insert Menu Items(4:11, 7:w1056, 8:w1056, 9:w1054) -> (3:w1053:refnum<k9>)  [unwired: 2 in, 2 out]
        n760 = Not Equal To 0?(x=w1051) -> (x != 0?=w1050:bool)
        n761 = Set Menu Item Info(6:w1050, 7:"Log Y", 11:w1053) -> ()  [unwired: 4 in, 2 out]
        n762 = local read "LMB Down"() -> (w1057:bool)
        n763 = event-data("Discard?"=w1057) -> ()  [unwired: 1 in, 1 out]
      }
      event "PID-Plot": Shortcut Menu Selection (User) {
        # "Zoom in to last \"Miniplot points\". Zoom out a bit to have some space around the points"
        n764 = event-data() -> ("CtlRef"=w1063:refnum<vi>, "ItemTag"=w1061:string)  [unwired: 1 in]
        n765 = Type Cast(type=refnum<vi> refnum ("R-Plot 0"), x=w1063) -> (*(type *) &x=w1062:refnum<vi>)
        n766 = case shown="\"Zoom In to Last Data\"" w1061 {
          tunnel: w1062 -> [_ w1066 w1095 w1101]
          frame Default {
          }
          frame "Autoscale XY" {
            w1065 = u8 2 ("X Scale.Scale Fit")
            n767 = property class="XYGraph (strict)"(reference=w1066, "XScale.ScaleFit"=w1065, "YScale.ScaleFit"=w1065) -> ()  [unwired: 1 in, 2 out]
          }
          frame "Zoom In to Last Data" {
            w1091 = u8 0 ("Y Scale.Scale Fit")
            n768 = property on="AVS Runtime Settings" class="Clust (strict)"() -> ("Value"=w1090:T17)  [unwired: 2 in, 2 out]
            n769 = property class="XYGraph (strict)"(reference=w1095) -> (reference out=w1092:refnum<vi>, "Value"=w1094:cluster{dbl[], dbl[]})  [unwired: 1 in, 1 out]
            n770 = Unbundle By Name(w1090) -> ("Data Memory 2"=w1089:dbl)
            n771 = Unbundle(w1094) -> (w1068:dbl[], w1093:dbl[])
            n772 = Multiply(x=w1089, y=60.0) -> (x*y=w1085:dbl)
            n773 = Reverse 1D Array(array=w1068) -> (reversed array=w1073:dbl[])
            n774 = Reverse 1D Array(array=w1093) -> (reversed array=w1081:dbl[])
            n775 = Index Array(array=w1073) -> (element=w1087:dbl)  [unwired: 1 in]
            n776 = Multiply(x=0.5, y=w1085) -> (x*y=w1086:dbl)
            n777 = Add(x=w1086, y=w1087) -> (x+y=w1084:dbl)
            n778 = Subtract(x=w1087, y=w1085) -> (x-y=w1082:dbl)
            n779 = call "Improved Threshold Detector.71.vi"("Threshold"=w1082, "Array"=w1068) -> ("Positive transition indices"=w1069:i32[])  [unwired: 8 in, 1 out]
            n780 = Index Array(array=w1069) -> (element=w1096:i32)  [unwired: 1 in]
            n781 = Array Size(array=w1068) -> (size(s)=w1071:i32)
            n782 = Index Array(array=w1068, index=w1096) -> (element=w1067:dbl)
            n783 = Subtract(x=w1071, y=w1096) -> (x-y=w1070:i32)
            n784 = Array Subset(array=w1081, length=w1070) -> (w1080:dbl[])  [unwired: 1 in]
            n785 = Array Max & Min(array=w1080) -> (max value=w1077:dbl, min value=w1076:dbl)  [unwired: 2 out]
            n786 = Subtract(x=w1077, y=w1076) -> (x-y=w1079:dbl)
            n787 = Divide(x=w1079, y=2.0) -> (x/y=w1075:dbl)
            n788 = Add(x=w1077, y=w1075) -> (x+y=w1072:dbl)
            n789 = Subtract(x=w1076, y=w1075) -> (x-y=w1074:dbl)
            n790 = property class="XYGraph (strict)"(reference=w1092, "XScale.ScaleFit"=w1091, "YScale.ScaleFit"=w1091, "XScale.Maximum"=w1084, "XScale.Minimum"=w1067, "YScale.Maximum"=w1072, "YScale.Minimum"=w1074) -> ()  [unwired: 1 in, 2 out]
          }
          frame "Log Y" {
            n791 = property class="XYGraph (strict)"(reference=w1101) -> (reference out=w1100:refnum<vi>, "YScale.Mapping Mode"=w1099:u8)  [unwired: 1 in, 1 out]
            n792 = Equal To 0?(x=w1099) -> (x = 0?=w1098:bool)
            n793 = Boolean To (0,1)(Boolean=w1098) -> (0, 1=w1097:i16)
            n794 = property class="XYGraph (strict)"(reference=w1100, "YScale.Mapping Mode"=w1097) -> ()  [unwired: 1 in, 2 out]
          }
        }
      }
      event "uPlots.uPlot 0", "uPlots.uPlot 1", "uPlots.uPlot 2", "uPlots.uPlot 3", "uPlots.uPlot 4", "uPlots.uPlot 5", "uPlots.uPlot 6", "uPlots.uPlot 7", "uPlots.uPlot 8", "uPlots.uPlot 9": Mouse Down {
        # "Switch to big plot on double click on small plot"
        n795 = event-data() -> ("Mods.Double Click"=w1103:bool, "CtlRef"=w1102:refnum<vi>)  [unwired: 1 in]
        n796 = case shown="True" w1103 {
          tunnel: w1102 -> [_ w1106]
          frame False {
          }
          frame True {
            n797 = property class="XYGraph (strict)"(reference=w1106) -> ("Label.Text"=w1107:string)  [unwired: 1 in, 2 out]
            n798 = Reverse String(1:w1107) -> (0:w1108:string)
            n799 = Decimal String To Number(string=w1108, default (0L)=8 ("default (0 I32)")) -> (number=w1105:i32)  [unwired: 1 in, 1 out]
            n800 = property on="Channel Controls" class="TabCtl (strict)"("Val(Sgnl)"=w1105) -> ()  [unwired: 2 in, 2 out]
          }
        }
      }
      event "Erase All": Value Change {
        # "Clear data array.\nReset PID."
        n801 = event-data() -> ()  [unwired: 1 in, 6 out]
        n802 = local read "Channel Controls"() -> (w1111:T3)
        n803 = local read "Data"() -> (w1112:cluster{"R":dbl[], "T":dbl[], "Time":dbl[]}[])
        n804 = Replace Array Subset(array=w1112, new element=cluster{"R":dbl[], "T":dbl[], "Time":dbl[]} {"R"=[], "T"=[], "Time"=[]} ("new element/subarray"), index=w1111) -> (w1110:cluster{"R":dbl[], "T":dbl[], "Time":dbl[]}[])
        n805 = local write "Data"(w1110) -> ()
        n806 = disable-structure shown="Disabled" {
          frame Disabled {
            n807 = Initialize Array(cluster{"R":dbl[], "T":dbl[], "Time":dbl[]} {"R"=[], "T"=[], "Time"=[]}, 10 ("dimension size")) -> ()  [unwired: 1 out]
          }
          frame Enabled {
          }
        }
      }
      event "Clear all plots": Value Change {
        n808 = event-data() -> ()  [unwired: 1 in, 6 out]
        n809 = Initialize Array(cluster{"R":dbl[], "T":dbl[], "Time":dbl[]} {"R"=[], "T"=[], "Time"=[]}, 10 ("dimension size")) -> (w1116:cluster{"R":dbl[], "T":dbl[], "Time":dbl[]}[])
        n810 = local write "Data"(w1116) -> ()
      }
      event "Bridge settings.AVS type": Value Change {
        # "Select bridge type (AVS/zBridge). Show/hide corresponding controls."
        n811 = event-data() -> ("NewVal"=w1119:T35)  [unwired: 1 in, 5 out]
        n812 = flat-sequence {
          tunnel: w1119 -> [w1125]
          frame #0 {
            w1121 = u8 0 ("Disabled")
            w1124 = u8 0 ("Disabled")
            w1123 = FALSE ("Visible")
            w1122 = u8 2 ("Disabled")
            n813 = property on="AVS_SPort" class="VISAName"("Visible"=w1123, "Disabled"=w1122) -> ()  [unwired: 2 in, 2 out]
            n814 = property on="Save Screen Data 2" class="Bool"("Visible"=w1123, "Disabled"=w1122) -> ()  [unwired: 2 in, 2 out]
            n815 = property on="Tab Control 5" class="TabCtl (strict)"("Disabled"=w1121) -> ()  [unwired: 2 in, 2 out]
            n816 = property on="Address" class="VISAName"("Visible"=w1123, "Disabled"=w1122) -> ()  [unwired: 2 in, 2 out]
            n817 = property on="Tab Control" class="TabCtl (strict)"("Disabled"=w1121) -> ()  [unwired: 2 in, 2 out]
            n818 = property on="Read AVS channels from" class="DigNum (strict)"("Disabled"=w1124) -> ()  [unwired: 2 in, 2 out]
            n819 = property on="Last Channel" class="DigNum (strict)"("Disabled"=w1124) -> ()  [unwired: 2 in, 2 out]
            n820 = property on="Stabilisation Delay" class="DigNum (strict)"("Disabled"=w1124) -> ()  [unwired: 2 in, 2 out]
            n821 = property on="Averages" class="DigNum (strict)"("Disabled"=w1124) -> ()  [unwired: 2 in, 2 out]
            n822 = property on="Delay Between Scans" class="DigNum (strict)"("Disabled"=w1124) -> ()  [unwired: 2 in, 2 out]
          }
          frame #1 {
            n823 = case shown="\"Disabled\", Default" w1125 {
              frame "AVS47A (GPIB interface)" {
                n824 = local write "Scan Parameters"(enum32{"Page 1", "Page 2"}."Page 1" ("Scan Parameters")) -> ()
                n825 = property on="Address" class="VISAName"("Visible"=TRUE, "Disabled"=u8 0) -> ()  [unwired: 2 in, 2 out]
              }
              frame "AVS47B (RS232 interface)" {
                w1129 = u8 2 ("Disabled")
                n826 = local write "Scan Parameters"(enum32{"Page 1", "Page 2"}."Page 1" ("Scan Parameters")) -> ()
                n827 = property on="AVS_SPort" class="VISAName"("Visible"=TRUE, "Disabled"=u8 0) -> ()  [unwired: 2 in, 2 out]
                n828 = property on="Read AVS channels from" class="DigNum (strict)"("Disabled"=w1129) -> ()  [unwired: 2 in, 2 out]
                n829 = property on="Last Channel" class="DigNum (strict)"("Disabled"=w1129) -> ()  [unwired: 2 in, 2 out]
              }
              frame "AVS48" {
                w1133 = u8 2 ("Disabled")
                n830 = local write "Scan Parameters"(enum32{"Page 1", "Page 2"}."Page 1" ("Scan Parameters")) -> ()
                n831 = property on="AVS_SPort" class="VISAName"("Visible"=TRUE, "Disabled"=u8 0) -> ()  [unwired: 2 in, 2 out]
                n832 = property on="Read AVS channels from" class="DigNum (strict)"("Disabled"=w1133) -> ()  [unwired: 2 in, 2 out]
                n833 = property on="Last Channel" class="DigNum (strict)"("Disabled"=w1133) -> ()  [unwired: 2 in, 2 out]
              }
              frame "AVS Emulation" {
                n834 = local write "Scan Parameters"(enum32{"Page 1", "Page 2"}."Page 1" ("Scan Parameters")) -> ()
              }
              frame "Impedance Bridge" {
                w1140 = u8 2 ("Disabled")
                n835 = local write "Scan Parameters"(enum32{"Page 1", "Page 2"}."Page 2" ("Scan Parameters")) -> ()
                n836 = property on="Save Screen Data 2" class="Bool"("Visible"=TRUE, "Disabled"=u8 0) -> ()  [unwired: 2 in, 2 out]
                n837 = property on="Read AVS channels from" class="DigNum (strict)"("Disabled"=w1140) -> ()  [unwired: 2 in, 2 out]
                n838 = property on="Last Channel" class="DigNum (strict)"("Disabled"=w1140) -> ()  [unwired: 2 in, 2 out]
                n839 = property on="Stabilisation Delay" class="DigNum (strict)"("Disabled"=w1140) -> ()  [unwired: 2 in, 2 out]
                n840 = property on="Averages" class="DigNum (strict)"("Disabled"=w1140) -> ()  [unwired: 2 in, 2 out]
                n841 = property on="Delay Between Scans" class="DigNum (strict)"("Disabled"=w1140) -> ()  [unwired: 2 in, 2 out]
              }
              frame "Disabled", Default {
                w1142 = u8 2 ("Disabled")
                n842 = property on="Tab Control 5" class="TabCtl (strict)"("Disabled"=w1142) -> ()  [unwired: 2 in, 2 out]
                n843 = property on="Tab Control" class="TabCtl (strict)"("Disabled"=w1142) -> ()  [unwired: 2 in, 2 out]
              }
            }
          }
        }
      }
      event "AVS Runtime Settings.Plot type": Value Change {
        # "Iterate through first 10 pages (plots only)"
        # "Switch between RxTime and TxTime plots"
        n844 = event-data() -> ("NewVal"=w1151:enum16{"R vs Time", "T vs Time"})  [unwired: 1 in, 5 out]
        n845 = Equal To 0?(x=w1151) -> (x = 0?=w1150:bool)
        n846 = Select(t=u32 10532351, s=w1150, f=u32 16711680) -> (s? t:f=w1147:u32)
        n847 = property on="uPlots" class="Clust (strict)"() -> ("Controls[]"=w1145:refnum<vi>[])  [unwired: 2 in, 2 out]
        n848 = property on="Channel Controls" class="TabCtl (strict)"() -> ("Pages"=w1152:refnum<vi>[])  [unwired: 2 in, 2 out]
        n849 = for {
          N: 10 -> [_]
          tunnel: w1152 -> [w1162] mode=indexing
          tunnel: w1147 -> [w1155]
          tunnel: w1145 -> [w1153] mode=indexing
          # "!!NOTE:This routine assumes that graph is control #0 on page!!"
          n850 = property class="Page"(reference=w1162) -> ("ControlsOnPage"=w1160:refnum<vi>[])  [unwired: 1 in, 2 out]
          n851 = Type Cast(type=refnum<vi> refnum ("R-Plot 0"), x=w1153) -> (*(type *) &x=w1154:refnum<vi>)
          n852 = Index Array(array=w1160, index=0) -> (element=w1158:refnum<vi>)
          n853 = Type Cast(type=refnum<vi> refnum ("R-Plot 0"), x=w1158) -> (*(type *) &x=w1157:refnum<vi>)
          n854 = property class="XYGraph (strict)"(reference=w1154, "Plot.Plot Color"=w1155, "Plot.Fill/Pt. Color"=w1155) -> ()  [unwired: 1 in, 2 out]
          n855 = property class="XYGraph (strict)"(reference=w1157, "Plot.Plot Color"=w1155, "Plot.Fill/Pt. Color"=w1155) -> ()  [unwired: 1 in, 2 out]
        }
        n856 = property on="ResetPIDloop" class="TypRef (strict)"() -> ("Value"=w1144:refnum<user-event>)  [unwired: 2 in, 2 out]
        n857 = Generate User Event(user event=w1144, event data cluster="" ("event data")) -> ()  [unwired: 2 in, 2 out]
      }
      event "AVS Runtime Settings.Read AVS channels from", "AVS Runtime Settings.Last Channel": Value Change {
        # "Change enabled channels for the AVS bridge"
        n858 = event-data() -> ()  [unwired: 1 in, 6 out]
        n859 = local read "UpdateChannelInfo"() -> (w1164:refnum<user-event>)
        n860 = Generate User Event(user event=w1164, event data cluster=bool[] [] ("event data")) -> ()  [unwired: 2 in, 2 out]
      }
      event "AVS Runtime Settings.Filter graphs:": Value Change {
        # "Graph filtering controls"
        n861 = event-data() -> ("NewVal"=w1165:bool)  [unwired: 1 in, 5 out]
        n862 = call "IsDisabled.vi"("Enabled?"=w1165) -> ("Numeric"=w1166:i16)
        n863 = property on="Y_min" class="DigNum (strict)"("Disabled"=w1166) -> ()  [unwired: 2 in, 2 out]
        n864 = property on="Y_max" class="DigNum (strict)"("Disabled"=w1166) -> ()  [unwired: 2 in, 2 out]
      }
      event "Channel Controls": Value Change {
        # "Show hide bottom Tesistance/Temperature panel depending on the current tab page"
        n865 = event-data() -> ("NewVal"=w1167:T3)  [unwired: 1 in, 5 out]
        n866 = case shown="Default" w1167 {
          frame Default {
            n867 = property on="Mode Buttons" class="RadioBtnsControl (strict)"() -> ("Value"=w1168:T13)  [unwired: 2 in, 2 out]
            n868 = property on="Data History" class="TabCtl (strict)"("Value"=enum32{"History", "Settings"}."History" ("Data History")) -> ()  [unwired: 2 in, 2 out]
            n869 = property on="Mode Buttons" class="RadioBtnsControl (strict)"("Val(Sgnl)"=w1168) -> ()  [unwired: 2 in, 2 out]
          }
          frame "All" {
            n870 = property on="Data History" class="TabCtl (strict)"("Value"=enum32{"History", "Settings"}."Settings" ("Data History")) -> ()  [unwired: 2 in, 2 out]
          }
        }
      }
      event "Thermometer": Value Change {
        # "Calibration changed - update calibrations list"
        n871 = event-data() -> ()  [unwired: 1 in, 6 out]
        n872 = property on="Thermometer" class="Clust (strict)"() -> ("Controls[]"=w1173:refnum<vi>[])  [unwired: 2 in, 2 out]
        n873 = Array Size(array=w1173) -> (size(s)=w1174:i32)
        n874 = for {
          N: w1174 -> [_]
          tunnel: w1173 -> [w1178] mode=indexing
          tunnel: [w1175] -> w1172 mode=indexing
          w1177 = refnum<vi> refnum  # Ring
          n875 = Type Cast(type=w1177, x=w1178) -> (*(type *) &x=w1176:refnum<vi>)
          n876 = property class="Ring"(reference=w1176) -> ("RingText.Text"=w1175:string)  [unwired: 1 in, 2 out]
        }
        n877 = Array To Cluster(array=w1172) -> (cluster=→"CurCalibrations":T23)
      }
      event User Event; "Data logging": Value Change {
        # "Log file settings changed. Generate new log file name"
        n878 = event-data() -> ()  [unwired: 1 in, 3 out]
        n879 = local read "Data logging"() -> (w1186:T27)
        n880 = Unbundle By Name(w1186) -> ("Run description"=w1180:string, "Filenames suffix"=w1181:string, "AVS_Path"=w1187:path, "AVS_FName"=w1185:string, "CAL_FName"=w1184:string)
        n881 = local write "LogFileCreationTime"(timestamp(2742897600 s since 1904-01-01)) -> ()
        n882 = call "MGI Make String Filesafe.vi"("String In"=w1180) -> ("Filesafe String Out"=w1179:string)
        n883 = call "GeneratePaths.vi"("Filename Suffix"=w1181, "Run description"=w1179, "AVS_Path"=w1187, "AVS_FName"=w1185, "CAL_Path"=w1187, "CAL_FName"=w1184) -> ("Generated Log path"=w1183:path, "Generated Calib path"=w1182:path)  [unwired: 8 in]
        n884 = local write "Log path"(w1183) -> ()
        n885 = local write "Calib path"(w1182) -> ()
      }
      event "Convert": Mouse Down; "QuickR": Value Change {
        # "Quick convert R->T"
        n886 = event-data() -> ()  [unwired: 1 in, 4 out]
        n887 = property on="Select sensor 1" class="Ring (strict)"() -> ("Strings []"=w1191:string[], "Value"=w1192:u16)  [unwired: 2 in, 2 out]
        n888 = property on="AVS_CalFolder" class="Path"() -> ("Value"=w1189:path)  [unwired: 2 in, 2 out]
        n889 = Index Array(array=w1191, index=w1192) -> (element=w1190:string)
        n890 = call "SelectSensor-txt no ext.vi"("Path"=w1189, "Resistance"="QuickR", "Select sensor"=w1190) -> ("Temperature"=→"T7":dbl)  [unwired: 1 out]
      }
      event "T Sweep.Current": Value Change {
        # "Current/ Setpoint value is changed"
        n891 = event-data() -> ("NewVal"=→"I3_SetPnt":dbl)  [unwired: 1 in, 5 out]
        n892 = property on="ResetPIDloop" class="TypRef (strict)"() -> ("Value"=w1196:refnum<user-event>)  [unwired: 2 in, 2 out]
        n893 = Generate User Event(user event=w1196, event data cluster="" ("event data")) -> ()  [unwired: 2 in, 2 out]
      }
      event "Automode 2": Value Change {
        n894 = event-data() -> ("NewVal"=w1198:bool)  [unwired: 1 in, 5 out]
        n895 = case shown="True" w1198 {
          frame False {
          }
          frame True {
            # "Set timer to zero (01-01-1904) so the first point is set immediately, w/o wainting for time delay."
            # "If automatic mode is enabled- fire TempStabilized event to record current R,T,I values and start sweeping through TCS channels arrays"
            n896 = disable-structure shown="Disabled" {
              frame Disabled {
                n897 = Generate User Event(event data cluster="" ("event data")) -> ()  [unwired: 3 in, 2 out]
                "Time Old" <- 0.0 ("Timer")
              }
              frame Enabled {
              }
            }
          }
        }
      }
      event "CS Mode": Value Change {
        # "Changed Channel1 automatic mode"
        n898 = event-data() -> ()  [unwired: 1 in, 6 out]
        n899 = property on="CS Mode" class="Enum (strict)"() -> ("Value"=w1202:enum16{"Manual", "Automatic"})  [unwired: 2 in, 2 out]
        n900 = case shown="\"Automatic\"" w1202 {
          tunnel: [TRUE ("Automatic mode ON") FALSE ("Automatic mode ON")] -> w1201
          frame "Automatic" {
            w1210 = TRUE
            # "Set automatic mode currents equal to last manual values. Switch on the current sources."
            n901 = local read "I"() -> (w1219:dbl[])
            n902 = property on="ON" class="Bool (strict)"() -> ("Value"=w1214:bool)  [unwired: 2 in, 2 out]
            n903 = property on="ON" class="Bool (strict)"() -> ("Value"=w1213:bool)  [unwired: 2 in, 2 out]
            n904 = property on="ON" class="Bool (strict)"() -> ("Value"=w1212:bool)  [unwired: 2 in, 2 out]
            n905 = property on="ON" class="Bool (strict)"() -> ("Value"=w1211:bool)  [unwired: 2 in, 2 out]
            n906 = property on="FB on 2" class="Enum (strict)"() -> ("Value"=w1205:enum16{"0", "1", "2", "3"})  [unwired: 2 in, 2 out]
            n907 = Multiply(x=1000.0, y=w1219) -> (x*y=w1206:dbl[])
            n908 = Exclusive Or(1:w1214, 2:w1210) -> (0:w1218:bool)
            n909 = Exclusive Or(1:w1213, 2:w1210) -> (0:w1216:bool)
            n910 = Exclusive Or(1:w1212, 2:w1210) -> (0:w1215:bool)
            n911 = Exclusive Or(1:w1211, 2:w1210) -> (0:w1217:bool)
            n912 = Index Array(array=w1206, index=w1205) -> (element=w1204:dbl)
            n913 = local write "I_in"(w1206) -> ()
            n914 = property on="Toggle ON/OFF" class="Bool (strict)"("Value"=w1218) -> ()  [unwired: 2 in, 2 out]
            n915 = property on="Toggle ON/OFF" class="Bool (strict)"("Value"=w1216) -> ()  [unwired: 2 in, 2 out]
            n916 = property on="Toggle ON/OFF" class="Bool (strict)"("Value"=w1215) -> ()  [unwired: 2 in, 2 out]
            n917 = property on="Toggle ON/OFF" class="Bool (strict)"("Value"=w1217) -> ()  [unwired: 2 in, 2 out]
            n918 = property on="I_0" class="DigNum (strict)"("Value"=w1204) -> ()  [unwired: 2 in, 2 out]
            n919 = property on="TempStabilized" class="TypRef (strict)"() -> ("Value"=w1209:refnum<user-event>)  [unwired: 2 in, 2 out]
            n920 = Generate User Event(user event=w1209, event data cluster=FALSE ("event data")) -> ()  [unwired: 2 in, 2 out]
          }
          frame "Manual" {
            # "Set manual mode currents \nequal to last automode \nvalues."
            n921 = local read "I_in"() -> (w1221:dbl[])
            n922 = Index Array(array=w1221) -> (element #1=w1225:dbl, element #2=w1224:dbl, element #3=w1223:dbl, element #4=w1222:dbl)  [unwired: 4 in]
            n923 = property on="I0" class="DigNum (strict)"("Val(Sgnl)"=w1225) -> ()  [unwired: 2 in, 2 out]
            n924 = property on="I1" class="DigNum (strict)"("Val(Sgnl)"=w1224) -> ()  [unwired: 2 in, 2 out]
            n925 = property on="I2" class="DigNum (strict)"("Val(Sgnl)"=w1223) -> ()  [unwired: 2 in, 2 out]
            n926 = property on="I3" class="DigNum (strict)"("Val(Sgnl)"=w1222) -> ()  [unwired: 2 in, 2 out]
          }
        }
        "Automatic mode 1" <- w1201
        "Automatic mode 2" <- w1201
        "Automatic mode 3" <- w1201
        "Automatic mode 0" <- w1201
      }
      event "Next step": Value Change {
        # "Go to next step in CS auto mode."
        n927 = event-data() -> ()  [unwired: 1 in, 6 out]
        n928 = flat-sequence {
          frame #0 {
            n929 = Get Date/Time In Seconds() -> (seconds since 1Jan1904=w1227:timestamp)
            n930 = To Double Precision Float(number=w1227) -> (double precision float=w1228:dbl)
            n931 = local write "Time Old"(w1228) -> ()
          }
          frame #1 {
            n932 = property on="TempStabilized" class="TypRef (strict)"() -> ("Value"=w1230:refnum<user-event>)  [unwired: 2 in, 2 out]
            n933 = Generate User Event(user event=w1230, event data cluster=TRUE ("event data")) -> ()  [unwired: 2 in, 2 out]
          }
        }
      }
      event "Data logging.External VI path": Value Change {
        # "Set path for the external VI to call on TempStabilised event"
        n934 = event-data() -> ("NewVal"=w1232:path)  [unwired: 1 in, 5 out]
        n935 = vi-ref "OnTempStabilizedRef.vi"() -> (w1233:refnum<vi>)
        n936 = Open VI Reference(type specifier VI Refnum (for type only)=w1233, vi path=w1232) -> (vi reference=w1231:refnum<vi>)  [unwired: 4 in, 1 out]
        n937 = local write "vi reference"(w1231) -> ()
      }
      event "Autorange": Value Change {
        # "Disabled"
        n938 = event-data() -> ("NewVal"=w1234:bool)  [unwired: 1 in, 5 out]
        n939 = Boolean To (0,1)(Boolean=w1234) -> (0, 1=w1237:i16)
        n940 = Multiply(x=i16 2, y=w1237) -> (x*y=w1235:i16)
        n941 = property on="Ranges" class="Clust (strict)"("Disabled"=w1235) -> ()  [unwired: 2 in, 2 out]
      }
      event "Current source settings.CS type": Value Change {
        # "Set CS type"
        n942 = event-data() -> ("NewVal"=w1238:T36)  [unwired: 1 in, 5 out]
        n943 = flat-sequence {
          tunnel: w1238 -> [w1265]
          frame #0 {
            w1250 = u8 2 ("Disabled")
            w1245 = u8 0 ("Disabled")
            w1260 = TRUE ("Visible")
            n944 = control-ref of="Current indicators"() -> (w1246:refnum<vi>)
            n945 = control-ref of="I0"() -> (w1257:refnum<vi>)
            n946 = control-ref of="I1"() -> (w1249:refnum<vi>)
            n947 = control-ref of="C_I0"() -> (w1256:refnum<vi>)
            n948 = control-ref of="C_I1"() -> (w1248:refnum<vi>)
            n949 = control-ref of="I2"() -> (w1244:refnum<vi>)
            n950 = control-ref of="I3"() -> (w1243:refnum<vi>)
            n951 = control-ref of="CS Mode"() -> (w1247:refnum<vi>)
            n952 = control-ref of="Map Channel 0 to 2"() -> (w1255:refnum<vi>)
            n953 = property class="TabCtl (strict)"(reference=w1246, "Disabled"=w1245) -> ()  [unwired: 1 in, 2 out]
            n954 = property class="Clust (strict)"(reference=w1257, "Disabled"=w1245) -> ()  [unwired: 1 in, 2 out]
            n955 = property class="Clust (strict)"(reference=w1249, "Disabled"=w1245) -> ()  [unwired: 1 in, 2 out]
            n956 = property class="Clust (strict)"(reference=w1244, "Disabled"=w1245) -> ()  [unwired: 1 in, 2 out]
            n957 = property class="Clust (strict)"(reference=w1243, "Disabled"=w1245) -> ()  [unwired: 1 in, 2 out]
            n958 = property class="Clust (strict)"(reference=w1256, "Disabled"=w1245) -> ()  [unwired: 1 in, 2 out]
            n959 = property class="Clust (strict)"(reference=w1248, "Disabled"=w1245) -> ()  [unwired: 1 in, 2 out]
            n960 = property class="Enum (strict)"(reference=w1255, "Disabled"=w1245) -> ()  [unwired: 1 in, 2 out]
            n961 = property class="Enum (strict)"(reference=w1247, "Disabled"=w1245) -> ()  [unwired: 1 in, 2 out]
            n962 = control-ref of="TCS_Port"() -> (w1259:refnum<vi>)
            n963 = property on="Tab Control 2" class="TabCtl (strict)"() -> ("Pages"=w1239:refnum<vi>[])  [unwired: 2 in, 2 out]
            n964 = Index Array(array=w1239, index=1) -> (element=w1240:refnum<vi>)
            n965 = control-ref of="Toggle Gated"() -> (w1251:refnum<vi>)
            n966 = control-ref of="Toggle Gated"() -> (w1252:refnum<vi>)
            n967 = control-ref of="Toggle Gated"() -> (w1253:refnum<vi>)
            n968 = control-ref of="Toggle Gated"() -> (w1254:refnum<vi>)
            n969 = control-ref of="QCS/PCS Device"() -> (w1262:refnum<vi>)
            n970 = control-ref of="I0 output to"() -> (w1261:refnum<vi>)
            n971 = property class="Page"(reference=w1240, "PageVis"=TRUE ("Page Visible")) -> ()  [unwired: 1 in, 2 out]
            n972 = property class="Bool (strict)"(reference=w1251, "Disabled"=w1250) -> ()  [unwired: 1 in, 2 out]
            n973 = property class="Bool (strict)"(reference=w1252, "Disabled"=w1250) -> ()  [unwired: 1 in, 2 out]
            n974 = property class="Bool (strict)"(reference=w1253, "Disabled"=w1250) -> ()  [unwired: 1 in, 2 out]
            n975 = property class="Bool (strict)"(reference=w1254, "Disabled"=w1250) -> ()  [unwired: 1 in, 2 out]
            n976 = property class="DigNum (strict)"(reference=w1262, "Visible"=w1260) -> ()  [unwired: 1 in, 2 out]
            n977 = property class="Enum (strict)"(reference=w1261, "Visible"=w1260) -> ()  [unwired: 1 in, 2 out]
            n978 = property class="VISAName"(reference=w1259, "Visible"=FALSE) -> ()  [unwired: 1 in, 2 out]
          }
          frame #1 {
            n979 = case shown="\"QCS v1\"" w1265 {
              tunnel: [refnum<class "TCS.lvclass"> refnum ("TCS.lvclass") refnum<class "QCS.lvclass"> refnum ("QCS.lvclass") w1285 w1299 refnum<class "PCS.lvclass"> refnum ("PCS.lvclass")] -> w1264
              tunnel: [w1266 w1284 u16 255 ("Value") u16 255 ("Value") w1304] -> w1263
              frame "TCS" {
                w1269 = u8 2 ("Disabled")
                w1282 = u8 0 ("Disabled")
                n980 = control-ref of="TCS_Port"() -> (w1272:refnum<vi>)
                n981 = control-ref of="Toggle Gated"() -> (w1281:refnum<vi>)
                n982 = control-ref of="Toggle Gated"() -> (w1280:refnum<vi>)
                n983 = control-ref of="Toggle Gated"() -> (w1279:refnum<vi>)
                n984 = control-ref of="Toggle Gated"() -> (w1278:refnum<vi>)
                n985 = control-ref of="QCS/PCS Device"() -> (w1274:refnum<vi>)
                n986 = control-ref of="I0"() -> (w1277:refnum<vi>)
                n987 = control-ref of="C_I0"() -> (w1270:refnum<vi>)
                n988 = control-ref of="Map Channel 0 to 2"() -> (w1271:refnum<vi>)
                n989 = property class="Bool (strict)"(reference=w1281, "Disabled"=w1282) -> ()  [unwired: 1 in, 2 out]
                n990 = property class="Bool (strict)"(reference=w1280, "Disabled"=w1282) -> ()  [unwired: 1 in, 2 out]
                n991 = property class="Bool (strict)"(reference=w1279, "Disabled"=w1282) -> ()  [unwired: 1 in, 2 out]
                n992 = property class="Bool (strict)"(reference=w1278, "Disabled"=w1282) -> ()  [unwired: 1 in, 2 out]
                n993 = property class="Clust (strict)"(reference=w1270, "Disabled"=w1269) -> ()  [unwired: 1 in, 2 out]
                n994 = property class="Clust (strict)"(reference=w1277, "Disabled"=u8 2) -> ()  [unwired: 1 in, 2 out]
                n995 = property class="DigNum (strict)"(reference=w1274, "Visible"=FALSE) -> ()  [unwired: 1 in, 2 out]
                n996 = property class="VISAName"(reference=w1272, "Visible"=TRUE) -> ()  [unwired: 1 in, 2 out]
                n997 = property class="Enum (strict)"(reference=w1271, "Disabled"=w1269) -> ()  [unwired: 1 in, 2 out]
                n998 = property on="TCS_Port" class="VISAName"() -> ("Value"=w1267:refnum<visa-resource-name>)  [unwired: 2 in, 2 out]
                n999 = call "VISA to RS232 Port Nr.vi"("VISA Resource Name"=w1267) -> ("Port Number"=w1266:u8)  [unwired: 1 in]
              }
              frame "QCS v1" {
                n1000 = property on="QCS/PCS Device" class="DigNum (strict)"() -> ("Value"=w1284:u16)  [unwired: 2 in, 2 out]
              }
              frame "CS Emulation" {
                w1285 = refnum<class "CS Emulation.lvclass"> refnum  # CS Emulation.lvclass
                n1001 = control-ref of="QCS/PCS Device"() -> (w1288:refnum<vi>)
                n1002 = property class="DigNum (strict)"(reference=w1288, "Visible"=FALSE) -> ()  [unwired: 1 in, 2 out]
              }
              frame "Disabled", Default {
                w1289 = u8 2 ("Disabled")
                w1299 = refnum<class "CS Emulation.lvclass"> refnum  # CS Emulation.lvclass
                n1003 = control-ref of="Current indicators"() -> (w1298:refnum<vi>)
                n1004 = control-ref of="I0"() -> (w1293:refnum<vi>)
                n1005 = control-ref of="I1"() -> (w1292:refnum<vi>)
                n1006 = control-ref of="I2"() -> (w1291:refnum<vi>)
                n1007 = control-ref of="I3"() -> (w1290:refnum<vi>)
                n1008 = control-ref of="QCS/PCS Device"() -> (w1302:refnum<vi>)
                n1009 = property class="DigNum (strict)"(reference=w1302, "Visible"=FALSE) -> ()  [unwired: 1 in, 2 out]
                n1010 = property class="Clust (strict)"(reference=w1293, "Disabled"=w1289) -> ()  [unwired: 1 in, 2 out]
                n1011 = property class="Clust (strict)"(reference=w1292, "Disabled"=w1289) -> ()  [unwired: 1 in, 2 out]
                n1012 = property class="Clust (strict)"(reference=w1291, "Disabled"=w1289) -> ()  [unwired: 1 in, 2 out]
                n1013 = property class="Clust (strict)"(reference=w1290, "Disabled"=w1289) -> ()  [unwired: 1 in, 2 out]
                n1014 = property class="TabCtl (strict)"(reference=w1298, "Disabled"=w1289) -> ()  [unwired: 1 in, 2 out]
                n1015 = property on="Tab Control 2" class="TabCtl (strict)"() -> ("Pages"=w1297:refnum<vi>[])  [unwired: 2 in, 2 out]
                n1016 = Index Array(array=w1297, index=1) -> (element=w1296:refnum<vi>)
                n1017 = property class="Page"(reference=w1296, "PageVis"=FALSE ("Page Visible")) -> ()  [unwired: 1 in, 2 out]
              }
              frame "PCS (n.a.)" {
                w1305 = u8 2 ("Disabled")
                n1018 = control-ref of="I0"() -> (w1311:refnum<vi>)
                n1019 = control-ref of="I1"() -> (w1310:refnum<vi>)
                n1020 = control-ref of="C_I0"() -> (w1309:refnum<vi>)
                n1021 = control-ref of="C_I1"() -> (w1308:refnum<vi>)
                n1022 = control-ref of="CS Mode"() -> (w1307:refnum<vi>)
                n1023 = control-ref of="Map Channel 0 to 2"() -> (w1306:refnum<vi>)
                n1024 = property class="Clust (strict)"(reference=w1309, "Disabled"=w1305) -> ()  [unwired: 1 in, 2 out]
                n1025 = property class="Clust (strict)"(reference=w1308, "Disabled"=w1305) -> ()  [unwired: 1 in, 2 out]
                n1026 = property class="Clust (strict)"(reference=w1311, "Disabled"=w1305) -> ()  [unwired: 1 in, 2 out]
                n1027 = property class="Clust (strict)"(reference=w1310, "Disabled"=w1305) -> ()  [unwired: 1 in, 2 out]
                n1028 = property class="Enum (strict)"(reference=w1307, "Disabled"=w1305) -> ()  [unwired: 1 in, 2 out]
                n1029 = property class="Enum (strict)"(reference=w1306, "Disabled"=w1305) -> ()  [unwired: 1 in, 2 out]
                n1030 = property on="QCS/PCS Device" class="DigNum (strict)"() -> ("Value"=w1304:u16)  [unwired: 2 in, 2 out]
              }
            }
            "CS ref" <- w1264
            n1031 = property on="HW Address" class="DigNum (strict)"("Value"=w1263) -> ()  [unwired: 2 in, 2 out]
          }
        }
      }
      event "Current source settings.QCS/PCS Device": Value Change {
        # "Set CS port"
        n1032 = event-data() -> ("NewVal"=w1312:u16)  [unwired: 1 in, 5 out]
        n1033 = property on="CS type" class="Enum (strict)"() -> ("Value"=w1313:T36)  [unwired: 2 in, 2 out]
        n1034 = case shown="\"QCS v1\"" w1313 {
          tunnel: w1312 -> [_ w1316 _]
          frame Default {
          }
          frame "QCS v1" {
            n1035 = Variant To Data(type=u32 255 ("HW Address"), Variant=w1316) -> (data=w1314:u32)  [unwired: 1 in, 1 out]
            n1036 = property on="HW Address" class="DigNum (strict)"("Value"=w1314) -> ()  [unwired: 2 in, 2 out]
          }
          frame "CS Emulation" {
            n1037 = property on="HW Address" class="DigNum (strict)"("Value"=u32 255 ("HW Address")) -> ()  [unwired: 2 in, 2 out]
          }
        }
      }
      event "Current source settings.TCS_Port": Value Change {
        # "Set TCS port"
        n1038 = event-data() -> ("NewVal"=w1318:refnum<visa-resource-name>)  [unwired: 1 in, 5 out]
        n1039 = property on="CS type" class="Enum (strict)"() -> ("Value"=w1319:T36)  [unwired: 2 in, 2 out]
        n1040 = case shown="\"TCS\"" w1319 {
          tunnel: w1318 -> [w1322 _]
          frame "TCS" {
            n1041 = Type Cast(type=refnum<visa-resource-name> refnum ("Value"), x=w1322) -> (*(type *) &x=w1321:refnum<visa-resource-name>)
            n1042 = call "VISA to RS232 Port Nr.vi"("VISA Resource Name"=w1321) -> ("Port Number"=w1323:u8)  [unwired: 1 in]
            n1043 = property on="HW Address" class="DigNum (strict)"("Value"=w1323) -> ()  [unwired: 2 in, 2 out]
          }
          frame Default {
          }
        }
      }
      event "I3 as temp.I3 as temp 2": Value Change {
        # "Enable/disable the PID loop"
        n1044 = event-data() -> ("NewVal"=w1335:bool)  [unwired: 1 in, 5 out]
        n1045 = call "IsDisabled.vi"("Enabled?"=w1335) -> ("Numeric"=w1339:i16)
        n1046 = property on="ResetPIDloop" class="TypRef (strict)"() -> ("Value"=w1338:refnum<user-event>)  [unwired: 2 in, 2 out]
        n1047 = property on="PID setup 2" class="Clust (strict)"("Disabled"=w1339) -> ()  [unwired: 2 in, 2 out]
        n1048 = Generate User Event(user event=w1338, event data cluster="" ("event data")) -> ()  [unwired: 2 in, 2 out]
        n1049 = property on="FB on" class="Enum (strict)"() -> ("Value"=w1332:enum16{"Resistance", "Temperature"})  [unwired: 2 in, 2 out]
        n1050 = property on="FB on 2" class="Enum (strict)"() -> ("Value"=w1331:enum16{"0", "1", "2", "3"})  [unwired: 2 in, 2 out]
        n1051 = property on="I3 as temp 2" class="Bool (strict)"() -> ("Value"=w1325:bool)  [unwired: 2 in, 2 out]
        n1052 = Initialize Array(FALSE, 4 ("dimension size")) -> (w1327:bool[])
        n1053 = And(x=TRUE ("new element/subarray"), y=w1325) -> (x .and. y?=w1324:bool)
        n1054 = Index Array(array=string[] ["%#_g uA", "%#_g mK"], index=w1332) -> (element=w1334:string)
        n1055 = Replace Array Subset(array=w1327, new element=w1324, index=w1331) -> (w1330:bool[])
        n1056 = local write "T Channel"(w1330) -> ()
        n1057 = Select(t=w1334, s=w1335, f="%#_g uA") -> ()  [unwired: 1 out]
      }
      event "Load Data": Value Change {
        # "Load data from log files"
        n1058 = event-data() -> ()  [unwired: 1 in, 6 out]
        n1059 = property on="AVS_Path" class="Path"() -> ("Value"=w1342:path)  [unwired: 2 in, 2 out]
        n1060 = call "File Dialog4"("start path"=w1342) -> ("selected paths"=w1341:path[], "cancelled"=w1340:bool)  [unwired: 11 in, 2 out]
        n1061 = case shown="False" w1340 {
          tunnel: w1341 -> [w1356 _]
          frame False {
            n1062 = property on="AVS type" class="Enum (strict)"() -> ("Value"=w1346:T35)  [unwired: 2 in, 2 out]
            n1063 = for {
              tunnel: w1356 -> [w1383] mode=indexing
              shift-right: [w1381] -> w1353
              shift-left: string[][] [] ("all rows") -> [w1382]
              # "skip header (7 lines)"
              n1064 = call <vilib>:"Read From Spreadsheet File (string).vi"("file path (dialog if empty)"=w1383) -> ("all rows"=w1379:string[][])  [unwired: 6 in, 4 out]
              n1065 = Array Subset(array=w1379, index (row)=7 ("index")) -> (w1378:string[][])  [unwired: 3 in]
              n1066 = Insert Into Array(array=w1382, new element=w1378) -> (w1381:string[][])  [unwired: 2 in]
            }
            n1067 = case shown="Default" w1346 {
              tunnel: [2 ("index") 2 ("index")] -> w1345
              tunnel: [8 ("length") 10 ("length")] -> w1343
              tunnel: [10 ("index") 12 ("index")] -> w1344
              frame Default {
              }
              frame "Impedance Bridge" {
              }
            }
            n1068 = Index Array(array=w1353, index (col)=1 ("disabled index (col)")) -> (element=w1350:string[])  [unwired: 1 in]
            n1069 = Array Subset(array=w1353, index (col)=w1345, length (col)=w1343) -> (w1352:string[][])  [unwired: 2 in]
            n1070 = Array Subset(array=w1353, index (col)=w1344, length (col)=w1343) -> (w1351:string[][])  [unwired: 2 in]
            n1071 = Transpose 2D Array(2D array=w1352) -> (transposed array=w1348:string[][])
            n1072 = Transpose 2D Array(2D array=w1351) -> (transposed array=w1347:string[][])
            n1073 = for {
              tunnel: w1348 -> [w1375] mode=indexing
              tunnel: w1347 -> [w1374] mode=indexing
              tunnel: w1350 -> [w1376]
              tunnel: [w1373] -> w1349 mode=indexing
              # "Sort data by date and remove duplicate points"
              n1074 = Fract/Exp String To Number(string=w1375) -> (number=w1370:dbl[])  [unwired: 3 in, 1 out]
              n1075 = Fract/Exp String To Number(string=w1376) -> (number=w1372:dbl[])  [unwired: 3 in, 1 out]
              n1076 = Fract/Exp String To Number(string=w1374) -> (number=w1371:dbl[])  [unwired: 3 in, 1 out]
              n1077 = call "Sort 1D Array (DBL)__ogtk.vi"("Array in"=w1372) -> ("Sorted Pointers"=w1377:i32[], "Sorted Array out"=w1365:dbl[])  [unwired: 9 in]
              n1078 = call "Reorder 1D Array2 (DBL)__ogtk.vi"("indices"=w1377, "array"=w1370) -> ("reordered array"=w1369:dbl[])  [unwired: 9 in]
              n1079 = call "Reorder 1D Array2 (DBL)__ogtk.vi"("indices"=w1377, "array"=w1371) -> ("reordered array"=w1367:dbl[])  [unwired: 9 in]
              n1080 = call "Remove Duplicates from 1D Array (DBL)__ogtk.vi"("Input Array"=w1369) -> ("Output Array"=w1368:dbl[], "indices of removed elements"=w1363:i32[])
              n1081 = call "Delete Elements from 1D Array (DBL)__ogtk.vi"("indices"=w1363, "array"=w1367) -> ("array w/ subset deleted"=w1366:dbl[])  [unwired: 8 in, 1 out]
              n1082 = call "Delete Elements from 1D Array (DBL)__ogtk.vi"("indices"=w1363, "array"=w1365) -> ("array w/ subset deleted"=w1364:dbl[])  [unwired: 8 in, 1 out]
              n1083 = Bundle("Output Array"=w1368, "array w/ subset deleted"=w1366, "array w/ subset deleted"=w1364) -> (w1373:T50)  [unwired: 1 in]
            }
            n1084 = local write "Data"(w1349) -> ()
          }
          frame True {
          }
        }
      }
      event "Save Data": Value Change {
        # "Load data from log files"
        n1085 = event-data() -> ()  [unwired: 1 in, 6 out]
        n1086 = property on="AVS_Path" class="Path"() -> ("Value"=w1386:path)  [unwired: 2 in, 2 out]
        n1087 = call "File Dialog"("start path"=w1386) -> ("selected path"=w1384:path, "cancelled"=w1385:bool)  [unwired: 11 in, 2 out]
        n1088 = case shown="False" w1385 {
          tunnel: w1384 -> [w1391 _]
          frame False {
            (unwired) 30 ("dimension size")
            n1089 = local read "Data"() -> (w1392:cluster{"R":dbl[], "T":dbl[], "Time":dbl[]}[])
            n1090 = for {
              tunnel: w1392 -> [w1406] mode=indexing
              tunnel: [w1397] -> w1390 mode=indexing
              shift-right: [w1393] -> w1388
              shift-left: string[][] [] -> [w1394]
              n1091 = Unbundle By Name(w1406) -> ("Time"=w1403:dbl[], "R"=w1402:dbl[], "T"=w1398:dbl[])
              n1092 = property on="Data logging" class="Clust (strict)"() -> ("Value"=w1405:T27)  [unwired: 2 in, 2 out]
              n1093 = Unbundle By Name(w1405) -> ("Date/Time Format"=w1404:string)
              n1094 = Array Size(array=w1398) -> (size(s)=w1397:i32)
              n1095 = for {
                tunnel: w1404 -> [w1409]
                tunnel: [w1408] -> w1401 mode=indexing
                tunnel: w1403 -> [w1407] mode=indexing
                n1096 = Format Date/Time String(time format string (%c)=w1409, seconds (now)=w1407) -> (date/time string=w1408:string)  [unwired: 1 in]
              }
              n1097 = Number To Fractional String(number=w1402) -> (F-format string=w1400:string[])  [unwired: 3 in]
              n1098 = Number To Fractional String(number=w1398) -> (F-format string=w1399:string[])  [unwired: 3 in]
              n1099 = Build Array(w1401, w1400, w1399) -> (w1395:string[][])
              n1100 = Transpose 2D Array(2D array=w1395) -> (transposed array=w1396:string[][])
              n1101 = Build Array (concatenate)(w1394, w1396) -> (w1393:string[][])
            }
            n1102 = Array Max & Min(array=w1390) -> ()  [unwired: 4 out]
            n1103 = call "Write To Spreadsheet File (string) w Error.vi"("transpose? (no:F)"=FALSE, "2D data"=w1388, "file path (dialog if empty)"=w1391) -> ()  [unwired: 7 in, 2 out]
          }
          frame True {
          }
        }
      }
      event "Save Screen Data": Value Change {
        n1104 = event-data() -> ()  [unwired: 1 in, 6 out]
        n1105 = property on="AVS_Path" class="Path"() -> ("Value"=w1412:path)  [unwired: 2 in, 2 out]
        n1106 = call "File Dialog7"("start path"=w1412) -> ("selected path"=w1410:path, "cancelled"=w1411:bool)  [unwired: 11 in, 2 out]
        n1107 = case shown="False" w1411 {
          tunnel: w1410 -> [w1437 _]
          frame False {
            # "!!NOTE:This routine assumes that XY graph is \ncontrol #0 on tab page!!"
            n1108 = property on="Channel Controls" class="TabCtl (strict)"() -> ("Pages"=w1435:refnum<vi>[], "Value"=w1434:T3)  [unwired: 2 in, 2 out]
            n1109 = Index Array(array=w1435, index=w1434) -> (element=w1433:refnum<vi>)
            n1110 = property class="Page"(reference=w1433) -> ("ControlsOnPage"=w1430:refnum<vi>[])  [unwired: 1 in, 2 out]
            n1111 = control-ref of="R-Plot 0"() -> (w1428:refnum<vi>)
            n1112 = Index Array(array=w1430, index=0) -> (element=w1432:refnum<vi>)
            n1113 = Type Cast(type=w1428, x=w1432) -> (*(type *) &x=w1429:refnum<vi>)
            n1114 = property class="XYGraph (strict)"(reference=w1429) -> ("Value"=w1427:cluster{dbl[], dbl[]}, "XScale.Maximum"=w1426:dbl, "XScale.Minimum"=w1425:dbl)  [unwired: 1 in, 2 out]
            n1115 = Unbundle(w1427) -> (w1424:dbl[], w1423:dbl[])
            n1116 = call "MGI Threshold 1D Array Extended.vi"("Threshold Y"=w1426, "Y Value[]"=w1424) -> ("Extended Fractional Index"=w1414:dbl)  [unwired: 1 in]
            n1117 = call "MGI Threshold 1D Array Extended.vi"("Threshold Y"=w1425, "Y Value[]"=w1424) -> ("Extended Fractional Index"=w1413:dbl)  [unwired: 1 in]
            n1118 = Subtract(x=w1414, y=w1413) -> (x-y=w1436:dbl)
            n1119 = Array Subset(array=w1424, index=w1413, length=w1436) -> (w1418:dbl[])
            n1120 = Array Subset(array=w1423, index=w1413, length=w1436) -> (w1416:dbl[])
            n1121 = property on="Data logging" class="Clust (strict)"() -> ("Value"=w1420:T27)  [unwired: 2 in, 2 out]
            n1122 = Unbundle By Name(w1420) -> ("Date/Time Format"=w1419:string)
            n1123 = Number To Fractional String(number=w1416) -> (F-format string=w1415:string[])  [unwired: 3 in]
            n1124 = for {
              tunnel: w1419 -> [w1440]
              tunnel: [w1439] -> w1417 mode=indexing
              tunnel: w1418 -> [w1438] mode=indexing
              n1125 = Format Date/Time String(time format string (%c)=w1440, seconds (now)=w1438) -> (date/time string=w1439:string)  [unwired: 1 in]
            }
            n1126 = Build Array(w1417, w1415) -> (w1422:string[][])
            n1127 = call <vilib>:"Write To Spreadsheet File (string).vi"("transpose? (no:F)"=TRUE, "2D data"=w1422, "file path (dialog if empty)"=w1437) -> ()  [unwired: 5 in, 1 out]
          }
          frame True {
          }
        }
      }
      event "Currents changed": Value Change {
        # "New values for currents were entered by user/automode-> write new data to CS"
        n1128 = event-data() -> ()  [unwired: 1 in, 6 out]
        n1129 = local read "CS ref"() -> (w1445:refnum<class "CS.lvclass">)
        n1130 = property on="CS status" class="Clust (strict)"() -> ("Value"=w1442:errorcluster)  [unwired: 2 in, 2 out]
        n1131 = call-dynamic "Read.vi"("CS in"=w1445, "error in (no error)"=w1442, "Optional"=TRUE ("Unused")) -> ("CS out"=w1444:refnum<class "CS.lvclass">, "error out"=w1441:errorcluster)  [unwired: 11 in, 4 out]
        n1132 = local write "CS ref"(w1444) -> ()
        n1133 = property on="CS status" class="Clust (strict)"("Value"=w1441) -> ()  [unwired: 2 in, 2 out]
      }
      event "I0 output to": Value Change {
        # "Switch QCS channel 0 to aux output"
        n1134 = event-data() -> ("OldVal"=w1452:T29, "NewVal"=w1447:T29)  [unwired: 1 in, 4 out]
        n1135 = To Long Integer(number=w1447) -> (32bit integer=→"Map Channel 0 to 2":i32)
        n1136 = local read "CS ref"() -> (w1450:refnum<class "CS.lvclass">)
        n1137 = property on="CS status" class="Clust (strict)"() -> ("Value"=w1451:errorcluster)  [unwired: 2 in, 2 out]
        n1138 = call-dynamic "Switch Output Channel.vi"("error in (no error)"=w1451, "New Channel"=w1447, "Old Channel"=w1452, "CS in"=w1450) -> ("error out"=w1448:errorcluster, "CS out"=w1449:refnum<class "CS.lvclass">)  [unwired: 6 in]
        n1139 = local write "CS ref"(w1449) -> ()
        n1140 = property on="CS status" class="Clust (strict)"("Value"=w1448) -> ()  [unwired: 2 in, 2 out]
      }
      event "T Sweep.Start": Value Change {
        # "Setup and Start Current/Temperature sweep for CS channel 3"
        n1141 = event-data() -> ("CtlRef"=w1453:refnum<vi>, "NewVal"=w1454:bool)  [unwired: 1 in, 4 out]
        n1142 = case shown="False" w1454 {
          tunnel: w1453 -> [w1455 w1458]
          frame False {
            n1143 = property class="Bool (strict)"(reference=w1455, "Caption.Text"="Start") -> ()  [unwired: 1 in, 2 out]
          }
          frame True {
            n1144 = property on="Start value" class="DigNum (strict)"() -> ("Value"=w1459:dbl)  [unwired: 2 in, 2 out]
            n1145 = property class="Bool (strict)"(reference=w1458, "Caption.Text"="Stop") -> ()  [unwired: 1 in, 2 out]
            n1146 = property on="Current" class="DigNum (strict)"("Val(Sgnl)"=w1459) -> ()  [unwired: 2 in, 2 out]
          }
        }
      }
      event "T Sweep.I_next": Value Change {
        # "Go to next step in Current/Temperature sweep for CS channel 3"
        n1147 = event-data() -> ()  [unwired: 1 in, 6 out]
        n1148 = property on="I_next" class="Bool (strict)"("Value"=FALSE) -> ()  [unwired: 2 in, 2 out]
        n1149 = Get Date/Time In Seconds() -> (seconds since 1Jan1904=w1467:timestamp)
        n1150 = To Double Precision Float(number=w1467) -> (double precision float=w1468:dbl)
        n1151 = local write "Time Old"(w1468) -> ()
        n1152 = property on="Current" class="DigNum (strict)"() -> ("Value"=w1460:dbl)  [unwired: 2 in, 2 out]
        n1153 = property on="Step" class="DigNum (strict)"() -> ("Value"=w1465:dbl)  [unwired: 2 in, 2 out]
        n1154 = Add(x=w1460, y=w1465) -> (x+y=w1464:dbl)
        n1155 = property on="End value" class="DigNum (strict)"() -> ("Value"=w1463:dbl)  [unwired: 2 in, 2 out]
        n1156 = property on="Start value" class="DigNum (strict)"() -> ("Value"=w1462:dbl)  [unwired: 2 in, 2 out]
        n1157 = In Range and Coerce(upper limit=w1463, x=w1464, lower limit=w1462) -> (coerced(x)=w1461:dbl)  [unwired: 1 out]
        n1158 = property on="Current" class="DigNum (strict)"("Val(Sgnl)"=w1461) -> ()  [unwired: 2 in, 2 out]
      }
      event "T Sweep.I_prev": Value Change {
        # "Go to previous step in Current/Temperature sweep for CS channel 3"
        n1159 = event-data() -> ()  [unwired: 1 in, 6 out]
        n1160 = Get Date/Time In Seconds() -> (seconds since 1Jan1904=w1476:timestamp)
        n1161 = property on="I_prev" class="Bool (strict)"("Value"=FALSE) -> ()  [unwired: 2 in, 2 out]
        n1162 = To Double Precision Float(number=w1476) -> (double precision float=w1477:dbl)
        n1163 = local write "Time Old"(w1477) -> ()
        n1164 = property on="Current" class="DigNum (strict)"() -> ("Value"=w1470:dbl)  [unwired: 2 in, 2 out]
        n1165 = property on="Step" class="DigNum (strict)"() -> ("Value"=w1475:dbl)  [unwired: 2 in, 2 out]
        n1166 = Subtract(x=w1470, y=w1475) -> (x-y=w1474:dbl)
        n1167 = property on="End value" class="DigNum (strict)"() -> ("Value"=w1473:dbl)  [unwired: 2 in, 2 out]
        n1168 = property on="Start value" class="DigNum (strict)"() -> ("Value"=w1472:dbl)  [unwired: 2 in, 2 out]
        n1169 = In Range and Coerce(upper limit=w1473, x=w1474, lower limit=w1472) -> (coerced(x)=w1471:dbl)  [unwired: 1 out]
        n1170 = property on="Current" class="DigNum (strict)"("Val(Sgnl)"=w1471) -> ()  [unwired: 2 in, 2 out]
      }
      event "Reset PID", "PID setup 2.Integral Gain": Value Change {
        # "Reset the PID loop"
        n1171 = event-data() -> ()  [unwired: 1 in, 6 out]
        n1172 = property on="ResetPIDloop" class="TypRef (strict)"() -> ("Value"=w1479:refnum<user-event>)  [unwired: 2 in, 2 out]
        n1173 = Generate User Event(user event=w1479, event data cluster="" ("event data")) -> ()  [unwired: 2 in, 2 out]
      }
      event User Event {
        # "Reset the PID loop"
        n1174 = event-data() -> ()  [unwired: 1 in, 5 out]
        n1175 = local write "Error"(0.0 ("T_error")) -> ()
      }
      event "Minimize", "Minimize 2": Value Change {
        (unwired) 29 ("Splitter Position")
        (unwired) 534 ("Numeric 2")
        # "Shrink/restore the program window"
        # "726"
        # "222"
        # "1243"
        # "816"
        n1176 = event-data() -> ()  [unwired: 1 in, 6 out]
        n1177 = case shown="False" "Minimize" {
          tunnel: "Minimize 2" -> [_ w1508]
          frame True {
            (unwired) T35."Disabled" ("Value")
            n1178 = property on="CS type" class="Enum (strict)"() -> ("Value"=w1493:T36)  [unwired: 2 in, 2 out]
            n1179 = property on="AVS type" class="Enum (strict)"() -> ("Value"=w1488:T35)  [unwired: 2 in, 2 out]
            n1180 = Equal?(x=w1488, y=T35."Disabled" ("Value")) -> (x = y?=w1486:bool)
            n1181 = Equal?(x=w1493, y=T36."Disabled" ("Value")) -> (x = y?=w1492:bool)
            n1182 = property on="Data History" class="TabCtl (strict)"("Value"=enum32{"History", "Settings"}."History" ("Data History")) -> ()  [unwired: 2 in, 2 out]
            n1183 = Exclusive Or(1:w1486, 2:w1492) -> (0:w1485:bool)
            n1184 = property on="Mode Buttons" class="RadioBtnsControl (strict)"("Disabled"=u8 2, "Val(Sgnl)"=T13."No Selection" ("Value (Signaling)")) -> ()  [unwired: 2 in, 2 out]
            n1185 = property class="VI"() -> ("Front Panel.PanelBounds"=w1496:T51)  [unwired: 2 in, 2 out]
            n1186 = Select(t=i16 105 ("y"), s=w1485, f=i16 169 ("y")) -> (s? t:f=w1489:i16)
            n1187 = Unbundle By Name(w1496) -> ("Left"=w1502:i16, "Top"=w1499:i16)
            n1188 = property on="Splitter 3" class="Splitter"("Position"=29 ("Splitter Position")) -> (error out=w1487:errorcluster)  [unwired: 2 in, 1 out]
            n1189 = Add(x=i16 806 ("right"), y=w1502) -> (x+y=w1501:i16)
            n1190 = Add(x=w1499, y=w1489) -> (x+y=w1498:i16)
            n1191 = Bundle By Name(cluster=w1496, "Right"=w1501, "Bottom"=w1498) -> (w1503:T51)
            n1192 = case shown="True" w1486 {
              tunnel: w1487 -> [_ w1506]
              frame False {
              }
              frame True {
                n1193 = property on="Splitter 4" class="Splitter"(error in=w1506, "Position"=32 ("Splitter Position")) -> ()  [unwired: 1 in, 2 out]
              }
            }
            n1194 = property class="VI"("Front Panel.PanelBounds"=w1503) -> ()  [unwired: 2 in, 2 out]
          }
          frame False {
            n1195 = property class="VI"() -> ("Front Panel.PanelBounds"=w1515:T51)  [unwired: 2 in, 2 out]
            n1196 = property on="Channel Controls" class="TabCtl (strict)"() -> ("Value"=w1523:T3)  [unwired: 2 in, 2 out]
            n1197 = Unbundle By Name(w1515) -> ("Left"=w1521:i16, "Top"=w1519:i16)
            n1198 = property on="Channel Controls" class="TabCtl (strict)"("Val(Sgnl)"=w1523) -> ()  [unwired: 2 in, 2 out]
            n1199 = Select(t=i16 806 ("right"), s=w1508, f=i16 1233 ("right")) -> (s? t:f=w1512:i16)
            n1200 = Add(x=w1512, y=w1521) -> (x+y=w1520:i16)
            n1201 = Add(x=w1519, y=i16 704) -> (x+y=w1517:i16)
            n1202 = Bundle By Name(cluster=w1515, "Right"=w1520, "Bottom"=w1517) -> (w1522:T51)
            n1203 = property on="Mode Buttons" class="RadioBtnsControl (strict)"("Disabled"=u8 0) -> ()  [unwired: 2 in, 2 out]
            n1204 = property class="VI"("Front Panel.PanelBounds"=w1522) -> (error out=w1509:errorcluster)  [unwired: 2 in, 1 out]
            n1205 = property on="Splitter 3" class="Splitter"(error in=w1509, "Position"=559 ("Splitter Position")) -> (error out=w1513:errorcluster)  [unwired: 1 in, 1 out]
            n1206 = property on="Splitter 4" class="Splitter"(error in=w1513, "Position"=635 ("Splitter Position")) -> ()  [unwired: 1 in, 2 out]
          }
        }
        n1207 = property on="Splitter 2" class="Splitter"("Position"=805 ("Splitter Position")) -> ()  [unwired: 2 in, 2 out]
      }
      event "Copy to Clipboard": Value Change {
        # "Copy current values to the clipboard"
        n1208 = event-data() -> ()  [unwired: 1 in, 6 out]
        n1209 = property on="Data array" class="Arr (strict)"() -> ("Value"=w1528:dbl[])  [unwired: 2 in, 2 out]
        n1210 = property on="T_array" class="Arr (strict)"() -> ("Value"=w1527:dbl[])  [unwired: 2 in, 2 out]
        n1211 = Build Array(w1528, w1527) -> (w1526:dbl[][])
        n1212 = Transpose 2D Array(2D array=w1526) -> (transposed array=w1525:dbl[][])
        n1213 = Array To Spreadsheet String(delimiter (Tab)="\t", array=w1525, 3:"%.4g" ("format string")) -> (spreadsheet string=w1531:string)
        n1214 = invoke class="App" method="Clipboard.Write"("Param 0"=w1531) -> ()  [unwired: 3 in, 4 out]
      }
      event "Show PID graph?": Value Change {
        # "Display plots with the PID parameters vs time for debugging"
        n1215 = event-data() -> ("NewVal"=w1532:bool)  [unwired: 1 in, 5 out]
        n1216 = property on="Channel Controls" class="TabCtl (strict)"() -> ("Pages"=w1535:refnum<vi>[])  [unwired: 2 in, 2 out]
        n1217 = Reverse 1D Array(array=w1535) -> (reversed array=w1534:refnum<vi>[])
        n1218 = Index Array(array=w1534) -> (element=w1533:refnum<vi>)  [unwired: 1 in]
        n1219 = property class="Page"(reference=w1533, "PageVis"=w1532) -> ()  [unwired: 1 in, 2 out]
      }
      event "I0.uA", "I1.uA", "I2.uA", "I3.uA": Mouse Up {
        # "Show curent edit filed on double clicking the current indicator. Set the field to the actual current value."
        n1220 = event-data() -> ("Mods.Double Click"=w1537:bool, "CtlRef"=w1536:refnum<vi>)  [unwired: 1 in, 5 out]
        n1221 = case shown="True" w1537 {
          tunnel: w1536 -> [_ w1548]
          frame False {
          }
          frame True {
            w1544 = TRUE ("Visible")
            n1222 = property class="Str"(reference=w1548) -> ("Owner"=w1547:refnum<vi>)  [unwired: 1 in, 2 out]
            n1223 = control-ref of="uA 0"() -> (w1554:refnum<vi>)
            n1224 = control-ref of="uA 1"() -> (w1557:refnum<vi>)
            n1225 = control-ref of="uA 2"() -> (w1556:refnum<vi>)
            n1226 = control-ref of="uA 3"() -> (w1555:refnum<vi>)
            n1227 = control-ref of="I0"() -> (w1545:refnum<vi>)
            n1228 = control-ref of="I1"() -> (w1551:refnum<vi>)
            n1229 = control-ref of="I2"() -> (w1550:refnum<vi>)
            n1230 = control-ref of="I3"() -> (w1543:refnum<vi>)
            n1231 = property on="I" class="Arr (strict)"() -> ("Value"=w1542:dbl[])  [unwired: 2 in, 2 out]
            n1232 = Type Cast(type=w1543, x=w1547) -> (*(type *) &x=w1546:refnum<vi>)
            n1233 = Build Array(w1554, w1557, w1556, w1555) -> (w1553:refnum<vi>[])
            n1234 = Build Array(w1545, w1551, w1550, w1543) -> (w1549:refnum<vi>[])
            n1235 = Search 1D Array(1D array=w1549, element=w1546) -> (index of element=w1541:i32)  [unwired: 1 in]
            n1236 = Index Array(array=w1542, index=w1541) -> (element=w1540:dbl)
            n1237 = Index Array(array=w1553, index=w1541) -> (element=w1552:refnum<vi>)
            n1238 = Multiply(x=1000.0, y=w1540) -> (x*y=w1539:dbl)
            n1239 = property on="Property Node" class="DigNum (strict)"(reference=w1552, "Value"=w1539, "Visible"=w1544, "Key Focus"=w1544) -> ()  [unwired: 1 in, 2 out]
          }
        }
      }
      event "I0.current flows", "I1.current flows", "I2.current flows", "I3.current flows": Mouse Up {
        # "Toggle the current channel by double clickin on the \"On\" led in the current indicator."
        n1240 = event-data() -> ("CtlRef"=w1558:refnum<vi>, "Mods.Double Click"=w1559:bool)  [unwired: 1 in, 5 out]
        n1241 = case shown="True" w1559 {
          tunnel: w1558 -> [_ w1568]
          frame False {
          }
          frame True {
            n1242 = control-ref of="current flows"() -> (w1573:refnum<vi>)
            n1243 = control-ref of="current flows"() -> (w1572:refnum<vi>)
            n1244 = control-ref of="current flows"() -> (w1571:refnum<vi>)
            n1245 = control-ref of="current flows"() -> (w1570:refnum<vi>)
            n1246 = control-ref of="Toggle ON/OFF"() -> (w1567:refnum<vi>)
            n1247 = control-ref of="Toggle ON/OFF"() -> (w1565:refnum<vi>)
            n1248 = control-ref of="Toggle ON/OFF"() -> (w1564:refnum<vi>)
            n1249 = control-ref of="Toggle ON/OFF"() -> (w1566:refnum<vi>)
            n1250 = Build Array(w1573, w1572, w1571, w1570) -> (w1569:refnum<vi>[])
            n1251 = Build Array(w1567, w1565, w1564, w1566) -> (w1563:refnum<vi>[])
            n1252 = Search 1D Array(1D array=w1569, element=w1568) -> (index of element=w1562:i32)  [unwired: 1 in]
            n1253 = Index Array(array=w1563, index=w1562) -> (element=w1561:refnum<vi>)
            n1254 = property class="Bool (strict)"(reference=w1561, "Val(Sgnl)"=TRUE ("Value (Signaling)")) -> ()  [unwired: 1 in, 2 out]
          }
        }
      }
      event "uA 0", "uA 1", "uA 2", "uA 3": Value Change {
        w1575 = refnum<vi> refnum  # Numeric
        w1579 = refnum<vi> refnum  # Enum
        # "User has entered the current by double clicking on the current indicators at the bottom. \nSet range to \"Auto\" and interpret the entered value as [uA]"
        # "!!NOTE:This routine assumes that Current and Range are controls #2 & #3 in current control cluster"
        n1255 = event-data() -> ("CtlRef"=w1587:refnum<vi>, "NewVal"=w1574:u32)  [unwired: 1 in, 4 out]
        n1256 = control-ref of="C_I0"() -> (w1596:refnum<vi>)
        n1257 = control-ref of="C_I1"() -> (w1594:refnum<vi>)
        n1258 = control-ref of="C_I2"() -> (w1595:refnum<vi>)
        n1259 = control-ref of="C_I3"() -> (w1597:refnum<vi>)
        n1260 = control-ref of="uA 0"() -> (w1589:refnum<vi>)
        n1261 = control-ref of="uA 1"() -> (w1592:refnum<vi>)
        n1262 = control-ref of="uA 2"() -> (w1591:refnum<vi>)
        n1263 = control-ref of="uA 3"() -> (w1590:refnum<vi>)
        n1264 = Build Array(w1596, w1594, w1595, w1597) -> (w1593:refnum<vi>[])
        n1265 = Build Array(w1589, w1592, w1591, w1590) -> (w1588:refnum<vi>[])
        n1266 = Search 1D Array(1D array=w1588, element=w1587) -> (index of element=w1586:i32)  [unwired: 1 in]
        n1267 = Index Array(array=w1593, index=w1586) -> (element=w1585:refnum<vi>)
        n1268 = property class="Clust (strict)"(reference=w1585) -> ("Controls[]"=w1584:refnum<vi>[])  [unwired: 1 in, 2 out]
        n1269 = Index Array(array=w1584, index #1=3 ("index"), index #2=2 ("index")) -> (element #1=w1581:refnum<vi>, element #2=w1577:refnum<vi>)
        n1270 = Type Cast(type=w1575, x=w1577) -> (*(type *) &x=w1576:refnum<vi>)
        n1271 = Type Cast(type=w1579, x=w1581) -> (*(type *) &x=w1580:refnum<vi>)
        n1272 = property on="Property Node" class="Num"(reference=w1576, "Value"=w1574) -> ()  [unwired: 1 in, 2 out]
        n1273 = property on="Property Node" class="Enum"(reference=w1580, "Value"=T37."Auto") -> ()  [unwired: 1 in, 2 out]
      }
      event "Ranges": Value Change {
        # "If user has changed the exitation, update the AVS bridge settings."
        n1274 = event-data() -> ("NewVal"=w1599:T18)  [unwired: 1 in, 5 out]
        n1275 = property on="Exc&Ranges" class="Clust (strict)"() -> ("Value"=w1598:T9)  [unwired: 2 in, 2 out]
        n1276 = call "Combine Excitation&Range.vi"("Ranges"=w1599, "Exc&Ranges In"=w1598) -> ("Exc&Ranges Out"=w1600:T52)
        n1277 = property on="Exc&Ranges" class="Clust (strict)"("Value"=w1600) -> ()  [unwired: 2 in, 2 out]
      }
      event Panel Close? {
        # "Ask for confirmation is user is trying to close the program"
        n1278 = event-data() -> ()  [unwired: 1 in, 4 out]
        n1279 = Two Button Dialog(message="Are you sure you want to quit the program?") -> (T button?=w1602:bool)  [unwired: 2 in]
        n1280 = Not(x=w1602) -> (.not. x?=w1603:bool)
        n1281 = event-data("Discard?"=w1603) -> ()  [unwired: 1 in, 1 out]
      }
      event "Save config": Mouse Up {
        (unwired) T39."HKEY_CURRENT_USER" ("root key (HKEY_LOCAL_MACHINE) 2")
        # "Save parameters to the configuration file"
        n1282 = event-data() -> ()  [unwired: 1 in, 8 out]
        n1283 = control-ref of="CS Names"() -> (w1614:refnum<vi>)
        n1284 = control-ref of="AVS names"() -> (w1613:refnum<vi>)
        n1285 = control-ref of="CurCalibrations"() -> (w1607:refnum<vi>)
        n1286 = control-ref of="I3 as temp"() -> (w1605:refnum<vi>)
        n1287 = control-ref of="Automode Settings 2"() -> (w1604:refnum<vi>)
        n1288 = control-ref of="Active"() -> (w1606:refnum<vi>)
        n1289 = control-ref of="Bridge settings"() -> (w1620:refnum<vi>)
        n1290 = control-ref of="AVS Runtime Settings"() -> (w1621:refnum<vi>)
        n1291 = control-ref of="Current source settings"() -> (w1619:refnum<vi>)
        n1292 = control-ref of="Thermometer"() -> (w1622:refnum<vi>)
        n1293 = control-ref of="PID setup 2"() -> (w1623:refnum<vi>)
        n1294 = control-ref of="Data logging"() -> (w1618:refnum<vi>)
        n1295 = call "Current VIs Parent Directory__ogtk.vi"() -> ("Parent Directory (+ Relative)"=w1610:path)  [unwired: 5 in]
        n1296 = call "File Dialog3"("start path"=w1610, "pattern (all files)"="*.ini") -> ("selected path"=w1608:path)  [unwired: 10 in, 3 out]
        n1297 = Build Array(w1606, w1620, w1621, w1619, w1618, w1622, w1623, w1614, w1613, w1607, w1605, w1604) -> (w1616:refnum<vi>[])
        n1298 = call "Save Load Settings to File by Ref with path.vi"("Array of Cluster References"=w1616, "subkey"="SOFTWARE\\Leiden Cryogenics\\TC" ("subkey 2"), "Action"=enum8{"Load", "Save"}."Save", "error in (no error)"=w1612, "configuration file path"=w1608) -> ("error out"=w1611:errorcluster)  [unwired: 4 in]
      }
      event "Load config": Mouse Up {
        # "Load parameters from the configuration file"
        n1299 = event-data() -> ()  [unwired: 1 in, 8 out]
        n1300 = flat-sequence {
          tunnel: [w1648] -> w1633
          tunnel: w1629 -> [w1643]
          tunnel: [w1638] -> w1624
          tunnel: w1633 -> [w1664]
          tunnel: [w1664] -> w1632
          tunnel: [w1662] -> w1625
          tunnel: w1624 -> [w1662]
          tunnel: [w1669] -> w1631
          tunnel: w1632 -> [w1668]
          tunnel: [w1666] -> w1626
          tunnel: w1625 -> [w1666]
          tunnel: w1631 -> [w1675]
          tunnel: [w1675] -> w1630
          tunnel: [w1673] -> w1627
          tunnel: w1626 -> [w1673]
          tunnel: w1630 -> [w1678]
          tunnel: [w1677] -> w1628
          tunnel: w1627 -> [w1676]
          frame #0 {
            (unwired) T39."HKEY_CURRENT_USER" ("root key (HKEY_LOCAL_MACHINE) 2")
            n1301 = call "Current VIs Parent Directory__ogtk.vi"() -> ("Parent Directory (+ Relative)"=w1640:path)  [unwired: 5 in]
            n1302 = control-ref of="Active"() -> (w1636:refnum<vi>)
            n1303 = control-ref of="Bridge settings"() -> (w1649:refnum<vi>)
            n1304 = control-ref of="AVS Runtime Settings"() -> (w1645:refnum<vi>)
            n1305 = control-ref of="Current source settings"() -> (w1646:refnum<vi>)
            n1306 = control-ref of="Data logging"() -> (w1647:refnum<vi>)
            n1307 = control-ref of="PID setup 2"() -> (w1644:refnum<vi>)
            n1308 = control-ref of="CS Names"() -> (w1642:refnum<vi>)
            n1309 = control-ref of="AVS names"() -> (w1641:refnum<vi>)
            n1310 = control-ref of="CurCalibrations"() -> (w1637:refnum<vi>)
            n1311 = control-ref of="I3 as temp"() -> (w1635:refnum<vi>)
            n1312 = control-ref of="Automode Settings 2"() -> (w1634:refnum<vi>)
            n1313 = call "File Dialog2"("start path"=w1640, "pattern (all files)"="*.ini") -> ("selected path"=w1638:path)  [unwired: 10 in, 3 out]
            n1314 = Build Array(w1636, w1649, w1645, w1646, w1647, w1644, w1642, w1641, w1637, w1635, w1634) -> (w1651:refnum<vi>[])
            n1315 = call "Save Load Settings to File by Ref with path.vi"("Array of Cluster References"=w1651, "subkey"="SOFTWARE\\Leiden Cryogenics\\TC" ("subkey 2"), "Action"=enum8{"Load", "Save"}."Load", "error in (no error)"=w1643, "configuration file path"=w1638) -> ("error out"=w1653:errorcluster)  [unwired: 4 in]
            n1316 = disable-structure shown="Disabled" {
              disable-tunnel: w1653 -> [w1656 w1661]
              disable-tunnel: [w1654 w1661] -> w1648
              frame Disabled {
                n1317 = property on="AVS type" class="Enum (strict)"(error in=w1656) -> (error out=w1657:errorcluster, "Value"=w1659:T35)  [unwired: 1 in, 1 out]
                n1318 = Equal To 0?(x=w1659) -> (x = 0?=w1660:bool)
                n1319 = property on="Address" class="VISAName"(error in=w1657, "Visible"=w1660) -> (error out=w1658:errorcluster)  [unwired: 1 in, 1 out]
                n1320 = Not(x=w1660) -> (.not. x?=w1655:bool)
                n1321 = property on="AVS_SPort" class="VISAName"(error in=w1658, "Visible"=w1655) -> (error out=w1654:errorcluster)  [unwired: 1 in, 1 out]
              }
              frame Enabled {
              }
            }
          }
          frame #1 {
            n1322 = Wait (ms)(milliseconds to wait=250) -> ()  [unwired: 1 out]
          }
          frame #2 {
            n1323 = control-ref of="Thermometer"() -> (w1667:refnum<vi>)
            n1324 = control-ref of="CurCalibrations"() -> (w1665:refnum<vi>)
            n1325 = control-ref of="AVS_CalFolder"() -> (w1671:refnum<vi>)
            n1326 = control-ref of="Select sensor 1"() -> (w1672:refnum<vi>)
            n1327 = control-ref of="Select sensor 1"() -> (w1670:refnum<vi>)
            n1328 = call "ReloadCalibrations.vi"("error in (no error)"=w1668, "Quick convert sensors"=w1670, "CurCalibrations"=w1665, "Calibration files path"=w1671, "Channel1 sensors"=w1672, "Channels list"=w1667) -> ("error out"=w1669:errorcluster)  [unwired: 1 in]
          }
          frame #3 {
            n1329 = Wait (ms)(milliseconds to wait=250) -> ()  [unwired: 1 out]
          }
          frame #4 {
            n1330 = disable-structure shown="Enabled" {
              disable-tunnel: w1678 -> [w1681 w1689]
              disable-tunnel: [w1680 w1687] -> w1677
              disable-tunnel: w1676 -> [w1679 _]
              frame Enabled {
                (unwired) T39."HKEY_CURRENT_USER" ("root key (HKEY_LOCAL_MACHINE) 2")
                n1331 = control-ref of="Thermometer"() -> (w1684:refnum<vi>)
                n1332 = Build Array(w1684) -> (w1683:refnum<vi>[])
                n1333 = call "Save Load Settings to File by Ref with path.vi"("Array of Cluster References"=w1683, "subkey"="SOFTWARE\\Leiden Cryogenics\\TC" ("subkey 2"), "Action"=enum8{"Load", "Save"}."Load", "error in (no error)"=w1681, "configuration file path"=w1679) -> ("error out"=w1680:errorcluster)  [unwired: 4 in]
              }
              frame Disabled {
                n1334 = property on="UpdateCalibrations" class="TypRef (strict)"(error in=w1689) -> (error out=w1688:errorcluster, "Value"=w1690:refnum<user-event>)  [unwired: 1 in, 1 out]
                n1335 = Generate User Event(user event=w1690, event data cluster="" ("event data"), error in=w1688) -> (error out=w1687:errorcluster)  [unwired: 1 in, 1 out]
              }
            }
          }
        }
      }
      event "Save Screen Data 2": Value Change {
        # "Show parameters menu. (only for zBridge)"
        n1336 = event-data() -> ()  [unwired: 1 in, 6 out]
        n1337 = disable-structure shown="Enabled" {
          frame Enabled {
            w1695 = 0 ("Page")
            n1338 = local read "zConfig"() -> (w1691:path)
            n1339 = local read "zDll"() -> (w1692:path)
            n1340 = call "SetParFilePath.vi"("path"=w1691, "zDll"=w1692) -> ("error out"=w1693:errorcluster, "zDll out"=w1694:path)  [unwired: 8 in]
            n1341 = call "ParamMenu.vi"("error in (no error)"=w1693, "Subpage"=w1695, "Page"=w1695, "path in"=w1694) -> ()  [unwired: 6 in, 2 out]
          }
          frame Disabled {
            n1342 = local read "zConfig"() -> (w1698:path)
            n1343 = local read "zDll"() -> (w1696:path)
            n1344 = call "SetParFilePath.vi"("path"=w1698, "zDll"=w1696) -> ("zDll out"=w1697:path)  [unwired: 8 in, 1 out]
            n1345 = call "zBridgeSettings_1page.vi"("zDll"=w1697) -> ()  [unwired: 10 in, 1 out]
          }
        }
      }
      event "Edit Calibrations": Value Change {
        # "Show calibration files editor. Works with .cal and .cal2 files only"
        n1346 = event-data() -> ("NewVal"=w1707:T6)  [unwired: 1 in, 5 out]
        n1347 = Cluster To Array(cluster=w1707) -> (array=w1706:bool[])
        n1348 = local read "CurCalibrations"() -> (w1701:T23)
        n1349 = Search 1D Array(1D array=w1706, element=TRUE) -> (index of element=w1704:i32)  [unwired: 1 in]
        n1350 = Cluster To Array(cluster=w1701) -> (array=w1700:string[])
        n1351 = Index Array(array=w1700, index=w1704) -> (element=w1703:string)
        n1352 = property on="AVS_CalFolder" class="Path"() -> ("Value"=w1702:path)  [unwired: 2 in, 2 out]
        n1353 = call "Edit Calibration Coefficients.vi"("Calibration Name"=w1703, "Calibration folder"=w1702) -> ("Cancelled?"=w1699:bool)  [unwired: 1 out]
        n1354 = case shown="False" w1699 {
          frame False {
            n1355 = property on="UpdateCalibrations" class="TypRef (strict)"() -> ("Value"=w1709:refnum<user-event>)  [unwired: 2 in, 2 out]
            n1356 = Generate User Event(user event=w1709, event data cluster="" ("event data")) -> ()  [unwired: 2 in, 2 out]
          }
          frame True {
          }
        }
      }
      event "Edit calibration": Value Change {
        # "Show calibration files editor for quick convert R->T. Works with .cal and .cal2 files only"
        n1357 = event-data() -> ()  [unwired: 1 in, 6 out]
        n1358 = property on="Select sensor 1" class="Ring (strict)"() -> ("Strings []"=w1712:string[], "Value"=w1713:u16)  [unwired: 2 in, 2 out]
        n1359 = Index Array(array=w1712, index=w1713) -> (element=w1711:string)
        n1360 = property on="AVS_CalFolder" class="Path"() -> ("Value"=w1714:path)  [unwired: 2 in, 2 out]
        n1361 = call "Edit Calibration Coefficients.vi"("Calibration Name"=w1711, "Calibration folder"=w1714) -> ("Cancelled?"=w1710:bool)  [unwired: 1 out]
        n1362 = case shown="False" w1710 {
          frame False {
            n1363 = property on="UpdateCalibrations" class="TypRef (strict)"() -> ("Value"=w1716:refnum<user-event>)  [unwired: 2 in, 2 out]
            n1364 = Generate User Event(user event=w1716, event data cluster="" ("event data")) -> ()  [unwired: 2 in, 2 out]
          }
          frame True {
          }
        }
      }
      event "zBridge params.AVS Name 0", "zBridge params.AVS Name 1", "zBridge params.AVS Name 2", "zBridge params.AVS Name 3", "zBridge params.AVS Name 4", "zBridge params.AVS Name 5", "zBridge params.AVS Name 6", "zBridge params.AVS Name 7", "zBridge params.AVS Name 8", "zBridge params.AVS Name 9": Mouse Down {
        # "Show parameters menu for the channel by double clicking on \"Channel parameters\". (only for zBridge)"
        n1365 = event-data() -> ("CtlRef"=w1719:refnum<vi>, "Mods.Double Click"=w1718:bool, "PlatMods.Alt"=w1717:bool)  [unwired: 1 in, 5 out]
        n1366 = case shown="False" w1718 {
          tunnel: w1719 -> [w1722 w1727]
          tunnel: w1717 -> [_ w1726]
          frame True {
            n1367 = control-ref of="zBridge params"() -> (w1724:refnum<vi>)
            n1368 = property class="Clust (strict)"(reference=w1724) -> ("Controls[]"=w1723:refnum<vi>[])  [unwired: 1 in, 2 out]
            n1369 = Search 1D Array(1D array=w1723, element=w1722) -> (index of element=w1720:i32)  [unwired: 1 in]
            n1370 = local read "zDll"() -> (w1725:path)
            n1371 = call "ParamMenu.vi"("Subpage"=w1720, "Page"=0, "path in"=w1725) -> ()  [unwired: 7 in, 2 out]
          }
          frame False {
            n1372 = case shown="True" w1726 {
              tunnel: w1727 -> [_ w1730]
              frame False {
              }
              frame True {
                # "Show information window.\nTends to crash the acquisition!"
                n1373 = control-ref of="zBridge params"() -> (w1732:refnum<vi>)
                n1374 = property class="Clust (strict)"(reference=w1732) -> ("Controls[]"=w1731:refnum<vi>[])  [unwired: 1 in, 2 out]
                n1375 = local read "zDll"() -> (w1729:path)
                n1376 = Search 1D Array(1D array=w1731, element=w1730) -> (index of element=w1728:i32)  [unwired: 1 in]
                n1377 = call "Show Info Window.vi"("Data set number"=w1728, "zDll"=w1729) -> ()  [unwired: 8 in, 2 out]
              }
            }
          }
        }
      }
      event "Active.active Channel 0", "Active.active Channel 1", "Active.active Channel 2", "Active.active Channel 3", "Active.active Channel 4", "Active.active Channel 5", "Active.active Channel 6", "Active.active Channel 7", "Active.active Channel 8", "Active.active Channel 9": Mouse Down {
        # "Switch channels On/Off by double clicking on \"Active\" LED. (only for zBridge and AVS47B)"
        n1378 = event-data() -> ("CtlRef"=w1735:refnum<vi>, "Mods.Double Click"=w1733:bool)  [unwired: 1 in, 6 out]
        n1379 = property on="AVS type" class="Enum (strict)"() -> ("Value"=w1734:T35)  [unwired: 2 in, 2 out]
        n1380 = case shown="True" w1733 {
          tunnel: w1735 -> [_ w1737]
          tunnel: w1734 -> [_ w1741]
          frame False {
          }
          frame True {
            n1381 = control-ref of="Active"() -> (w1740:refnum<vi>)
            n1382 = property class="Clust (strict)"(reference=w1740) -> ("Controls[]"=w1738:refnum<vi>[])  [unwired: 1 in, 2 out]
            n1383 = property class="Bool (strict)"(reference=w1737) -> ("Value"=w1736:bool)  [unwired: 1 in, 2 out]
            n1384 = Search 1D Array(1D array=w1738, element=w1737) -> (index of element=w1739:i32)  [unwired: 1 in]
            n1385 = case shown="Default" w1741 {
              tunnel: w1739 -> [_ w1746 w1747]
              tunnel: w1738 -> [_ w1745 _]
              tunnel: w1736 -> [_ w1742 _]
              frame Default {
              }
              frame "AVS47B (RS232 interface)" {
                n1386 = Index Array(array=w1745, index=w1746) -> (element=w1744:refnum<vi>)
                n1387 = Not(x=w1742) -> (.not. x?=w1743:bool)
                n1388 = property class="Ctl"(reference=w1744, "Value"=w1743) -> ()  [unwired: 1 in, 2 out]
              }
              frame "Impedance Bridge" {
                w1749 = T53."Active" ("Enum")
                # "Invert Active flag"
                n1389 = local read "zDll"() -> (w1752:path)
                n1390 = call "GetByteParam.vi"("ParNo"=w1749, "SetNo"=w1747, "zDll"=w1752) -> ("return type"=w1751:u8)  [unwired: 6 in, 2 out]
                n1391 = Decrement(x=w1751) -> (x-1=w1750:i8)
                n1392 = Absolute Value(x=w1750) -> (abs(x)=w1748:i8)
                n1393 = call "SetByteParam.vi"("SetNo"=w1747, "ParNo"=w1749, "Data"=w1748, "zDll"=w1752) -> ()  [unwired: 6 in, 2 out]
              }
            }
          }
        }
      }
      event "Small R.R1 2", "Small R.R1 2", "Small R.R1 2", "Small R.R1 2", "Small R.R1 2", "Small R.R1 2", "Small R.R1 2", "Small R.R1 2", "Small R.R1 2", "Small R.R1 2", "Small T.R1", "Small T.R1", "Small T.R1", "Small T.R1", "Small T.R1", "Small T.R1", "Small T.R1", "Small T.R1", "Small T.R1", "Small T.R1": Mouse Down {
        n1394 = event-data() -> ()  [unwired: 1 in, 8 out]
      }
      event "PID setup 2.FB on 2": Value Change {
        n1395 = event-data() -> ("NewVal"=w1755:enum16{"0", "1", "2", "3"})  [unwired: 1 in, 5 out]
        n1396 = property on="ResetPIDloop" class="TypRef (strict)"() -> ("Value"=w1764:refnum<user-event>)  [unwired: 2 in, 2 out]
        n1397 = Generate User Event(user event=w1764, event data cluster="" ("event data")) -> ()  [unwired: 2 in, 2 out]
        n1398 = property on="I3 as temp 2" class="Bool (strict)"() -> ("Value"=w1757:bool)  [unwired: 2 in, 2 out]
        n1399 = Initialize Array(FALSE, 4 ("dimension size")) -> (w1759:bool[])
        n1400 = And(x=TRUE ("new element/subarray"), y=w1757) -> (x .and. y?=w1756:bool)
        n1401 = Replace Array Subset(array=w1759, new element=w1756, index=w1755) -> (→"T Channel":bool[])
        n1402 = Index Array(array=string[] ["%#_g uA", "%#_g mK"], index=w1755) -> ()  [unwired: 1 out]
      }
      event "AVS names": Value Change {
        # "Update channel names on the small bottom panel when the names are changed."
        n1403 = event-data() -> ("NewVal"=→"AVS names small":T5)  [unwired: 1 in, 5 out]
      }
      event "I_list": Value Change {
        n1404 = event-data() -> ("NewVal"=w1769:dbl[][])  [unwired: 1 in, 5 out]
        n1405 = local read "I_list_idx"() -> (w1768:i32)
        n1406 = Decrement(x=w1768) -> (x-1=w1767:i32)
        n1407 = Array Size(array=w1769) -> (size(s)=w1771:i32[])
        n1408 = Index Array(array=w1771) -> (element=→"I_list_idx_max":i32)  [unwired: 1 in]
        n1409 = Index Array(array=w1769, index (row)=w1767) -> (element=→"I_list[i]":dbl[])  [unwired: 1 in]
      }
      event "I_list": Shortcut Menu Activation? {
        n1410 = event-data() -> ()  [unwired: 1 in, 7 out]
        n1411 = event-data() -> ()  [unwired: 2 in, 1 out]
      }
      event "I_list": Shortcut Menu Selection (App) {
        n1412 = event-data() -> ("ItemTag"=w1772:string)  [unwired: 1 in, 7 out]
        n1413 = case shown="\"APP_SC_COPY_DATA\"" w1772 {
          frame Default {
          }
          frame "APP_SC_PASTE_DATA" {
            n1414 = invoke class="App" method="Clipboard.Read"() -> ("Read Clipbrd"=w1775:string)  [unwired: 3 in, 2 out]
            n1415 = Spreadsheet String To Array(format string="%d", spreadsheet string=w1775) -> (array=w1773:dbl[][])  [unwired: 2 in]
            n1416 = local write "I_list"(w1773) -> ()
          }
          frame "APP_SC_COPY_DATA" {
            n1417 = local read "I_list"() -> (w1778:dbl[][])
            n1418 = Array To Spreadsheet String(array=w1778, 3:"%d" ("format string")) -> (spreadsheet string=w1776:string)  [unwired: 1 in]
            n1419 = invoke class="App" method="Clipboard.Write"("Param 0"=w1776) -> ()  [unwired: 3 in, 4 out]
          }
        }
      }
      event "I_tofirst": Value Change {
        n1420 = event-data() -> ("OldVal"=w1779:bool)  [unwired: 1 in, 5 out]
        n1421 = local write "I_tofirst"(w1779) -> ()
        n1422 = property on="I_list_idx" class="DigNum (strict)"("Val(Sgnl)"=1 ("Value (Signaling)")) -> ()  [unwired: 2 in, 2 out]
      }
      event "I_next": Value Change {
        n1423 = event-data() -> ("OldVal"=w1781:bool)  [unwired: 1 in, 5 out]
        n1424 = local write "I_next"(w1781) -> ()
        n1425 = local read "I_list_idx"() -> (w1783:i32)
        n1426 = Increment(x=w1783) -> (x+1=w1782:i32)
        n1427 = property on="I_list_idx" class="DigNum (strict)"("Val(Sgnl)"=w1782) -> ()  [unwired: 2 in, 2 out]
      }
      event "I_prev": Value Change {
        n1428 = event-data() -> ("OldVal"=w1784:bool)  [unwired: 1 in, 5 out]
        n1429 = local write "I_prev"(w1784) -> ()
        n1430 = local read "I_list_idx"() -> (w1786:i32)
        n1431 = Decrement(x=w1786) -> (x-1=w1785:i32)
        n1432 = property on="I_list_idx" class="DigNum (strict)"("Val(Sgnl)"=w1785) -> ()  [unwired: 2 in, 2 out]
      }
      event "I_Clear": Value Change {
        n1433 = event-data() -> ()  [unwired: 1 in, 6 out]
        n1434 = flat-sequence {
          frame #0 {
            n1435 = local write "I_list"(dbl[][] [] ("I_list")) -> ()
          }
          frame #1 {
            n1436 = property on="I_tofirst" class="Bool (strict)"("Val(Sgnl)"=TRUE ("Value (Signaling)")) -> ()  [unwired: 2 in, 2 out]
          }
        }
      }
      event "I_list_idx": Value Change {
        w1810 = 10  # Lines to scroll
        n1437 = event-data() -> ("NewVal"=w1793:i32)  [unwired: 1 in, 5 out]
        n1438 = Array Size(array="I_list") -> (size(s)=w1796:i32[])
        n1439 = Index Array(array=w1796) -> (element=w1794:i32)  [unwired: 1 in]
        n1440 = Get Date/Time In Seconds() -> (seconds since 1Jan1904=w1790:timestamp)
        n1441 = local write "I_list_idx_max"(w1794) -> ()
        n1442 = To Double Precision Float(number=w1790) -> (double precision float=w1789:dbl)
        n1443 = local write "Time Old"(w1789) -> ()
        n1444 = In Range and Coerce(upper limit=w1794, x=w1793, lower limit=1) -> (coerced(x)=w1791:i32)  [unwired: 1 out]
        "I_list_idx" <- w1791
        n1445 = Decrement(x=w1791) -> (x-1=w1792:i32)
        n1446 = Initialize Array(FALSE, w1810) -> (w1811:bool[])
        n1447 = Index Array(array="I_list", index (row)=w1792) -> (element=w1813:dbl[])  [unwired: 1 in]
        n1448 = local write "I_list[i]"(w1813) -> ()
        n1449 = Subtract(x=w1792, y=w1810) -> (x-y=w1800:i32)
        n1450 = Increment(x=w1800) -> (x+1=w1799:i32)
        n1451 = Decrement(x=w1810) -> (x-1=w1808:i32)
        n1452 = In Range and Coerce(upper limit=inf, x=w1799, lower limit=0) -> (coerced(x)=w1798:dbl)  [unwired: 1 out]
        n1453 = In Range and Coerce(upper limit=w1808, x=w1792, lower limit=0) -> (coerced(x)=w1805:i32)  [unwired: 1 out]
        n1454 = control-ref of="I_list"() -> (w1803:refnum<vi>)
        n1455 = Build Array(w1798, 0 ("element")) -> (w1804:dbl[])
        n1456 = Replace Array Subset(array=w1811, new element=TRUE ("new element/subarray"), index=w1805) -> (→"I_selection":bool[])
        n1457 = property class="Arr (strict)"(reference=w1803, "Index Values"=w1804) -> ()  [unwired: 1 in, 2 out]
      }
      event "Save to file": Value Change {
        n1458 = event-data() -> ()  [unwired: 1 in, 6 out]
        n1459 = call "File Dialog6"() -> ("selected path"=w1816:path, "cancelled"=w1815:bool)  [unwired: 12 in, 2 out]
        n1460 = case shown="False" w1815 {
          tunnel: w1816 -> [w1817 _]
          frame False {
            n1461 = local read "I_list"() -> (w1819:dbl[][])
            n1462 = call <vilib>:"Write To Spreadsheet File (DBL).vi"("format (%.3f)"="%.1f", "2D data"=w1819, "file path (dialog if empty)"=w1817) -> ()  [unwired: 5 in, 1 out]
          }
          frame True {
          }
        }
      }
      event "Load from file": Value Change {
        n1463 = event-data() -> ()  [unwired: 1 in, 6 out]
        n1464 = call "File Dialog5"() -> ("selected path"=w1820:path, "cancelled"=w1821:bool)  [unwired: 12 in, 2 out]
        n1465 = case shown="False" w1821 {
          tunnel: w1820 -> [w1822 _]
          frame False {
            n1466 = call <vilib>:"Read From Spreadsheet File (DBL).vi"("file path (dialog if empty)"=w1822) -> ("all rows"=w1823:dbl[][])  [unwired: 6 in, 4 out]
            n1467 = local write "I_list"(w1823) -> ()
          }
          frame True {
          }
        }
      }
      event "Write to log": Value Change {
        n1468 = event-data() -> ()  [unwired: 1 in, 6 out]
        n1469 = property on="TempStabilized" class="TypRef (strict)"() -> ("Value"=w1825:refnum<user-event>)  [unwired: 2 in, 2 out]
        n1470 = Generate User Event(user event=w1825, event data cluster=FALSE ("event data")) -> ()  [unwired: 2 in, 2 out]
      }
      event "Set Color": Value Change {
        n1471 = event-data() -> ()  [unwired: 1 in, 6 out]
        n1472 = property on="ColorBox" class="TabCtl (strict)"("Visible"=TRUE) -> ()  [unwired: 2 in, 2 out]
      }
      event "ColorBox": Mouse Move {
        n1473 = event-data() -> ("Coords"=w1829:T49)  [unwired: 1 in]
        n1474 = call <vilib>:"Picture to Pixmap.vi"("picture"="Colors") -> ("image data"=w1835:T48)  [unwired: 9 in, 1 out]
        n1475 = property on="Colors" class="Pict"() -> ("Position"=w1828:T54)  [unwired: 2 in, 2 out]
        n1476 = call <vilib>:"Unflatten Pixmap.vi"("image data"=w1835) -> ("24-bit pixmap"=w1830:u32[][])  [unwired: 4 in, 6 out]
        n1477 = Subtract(x=w1829, y=w1828) -> (x-y=w1833:T49)
        n1478 = Unbundle(w1833) -> ("Horizontal"=w1832:i32, "Vertical"=w1831:i32)
        n1479 = Index Array(array=w1830, index (row)=w1831, index (col)=w1832) -> (element=→"Color":u32)
      }
      event "ColorBox": Mouse Down {
        n1480 = event-data() -> ()  [unwired: 1 in, 8 out]
        n1481 = property on="ColorBox" class="TabCtl (strict)"("Visible"=FALSE) -> ()  [unwired: 2 in, 2 out]
      }
    }
    "General" <- w21
  }
  n1482 = while {
    stop <- w1837 stop-if-true
    # "Main loop"
    n1483 = property on="start 2" class="Bool (strict)"() -> ("Value"=w1839:bool)  [unwired: 2 in, 2 out]
    n1484 = Wait (ms)(milliseconds to wait=u32 200) -> ()  [unwired: 1 out]
    n1485 = case shown="True" w1839 {
      frame False {
        n1486 = Wait (ms)(milliseconds to wait=u32 250) -> ()  [unwired: 1 out]
      }
      frame True {
        n1487 = while {
          i -> [w1851]
          stop <- "Stop" stop-if-true
          # "AVS/zBridge read-out"
          n1488 = case shown="False" "Pause" {
            tunnel: w1851 -> [w1858 _]
            frame False {
              # "for the first measurement set Stab.Time=12 s to do autoranging"
              n1489 = property on="AVS Runtime Settings" class="Clust (strict)"() -> ("Value"=w1875:T17)  [unwired: 2 in, 2 out]
              n1490 = Unbundle By Name(w1875) -> ("Stabilisation Delay"=w1866:dbl, "Averages"=w1859:u16, "Last Channel"=w1874:i8, "Read AVS channels from"=w1873:i8)
              n1491 = local read "Active"() -> (w1856:T12)
              n1492 = property on="AVS type" class="Enum (strict)"() -> ("Value"=w1871:T35)  [unwired: 2 in, 2 out]
              n1493 = call "Split Exc&Range.vi"("Excitations 2"="Exc&Ranges") -> ("Excitations"=w1863:T18, "Ranges"=w1857:T55)  [unwired: 4 in]
              n1494 = property on="AVS VISA session" class="VISAName"() -> ("Value"=w1872:refnum<visa-resource-name>)  [unwired: 2 in, 2 out]
              n1495 = Cluster To Array(cluster=w1856) -> (array=w1855:bool[])
              n1496 = call "If First Iteration.vi"("Iteration"=w1858, "Value In"=w1866, "Default"=12.0) -> ("Value Out"=w1865:dbl)
              n1497 = case shown="\"Impedance Bridge\"" w1871 {
                tunnel: w1872 -> [w1885 w1896 _ _ _ _]
                tunnel: w1865 -> [w1881 w1899 w1901 w1911 _ _]
                tunnel: w1859 -> [w1882 w1898 _ _ _ _]
                tunnel: w1874 -> [w1883 w1894 _ _ _ _]
                tunnel: w1873 -> [w1884 w1895 _ _ _ _]
                tunnel: w1863 -> [w1886 w1890 _ _ _ _]
                tunnel: [w1877 w1889 errorcluster {"status"=FALSE, "code"=0, "source"=""} ("error out") errorcluster {"status"=FALSE, "code"=0, "source"=""} ("error out") w1931 errorcluster {"status"=FALSE, "code"=0, "source"=""} ("error out")] -> w1862
                tunnel: w1857 -> [w1879 w1892 w1906 w1912 w1932 w1936]
                tunnel: "Autorange" -> [w1880 w1893 _ _ _ _]
                tunnel: [w1878 w1891 w1906 w1912 w1932 w1936] -> w1854
                tunnel: [w1876 w1888 dbl[] [] ("Data array") w1910 w1923 dbl[] [] ("Data array")] -> w1860
                tunnel: w1855 -> [_ w1887 _ _ _ _]
                frame "AVS47A (GPIB interface)" {
                  # "AVS 47 (GPIB)"
                  n1498 = call "AVS_do_single_scan.vi"("AVS Port"=w1885, "Stabilization Delay"=w1881, "Autorange"=w1880, "Number of Averages"=w1882, "Last Channel"=w1883, "First Channel"=w1884, "Excitations"=w1886, "Ranges"=w1879) -> ("error out"=w1877:errorcluster, "R"=w1876:dbl[], "Ranges"=w1878:T56)  [unwired: 3 in, 2 out]
                }
                frame "AVS47B (RS232 interface)" {
                  # "AVS 47B (RS232)"
                  n1499 = Type Cast(type=refnum<visa-resource-name> refnum ("dup VISA session"), x=w1896) -> (*(type *) &x=w1900:refnum<visa-resource-name>)
                  n1500 = call "Scanner.vi"("STABILIZATION  DELAY"=w1899, "FIRST CH TO SCAN"=w1895, "LAST CH TO SCAN"=w1894, "Autorange"=w1893, "AVERAGE COUNT"=w1898, "Excitation"=w1890, "Range"=w1892, "VISA resource"=w1900, "array"=w1887) -> ("RI"=w1888:dbl[], "Range out"=w1891:T57, "error out 2"=w1889:errorcluster)  [unwired: 1 in, 3 out]
                }
                frame "AVS48" {
                  n1501 = Multiply(x=w1901, y=u32 1000 ("milliseconds to wait")) -> (x*y=w1902:dbl)
                  n1502 = Wait (ms)(milliseconds to wait=w1902) -> ()  [unwired: 1 out]
                  n1503 = call "AVS48 Single Scan.vi"() -> ()  [unwired: 12 in]
                }
                frame "AVS Emulation" {
                  n1504 = local read "I_in"() -> (w1908:dbl[])
                  n1505 = Multiply(x=w1911, y=u32 1000 ("milliseconds to wait")) -> (x*y=w1920:dbl)
                  n1506 = Wait (ms)(milliseconds to wait=w1920) -> ()  [unwired: 1 out]
                  n1507 = Index Array(array=w1908, index=3) -> ()  [unwired: 1 out]
                  n1508 = property on="I" class="Arr (strict)"() -> ("Value"=w1919:dbl[])  [unwired: 2 in, 2 out]
                  n1509 = Multiply(x=1000.0, y=w1919) -> (x*y=w1914:dbl[])
                  n1510 = Index Array(array=w1914, index #1=2 ("index"), index #2=3 ("index")) -> (element #1=w1915:dbl, element #2=w1916:dbl)
                  n1511 = call "AVS Emulate.vi"("I_mc"=w1916, "I_still"=w1915, "Sampling time"=w1911) -> ("R"=w1910:dbl[])  [unwired: 1 out]
                }
                frame "Impedance Bridge" {
                  n1512 = local read "Bridge status"() -> (w1924:errorcluster)
                  n1513 = local read "zDll"() -> (w1933:path)
                  n1514 = call "Read Data from Single Channel.vi"("error in (no error)"=w1924, "zDll"=w1933) -> ("error out"=w1931:errorcluster, "Value"=w1928:dbl, "Scan parameters/Error string"=→"zBridge params/Error":string, "Set number"=w1929:u8, "Error code"=→"Error code":u8, "Unit"=→"Unit":string, "Scan Parameters"=→"Scan Parameters":cluster{string, "Freq":dbl, "V_exc":dbl})  [unwired: 3 in]
                  "zBridge set nr." <- w1929
                  n1515 = Replace Array Subset(array="Data array", new element=w1928, index=w1929) -> (w1923:dbl[])
                }
                frame "Disabled", Default {
                }
              }
              "Bridge status" <- w1862
              n1516 = property on="Delay" class="DigNum (strict)"() -> ("Value"=w1870:u32)  [unwired: 2 in, 2 out]
              n1517 = property on="Data array" class="Arr (strict)"("Val(Sgnl)"=w1860) -> ()  [unwired: 2 in, 2 out]
              n1518 = property on="Ranges" class="Clust (strict)"("Val(Sgnl)"=w1854) -> ()  [unwired: 2 in, 2 out]
              n1519 = Multiply(x=u32 1000, y=w1870) -> (x*y=w1869:u32)
              n1520 = Wait (ms)(milliseconds to wait=w1869) -> ()  [unwired: 1 out]
            }
            frame True {
            }
          }
        }
        n1521 = while {
          stop <- w1938 stop-if-true
          (unwired) errorcluster {"status"=FALSE, "code"=0, "source"=""} ("Value")
          # "Current source control"
          n1522 = property on="CS status" class="Clust (strict)"() -> ("Value"=w1937:errorcluster)  [unwired: 2 in, 2 out]
          n1523 = stacked-sequence {
            seq-local: [w1966 _ _ _] -> [_ w1975 _ _]
            seq-local: [w1965 _ _ _] -> [_ w1974 _ _]
            seq-local: [_ w1975 _ _] -> [_ _ w1985 _]
            seq-local: [_ w1973 _ _] -> [_ _ w1984 _]
            tunnel: w1937 -> [w1964 _ _ _]
            frame #0 {
              # "Write 0 instead of the actual \ncurrent value to log if there \nis no current flow."
              # "Read current CS status"
              n1524 = local read "CS ref"() -> (w1954:refnum<class "CS.lvclass">)
              n1525 = property on="TCS port" class="Ring (strict)" props=["Value"]() -> ()  [unwired: 2 in, 3 out]
              n1526 = call-dynamic "Read.vi"("CS in"=w1954, "error in (no error)"=w1964, "Optional"=FALSE) -> ("CS out"=w1966:refnum<class "CS.lvclass">, "I0"=w1957:T58, "I1"=w1958:T58, "I2"=w1959:T58, "I3"=w1960:T58, "error out"=w1965:errorcluster)  [unwired: 11 in]
              n1527 = Unbundle By Name(w1957) -> ("Current (string)"=w1952:string, "I?"=w1951:bool)
              n1528 = Unbundle By Name(w1958) -> ("Current (string)"=w1967:string, "I?"=w1950:bool)
              "Current1flow" <- w1950
              n1529 = Unbundle By Name(w1959) -> ("Current (string)"=w1955:string, "I?"=w1949:bool)
              n1530 = Unbundle By Name(w1960) -> ("Current (string)"=w1968:string, "I?"=w1948:bool)
              n1531 = call "CS Data Converter.vi"("CS Data"=w1957) -> ("CS Indicator"=→"I0":T59)
              n1532 = call "CS Data Converter.vi"("CS Data"=w1958) -> ("CS Indicator"=→"I1":T59)
              n1533 = call "CS Data Converter.vi"("CS Data"=w1959) -> ("CS Indicator"=→"I2":T59)
              n1534 = call "CS Data Converter.vi"("CS Data"=w1960) -> ("CS Indicator"=→"I3":T59)
              n1535 = Fract/Exp String To Number(string=w1952) -> (number=w1956:dbl)  [unwired: 3 in, 1 out]
              n1536 = Fract/Exp String To Number(string=w1967) -> (number=w1963:dbl)  [unwired: 3 in, 1 out]
              n1537 = Fract/Exp String To Number(string=w1955) -> (number=w1962:dbl)  [unwired: 3 in, 1 out]
              n1538 = Fract/Exp String To Number(string=w1968) -> (number=w1961:dbl)  [unwired: 3 in, 1 out]
              n1539 = Build Array(w1951, w1950, w1949, w1948) -> (w1947:bool[])
              n1540 = Not(x=w1947) -> (.not. x?=w1943:bool[])
              n1541 = Build Array(w1956, w1963, w1962, w1961) -> (w1946:dbl[])
              "I" <- w1946
              n1542 = for {
                tunnel: w1943 -> [w1972] mode=indexing
                tunnel: w1946 -> [w1971] mode=indexing
                tunnel: dbl[] [0.0, 0.0, 0.0, 0.0] ("t") -> [w1970] mode=indexing
                tunnel: [w1969] -> w1944 mode=indexing
                n1543 = Select(t=w1970, s=w1972, f=w1971) -> (s? t:f=w1969:dbl)
              }
              "Actual I" <- w1944
            }
            frame #1 {
              n1544 = Wait (ms)(milliseconds to wait=100) -> ()  [unwired: 1 out]
              n1545 = call <vilib>:"Clear Errors.vi"("error in (no error)"=w1974) -> ("error out"=w1973:errorcluster)  [unwired: 6 in]
            }
            frame #2 {
              # "Only send data to CS if\nnew value was entered"
              # "Set CS status"
              n1546 = call "CS OnOff & Gated and Current & Range.vi"("I in"="C_I0") -> ("OnOff & Gated"=w1996:T60, "Current & Range"=w1981:T61, "I out"=w1989:T62)  [unwired: 2 in]
              n1547 = call "CS OnOff & Gated and Current & Range.vi"("I in"="C_I1") -> ("OnOff & Gated"=w1995:T60, "Current & Range"=w1980:T61, "I out"=w1986:T62)  [unwired: 2 in]
              n1548 = call "CS OnOff & Gated and Current & Range.vi"("I in"="C_I2") -> ("OnOff & Gated"=w1992:T60, "Current & Range"=w1979:T61, "I out"=w1987:T62)  [unwired: 2 in]
              n1549 = call "CS OnOff & Gated and Current & Range.vi"("I in"="C_I3") -> ("OnOff & Gated"=w1991:T60, "Current & Range"=w1978:T61, "I out"=w1988:T62)  [unwired: 2 in]
              n1550 = local write "C_I0"(w1989) -> ()
              n1551 = local write "C_I1"(w1986) -> ()
              n1552 = local write "C_I2"(w1987) -> ()
              n1553 = local write "C_I3"(w1988) -> ()
              n1554 = local read "I_in"() -> (w1977:dbl[])
              n1555 = Equal To 0?(x="CS Mode") -> (x = 0?=w1982:bool)
              n1556 = call "CS_set_channels.vi"("CS in"=w1985, "Current & Range0"=w1981, "Current & Range1"=w1980, "Current & Range 2"=w1979, "Current & Range3"=w1978, "error out"=w1984, "I 2"=w1977, "Auto?"=w1982) -> ("CS.lvclass out"=w2001:refnum<class "CS.lvclass">, "Current Changed?"=w1998:bool, "error out 2"=w2002:errorcluster)  [unwired: 9 in]
              n1557 = call-dynamic "Set Mode.vi"("CS.lvclass in"=w2001, "On&G 0"=w1996, "On&G 1"=w1995, "On&G 2"=w1992, "On&G 3"=w1991, "error in (no error)"=w2002) -> ("CS.lvclass out"=w1999:refnum<class "CS.lvclass">, "error out"=w2000:errorcluster)  [unwired: 12 in]
              n1558 = case shown="False" w1998 {
                selector: w1998 -> [_ w2003]
                frame False {
                }
                frame True {
                  n1559 = property on="Currents changed" class="Bool (strict)"("Val(Sgnl)"=w2003) -> ()  [unwired: 2 in, 2 out]
                }
              }
              n1560 = local write "CS ref"(w1999) -> ()
              n1561 = property on="CS status" class="Clust (strict)"("Value"=w2000) -> ()  [unwired: 2 in, 2 out]
            }
            frame #3 {
              n1562 = Wait (ms)(milliseconds to wait=100) -> ()  [unwired: 1 out]
            }
          }
          n1563 = local read "Stop"() -> (w1938:bool)
        }
        n1564 = while {
          stop <- w1843 stop-if-true
          # "zBridge status read-out"
          n1565 = property on="AVS type" class="Enum (strict)"() -> ("Value"=w1841:T35)  [unwired: 2 in, 2 out]
          n1566 = case shown="\"Impedance Bridge\"" w1841 {
            frame Default {
            }
            frame "Impedance Bridge" {
              n1567 = local read "Bridge status"() -> (w1848:errorcluster)
              n1568 = local read "zDll"() -> (w1849:path)
              n1569 = call "ScanStatus.vi"("error in (no error)"=w1848, "zDll"=w1849) -> ("error out"=w1847:errorcluster, "Status"=w1845:i32, "Channel"=w1846:i32)  [unwired: 7 in]
              n1570 = local write "Bridge status"(w1847) -> ()
              n1571 = call "zBridge Format Status.vi"("Status"=w1845, "Channel"=w1846) -> ("Status"=→"Status":T63, "Active channel"=→"Active channel":T64)  [unwired: 2 in]
            }
          }
          n1572 = Wait (ms)(milliseconds to wait=u32 200) -> ()  [unwired: 1 out]
          n1573 = local read "Stop"() -> (w1843:bool)
        }
      }
    }
    n1574 = local read "Stop"() -> (w1837:bool)
  }
  n1575 = disable-structure shown="Disabled" {
    frame Disabled {
      w2009 = string[] ["Paste Data from Clipboard"] ("item names")
      (unwired) enum32{"Page 1"}."Page 1" ("Tab Control 4")
      n1576 = local read "Scan Parameters"() -> ()  [unwired: 1 out]
      n1577 = local read "Active"() -> ()  [unwired: 1 in]
      n1578 = property class="XYGraph (strict)" props=["YScale", "Mapping Mode"]() -> ()  [unwired: 2 in, 3 out]
      n1579 = Insert Menu Items(4:4, 7:w2009, 8:w2009) -> ()  [unwired: 3 in, 3 out]
      n1580 = property on="ON" class="Boolean (strict)"() -> ("Value"=w2016:bool)  [unwired: 2 in, 2 out]
      n1581 = control-ref of="Active"() -> ()  [unwired: 1 out]
      n1582 = Exclusive Or(1:w2016, 2:TRUE ("x")) -> (0:w2015:bool)
      n1583 = property on="Toggle ON/OFF" class="Bool (strict)"("Value"=w2015) -> ()  [unwired: 2 in, 2 out]
      n1584 = control-ref of="I_list"() -> (w2011:refnum<vi>)
      n1585 = property on="ResetPIDloop" class="TypRef (strict)"() -> ("Value"=w2021:refnum<user-event>)  [unwired: 2 in, 2 out]
      n1586 = property class="Arr (strict)"(reference=w2011) -> ("Index Values"=w2012:u32[])  [unwired: 1 in, 2 out]
      n1587 = Generate User Event(user event=w2021, event data cluster="" ("event data")) -> ()  [unwired: 2 in, 2 out]
      n1588 = Index Array(array=w2012) -> (element=w2013:u32)  [unwired: 1 in]
      n1589 = property on="Tab Control 2" class="TabCtl (strict)"() -> ("Pages"=w2017:refnum<vi>[])  [unwired: 2 in, 2 out]
      n1590 = property on="I_list_idx" class="DigNum (strict)"("Val(Sgnl)"=w2013) -> ()  [unwired: 2 in, 2 out]
      n1591 = Index Array(array=w2017, index=1) -> (element=w2018:refnum<vi>)
      n1592 = Generate User Event(event data cluster="" ("event data")) -> ()  [unwired: 3 in, 2 out]
      n1593 = property class="Page"(reference=w2018, "PageVis"=TRUE ("Page Visible")) -> ()  [unwired: 1 in, 2 out]
      n1594 = local read "Error"() -> ()  [unwired: 1 out]
      n1595 = local read "Int"() -> ()  [unwired: 1 out]
      n1596 = local read item#-1() -> ()  [unwired: 1 out]
      n1597 = Initialize Array(0.0 ("element"), 4 ("dimension size")) -> (w2005:dbl[])
      n1598 = call <userlib>:"MGI Get Slope at Point.vi"() -> ()  [unwired: 11 in, 1 out]
      n1599 = local write "I_in"(w2005) -> ()
      n1600 = call "Write To Spreadsheet File (string) w Error.vi"() -> ()  [unwired: 10 in, 2 out]
    }
    frame Enabled {
    }
  }
  n1601 = control-ref of="Automode Settings 2"() -> ()  [unwired: 1 out]
  n1602 = property on="I3_SP" class="DigNum (strict)" props=["Value"]() -> ()  [unwired: 2 in, 3 out]
